vi "DPC LabView Controller.vi"() -> ()   [LabVIEW 2024]
doc: "This example program utilizes almost all VI's included in the AALBORG DPCM LabView Driver Library. In addition to the extended program example it provides access to the PI data Waveform Chart, User Defined Gas Mixture, Alarm Events and Process Information data logging settings and features of the DPM and DPC instruments. \nIf you have questions regarding VI's used in this example please refer to the \"AALBORG DPCM LabView Driver Library\" Manual (available on the AALBORG website and included in this driver library). If you still have questions please contact AALBORG at 845-770-3000 or info@aalborg.com"
uses:
  Examples/DPCM LabView Driver 2020_1v1/SubVI/Utilities/Control 1.ctl
  <vilib>/Utility/error.llb/Trim Whitespace One-Sided.vi
  Examples/DPCM LabView Driver 2020_1v1/SubVI/Utilities/Global.vi
panel:
  out "error out":errorcluster
  in  "Read Valve Output":bool
  in  "Read Register":bool
  out "Register Value":string
  in  "Reg. to read":u16 max=413
  in  "Log Register Values":bool
  out "Total GM:":u16
  in  "Gas mixture input":T1={"Ratio % 1"=0.0, "Enable # 1"=FALSE, "Ratio % 2"=0.0, "Enable # 2"=FALSE, "Ratio % 3"=0.0, "Enable # 3"=FALSE, "Ratio % 4"=0.0, "Enable # 4"=FALSE, "Ratio % 5"=0.0, "Enable # 5"=FALSE, "Mixture Gas 1"=0, "Mixture Gas 2"=0, "Mixture Gas 3"=0, "Mixture Gas 4"=0, "Mixture Gas 5"=0, "Create Mixture"=FALSE, "Mix. #"=200, "Mix. name"="MyMix1", "Completion\ntext"="", "Delete Mixture"=FALSE} caption="User Defined Gas Mixture input" {"Mix. #" min=200 max=219 step=1; "Mixture Gas 5" items=["Air", "Argon", "Carbon Dioxide", "Nitrogen", "Oxygen", "Helium", "Carbon Monoxide", "Ethylene", "Ethane", "n-Butane", "i-Butane", "Propane", "Deuterium", "Hydrogen", "Nitrous Oxide", "Methane", "Neon", "Krypton", "Sulfur Hexafluoride", "Xenon", "Acetylene", "25CO2/75Ar", "10CO2/90Ar", "8CO2/92Ar", "2CO2/98Ar", "75CO2/25Ar", "75He/25Ar", "25He/75Ar", "He A1025", "StargonCS", "95Ar/5CH4"]; "Mixture Gas 4" items=["Air", "Argon", "Carbon Dioxide", "Nitrogen", "Oxygen", "Helium", "Carbon Monoxide", "Ethylene", "Ethane", "n-Butane", "i-Butane", "Propane", "Deuterium", "Hydrogen", "Nitrous Oxide", "Methane", "Neon", "Krypton", "Sulfur Hexafluoride", "Xenon", "Acetylene", "25CO2/75Ar", "10CO2/90Ar", "8CO2/92Ar", "2CO2/98Ar", "75CO2/25Ar", "75He/25Ar", "25He/75Ar", "He A1025", "StargonCS", "95Ar/5CH4"]; "Mixture Gas 3" items=["Air", "Argon", "Carbon Dioxide", "Nitrogen", "Oxygen", "Helium", "Carbon Monoxide", "Ethylene", "Ethane", "n-Butane", "i-Butane", "Propane", "Deuterium", "Hydrogen", "Nitrous Oxide", "Methane", "Neon", "Krypton", "Sulfur Hexafluoride", "Xenon", "Acetylene", "25CO2/75Ar", "10CO2/90Ar", "8CO2/92Ar", "2CO2/98Ar", "75CO2/25Ar", "75He/25Ar", "25He/75Ar", "He A1025", "StargonCS", "95Ar/5CH4"]; "Mixture Gas 2" items=["Air", "Argon", "Carbon Dioxide", "Nitrogen", "Oxygen", "Helium", "Carbon Monoxide", "Ethylene", "Ethane", "n-Butane", "i-Butane", "Propane", "Deuterium", "Hydrogen", "Nitrous Oxide", "Methane", "Neon", "Krypton", "Sulfur Hexafluoride", "Xenon", "Acetylene", "25CO2/75Ar", "10CO2/90Ar", "8CO2/92Ar", "2CO2/98Ar", "75CO2/25Ar", "75He/25Ar", "25He/75Ar", "He A1025", "StargonCS", "95Ar/5CH4"]; "Mixture Gas 1" items=["Air", "Argon", "Carbon Dioxide", "Nitrogen", "Oxygen", "Helium", "Carbon Monoxide", "Ethylene", "Ethane", "n-Butane", "i-Butane", "Propane", "Deuterium", "Hydrogen", "Nitrous Oxide", "Methane", "Neon", "Krypton", "Sulfur Hexafluoride", "Xenon", "Acetylene", "25CO2/75Ar", "10CO2/90Ar", "8CO2/92Ar", "2CO2/98Ar", "75CO2/25Ar", "75He/25Ar", "25He/75Ar", "He A1025", "StargonCS", "95Ar/5CH4"]; "Ratio % 1" min=0.0 max=100.0 step=0.01; "Ratio % 2" min=0.0 max=100.0 step=0.01; "Ratio % 3" min=0.0 max=100.0 step=0.01; "Ratio % 4" min=0.0 max=100.0 step=0.01; "Ratio % 5" min=0.0 max=100.0 step=0.01}
  in  "AE Reset":bool
  in  "Alarm Events":T2={"AE Enable 0"=TRUE, "AE Enable 1"=TRUE, "AE Enable 2"=TRUE, "AE Enable 3"=TRUE, "AE Enable 4"=TRUE, "AE Enable 5"=TRUE, "AE Enable 6"=TRUE, "AE Enable 7"=TRUE, "AE Enable 8"=TRUE, "AE Enable 9"=TRUE, "AE Enable 10"=TRUE, "AE Enable 11"=TRUE, "AE Enable 12"=TRUE, "AE Enable 13"=TRUE, "AE Latch 0"=TRUE, "AE Latch 1"=TRUE, "AE Latch 2"=TRUE, "AE Latch 3"=TRUE, "AE Latch 4"=TRUE, "AE Latch 5"=TRUE, "AE Latch 6"=TRUE, "AE Latch 7"=TRUE, "AE Latch 8"=TRUE, "AE Latch 9"=TRUE, "AE Latch 10"=TRUE, "AE Latch 11"=TRUE, "AE Latch 12"=TRUE, "AE Latch 13"=TRUE, "AE Indicator 0"=FALSE, "AE Indicator 1"=FALSE, "AE Indicator 2"=FALSE, "AE Indicator 3"=FALSE, "AE Indicator 4"=FALSE, "AE Indicator 5"=FALSE, "AE Indicator 6"=FALSE, "AE Indicator 7"=FALSE, "AE Indicator 8"=FALSE, "AE Indicator 9"=FALSE, "AE Indicator 10"=FALSE, "AE Indicator 11"=FALSE, "AE Indicator 12"=FALSE, "AE Indicator 13"=FALSE}
  in  "PI Logging Options":T3={"Set Point"=TRUE, "Valve Counts"=FALSE, "Mass Flow"=TRUE, "Volumetric Flow"=TRUE, "Totalizer#1"=TRUE, "Totalizer#2"=TRUE, "Gas Temperature"=TRUE, "Gas Pressure"=TRUE, "Flow Alarm"=TRUE, "Temp. Alarm"=TRUE, "Pressure Alarm"=TRUE, "Alarm Events"=FALSE, "Diagnostic Events"=FALSE, "Selected Gas"=FALSE, "Log Data"=FALSE, "Include Header"=TRUE}
  in  "Chart: Adjust Scale":bool
  in  "Chart: AutoScale Chart":bool
  in  "Chart: Enable Graphic":bool
  in  "Chart: Pressure":bool
  in  "Chart: Temperature":bool
  in  "Chart: Set Point":bool
  in  "Chart: Volum Flow":bool
  in  "Chart: Mass Flow":bool
  out "Chart":cluster{dbl, dbl, dbl, dbl, dbl}(graph)={50.0, 50.24, 50.0, 23.8, 14.76}
  out "Wait Message":cluster{"Boolean":bool}
  in  "stop":bool
  out "Process Information":T4
  in  "Set Point Options":T5 {"Setpoint Value" min=0.0 max=0.0}
  in  "Analog Input":string(combo)
  in  "Analog Output":string(combo)
  in  "SS Relay Assignment":string(combo)
  in  "Measuring Units":T6
  in  "Update Time  [ms]":u32=150 min=100
  out "Measurem.\nper second":dbl format="%#.3g"
  in  "Selected Gas":string(combo)
  in  "Alarms":enum32{"Flow ", "Temp. ", "Pressure "}(tab)
  in  "Flow Alarm":T7 {"Power Up Delay [s]" min=0.0 max=3600.0 format="%#.0f"; "Action Delay [s]" min=0.0 max=3600.0 format="%#.0f"; "Low Alarm Limit" min=0.0 max=125.0 format="%#.1f"; "High Alarm Limit" min=0.0 max=125.0 format="%#.1f"}
  in  "Temperature Alarm":T8={"Enabled"=FALSE, "Status:"="", "High Temp. Alarm Limit"=253.1, "Low Temp. Alarm Limit"=0.0, "Temp. Alarm Latch"=FALSE, "Action Delay [s]"=0.0, "Power Up Delay [s]"=0.0} {"Power Up Delay [s]" min=0.0 max=3600.0 format="%#.0f"; "Action Delay [s]" min=0.0 max=3600.0 format="%#.0f"; "Low Temp. Alarm Limit" min=0.0 max=125.0 format="%#.1f"; "High Temp. Alarm Limit" min=253.1 max=343.1 format="%#.1f"}
  in  "Pressure Alarm":T9={"Enabled"=FALSE, "Status:"="", "High Pressure Alarm Limit"=253.1, "Low Pressure Alarm Limit"=0.0, "Pressure Alarm Latch"=FALSE, "Action Delay [s]"=0.0, "Power Up Delay [s]"=0.0} {"Power Up Delay [s]" min=0.0 max=3600.0 format="%#.0f"; "Action Delay [s]" min=0.0 max=3600.0 format="%#.0f"; "Low Pressure Alarm Limit" min=0.0 max=125.0 format="%#.1f"; "High Pressure Alarm Limit" min=253.1 max=343.1 format="%#.1f"}
  in  "Tab Control":T10(tab)
  in  "Totalizer #1 Options":T11 {"Power Up Delay [seconds]" min=0.0 max=3600.0 format="%#.0f"; "Auto Reset Delay [seconds]" min=0.0 max=3600.0 format="%#.0f"; "Current Volume" format="%#.2f"; "Action Volume" format="%#.2f"; "Start @ Flow" min=0.0 max=100.0 format="%#.2f"}
  in  "Totalizer #2 Options":T12 {"Current Volume" format="%#.2f"; "Action Volume" format="%#.2f"; "Start @ Flow" min=0.0 max=100.0 format="%#.1f"; "Power Up Delay [Seconds]" min=0.0 max=3600.0 format="%#.0f"; "Auto Reset Delay [Seconds]" min=0.0 max=3600.0 format="%#.0f"}
  in  "Pulse Output Options":T13={"Enabled"=FALSE, "Start @ Flow Rate"=0.0, "Unit Per Pulse"=0.0, "Pulse Unit"="", "Pulse Active Time [ms]"=25.0} {"Pulse Active Time [ms]" min=25.0 max=3276.0 format="%#.0f"; "Unit Per Pulse" format="%#.2f"; "Start @ Flow Rate" min=0.0 max=100.0 format="%#.1f"}
  out "Device Information":T14
  in  "Serial Configuration":T16={"Baud Rate"=9600, "Serial Port #"="COM1", "RS-485"=FALSE, " Address"=17} {"Address" min=1 format="%2x"; "Baud Rate" items=["300"=300, "600"=600, "1200"=1200, "2400"=2400, "4800"=4800, "9600"=9600, "19200"=19200, "38400"=38400]}
  # "Timing Options"
  # "(will require longer update time)"
  # "Before changing Analog Input or Output mode make sure proper equipment is connected to the corresponding pins on the interface connector!"
  # "E/D"
  # "Latch"
  # "Register Values"
  # "AALBORG INSTRUMENTS"
  # "& CONTROLS INC."
  # "Possible Issues\n• When communicating with instruments over RS-485 interface and \"Read Valve Output\" check box is selected some times it is possible to get \"Communication Error\" message when low \"Baud Rate\" settings are selected. In this case use 19200 or higher \"Baud Rate\" settings to be able to faster transfer long data frames to and from the instrument.\n\n• Do not use \"Update Time\" settings with values below 50 ms. Doing so especially with low \"Baud Rate\" settings may result in communication error."
  # "High Flow Alarm"
  # "Low Flow Alarm"
  # "Flow between H & L"
  # "Totalizer#1 > Limit"
  # "Totalizer#2 > Limit"
  # "High Press. Alarm"
  # "Low Pressure Alarm"
  # "Press. between H&L"
  # "High Temp. Alarm"
  # "Low Temp. Alarm"
  # "Temp. Between H&L"
  # "Pulse Output > Limit"
  # "Password Event"
  # "Power On Event"
  # "Altering options will start a new log"
  # "(The data file will be open in the folder containing the VI)"
  # "Populating VI with instrument information. Standby..."
  # "Alarm"
  # "%FS"
  # "%FS"
  # "K  [253.1 - 343.1K]"
  # "K [253.0 - 343.0K]"
  # "PSIA  [0.1-100 PSIA]"
  # "PSIA [0.0-99.9 PSIA]"
  # "%FS"
  # "%FS"
  # "%FS"
  # "/Pulse"
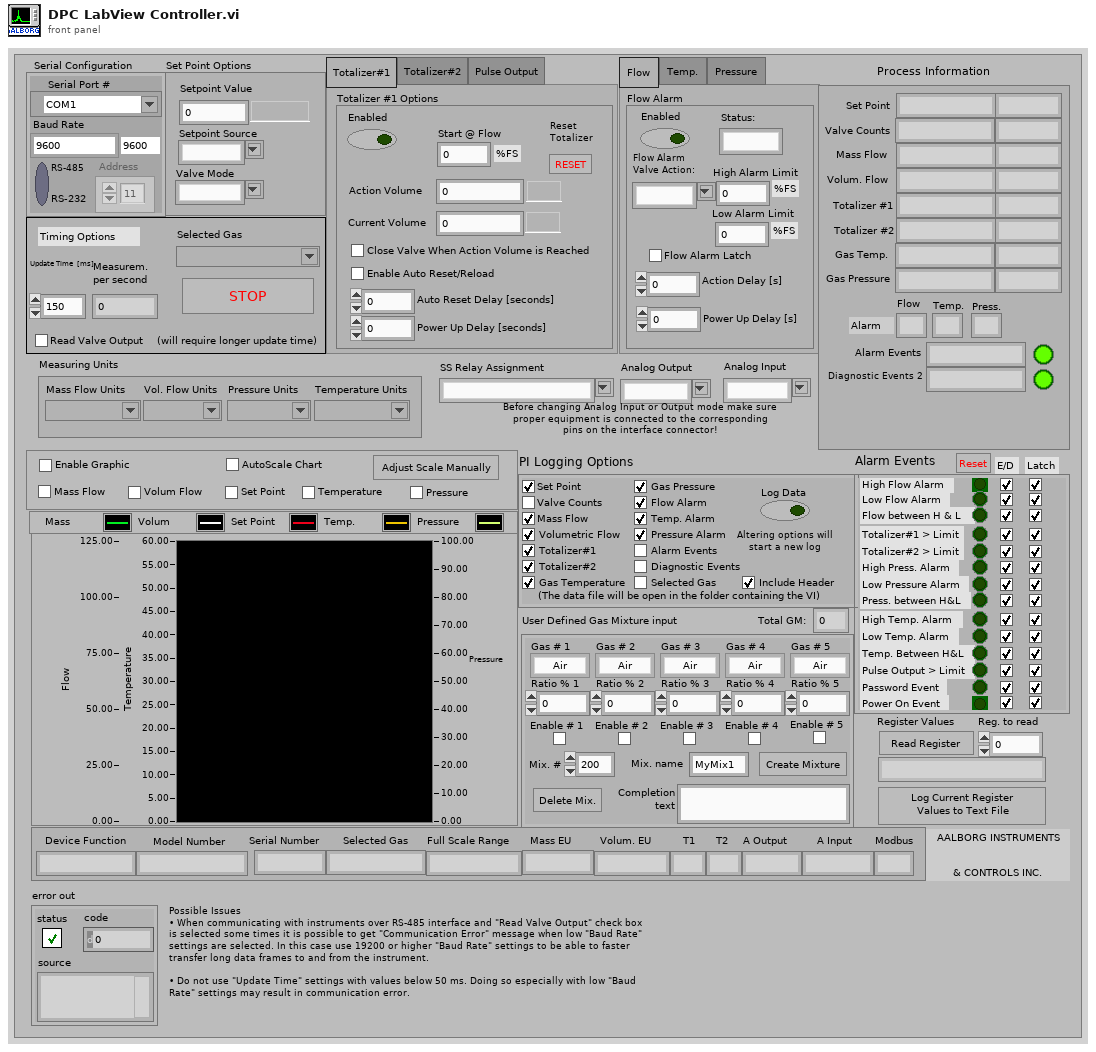
[diagram p1: front panel]
types:
  T1 = cluster{"Ratio % 1":dbl, "Enable # 1":bool, "Ratio % 2":dbl, "Enable # 2":bool, "Ratio % 3":dbl, "Enable # 3":bool, "Ratio % 4":dbl, "Enable # 4":bool, "Ratio % 5":dbl, "Enable # 5":bool, "Mixture Gas 1":u16, "Mixture Gas 2":u16, "Mixture Gas 3":u16, "Mixture Gas 4":u16, "Mixture Gas 5":u16, "Create Mixture":bool, "Mix. #":u16, "Mix. name":string, "Completion\ntext":string, "Delete Mixture":bool}
  T2 = cluster{"AE Enable 0":bool, "AE Enable 1":bool, "AE Enable 2":bool, "AE Enable 3":bool, "AE Enable 4":bool, "AE Enable 5":bool, "AE Enable 6":bool, "AE Enable 7":bool, "AE Enable 8":bool, "AE Enable 9":bool, "AE Enable 10":bool, "AE Enable 11":bool, "AE Enable 12":bool, "AE Enable 13":bool, "AE Latch 0":bool, "AE Latch 1":bool, "AE Latch 2":bool, "AE Latch 3":bool, "AE Latch 4":bool, "AE Latch 5":bool, "AE Latch 6":bool, "AE Latch 7":bool, "AE Latch 8":bool, "AE Latch 9":bool, "AE Latch 10":bool, "AE Latch 11":bool, "AE Latch 12":bool, "AE Latch 13":bool, "AE Indicator 0":bool, "AE Indicator 1":bool, "AE Indicator 2":bool, "AE Indicator 3":bool, "AE Indicator 4":bool, "AE Indicator 5":bool, "AE Indicator 6":bool, "AE Indicator 7":bool, "AE Indicator 8":bool, "AE Indicator 9":bool, "AE Indicator 10":bool, "AE Indicator 11":bool, "AE Indicator 12":bool, "AE Indicator 13":bool}
  T3 = cluster{"Set Point":bool, "Valve Counts":bool, "Mass Flow":bool, "Volumetric Flow":bool, "Totalizer#1":bool, "Totalizer#2":bool, "Gas Temperature":bool, "Gas Pressure":bool, "Flow Alarm":bool, "Temp. Alarm":bool, "Pressure Alarm":bool, "Alarm Events":bool, "Diagnostic Events":bool, "Selected Gas":bool, "Log Data":bool, "Include Header":bool}
  T4 = cluster{"Mass Flow":string, "Volum. Flow":string, "Totalizer #1":string, "Totalizer #2":string, "Gas Temp.":string, "Gas Pressure":string, "Flow":string, "Press.":string, "Temp.":string, "Alarm Events":string, "Diagnostic Events 2":string, "Set Point":string, "Valve Counts":string, "Alarm Ind":bool, "Diagnostic Ind":bool, "SP Units":string, "Valve Counts Units":string, "Mass Flow Units":string, "Vol Flow Units":string, "Total1 Vol Units":string, "Total2 Vol Units":string, "Gas Temp Units":string, "Gas Press Units":string}
  T5 = cluster{"Setpoint Value":dbl, "Mass Flow EU 2":string, "Setpoint Source":string, "Valve Mode":string}
  T6 = cluster{"Mass Flow Units":string, "Vol. Flow Units":string, "Pressure Units":string, "Temperature Units":string}
  T7 = cluster{"Enabled":bool, "Status:":string, "High Alarm Limit":dbl, "Low Alarm Limit":dbl, "Flow Alarm Latch":bool, "Action Delay [s]":dbl, "Power Up Delay [s]":dbl, "Flow Alarm Valve Action:":string}
  T8 = cluster{"Enabled":bool, "Status:":string, "High Temp. Alarm Limit":dbl, "Low Temp. Alarm Limit":dbl, "Temp. Alarm Latch":bool, "Action Delay [s]":dbl, "Power Up Delay [s]":dbl}
  T9 = cluster{"Enabled":bool, "Status:":string, "High Pressure Alarm Limit":dbl, "Low Pressure Alarm Limit":dbl, "Pressure Alarm Latch":bool, "Action Delay [s]":dbl, "Power Up Delay [s]":dbl}
  T10 = enum32{"Totalizer#1", "Totalizer#2", "Pulse Output"}
  T11 = cluster{"Enabled":bool, "Start @ Flow":dbl, "Action Volume":dbl, "Total EU 1":string, "Current Volume":dbl, "Total EU 2":string, "Close Valve When Action Volume is Reached":bool, "Enable Auto Reset/Reload":bool, "Auto Reset Delay [seconds]":dbl, "Power Up Delay [seconds] ":dbl, "Reset Totalizer":bool}
  T12 = cluster{"Enabled":bool, "Start @ Flow":dbl, "Action Volume":dbl, "Total EU 1":string, "Current Volume":dbl, "Total EU 2":string, "Close Valve When Action Volume is Reached":bool, "Enable Auto Reset/Reload":bool, "Auto Reset Delay [Seconds]":dbl, "Power Up Delay [Seconds] ":dbl, "Reset Totalizer":bool}
  T13 = cluster{"Enabled":bool, "Start @ Flow Rate":dbl, "Unit Per Pulse":dbl, "Pulse Unit":string, "Pulse Active Time [ms]":dbl}
  T14 = cluster{"Device Function":string, "Model Number":string, "Serial Number":string, "Selected Gas":string, "Full Scale Range":string, "Mass EU":string, "Volum. EU":string, "    T1 ":string, "   T2 ":string, "A Output":string, "A Input":string, "Modbus":string}
  T15 = typedef "Control 1.ctl" = u32
  T16 = cluster{"Baud Rate":T15, "Serial Port #":refnum<visa-resource-name>, "RS-485":bool, " Address":u8}
  T17 = cluster{"Mass Flow":bool, "Volum Flow":bool, "Set Point":bool, "Temperature":bool, "Pressure":bool, "AutoScale Chart":bool}
  T18 = cluster{"Enabled":string, "High Alarm Limit":string, "Low Alarm Limit":string, "Action Delay":string, "Latch Mode":string, "Power Up Delay":string}
  T19 = cluster{"Enabled":bool, "Start @ Flow":dbl, "Limit Volume":dbl, "Total EU 1":string, "Current Volume":dbl, "Total EU 2":string, "Close Valve When Limit Volume is Reached":bool, "Enable Auto Reset/Reload":bool, "Auto Reset Delay [Seconds]":dbl, "Power Up Delay [Seconds] ":dbl, "Reset Totalizer":bool}
  T20 = cluster{"Enabled":bool, "Start @ Flow":dbl, "Limit Volume":dbl, "Total EU 1":string, "Current Volume":dbl, "Total EU 2":string, "Close Valve When Limit Volume is Reached":bool, "Enable Auto Reset/Reload":bool, "Auto Reset Delay [seconds]":dbl, "Power Up Delay [seconds] ":dbl, "Reset Totalizer":bool}
  T21 = cluster{"Enabled":enum8{"Enabled", "Disabled", "Disabled and Grayed Out"}, "Disabled and Grayed Out":enum8{"Enabled", "Disabled", "Disabled and Grayed Out"}}
  T22 = enum16{"open", "replace", "create", "open or create", "replace or create", "replace or create with confirmation"}
  T23 = cluster{"Mass Flow":string, "Valve Counts":string, "Volumetric Flow":string, "Totalizer":string, "Temperature":string, "Pressure":string}
  T24 = cluster{"Gas # 1":u16, "Mix % 1":dbl, "Include # 1":bool, "Gas # 2":u16, "Mix % 2":dbl, "Include # 2":bool, "Gas # 3":u16, "Mix % 3":dbl, "Include # 3":bool, "Gas # 4":u16, "Mix % 4":dbl, "Include # 4":bool, "Gas # 5":u16, "Mix % 5":dbl, "Include # 5":bool}
  T25 = cluster{"Model Number":string, "Serial Number":string, "Gas Name":string, "FS Range":string, "Mass Flow EU":string, "Volumetric Flow EU":string, "Modbus":string, "Totalizer#1 Mode":string, "Totalizer#2 Mode":string, "Analog Output":string, "Pressure EU":string, "Temperature EU":string, "Device Function":string}
  T26 = enum8{"Enabled", "Disabled", "Disabled and Grayed Out"}
  T27 = typedef "LVComboBoxStrsAndValuesArrayTypeDef.ctl" = cluster{"String":string, "Value":string}[]
  T28 = cluster{"Setpoint Source Out":string, "Valve Mode Out":string, dbl}
  T29 = cluster{"Tot. Mode":string, "Start @ Flow":string, "Limit Volume":string, "Power Up Delay":string, "Auto Reset Mode":string, "Auto Reset Delay":string}
  T30 = cluster{"Enabled":string, "Start @ Flow":string, "Unit Per Pulse":string, "Pulse Active Time":string}
  T31 = cluster{"string array[0]":string, "string array[1]":string, "string array[2]":string, "string array[3]":string, "string array[4]":string, "string array[5]":string, "string array[6]":string, "string array[7]":string, "string array[8]":string, "string array[9]":string, "string array[10]":string}
  T32 = enum16{"Left Button", "Center Button", "Right Button", "Window Close"}
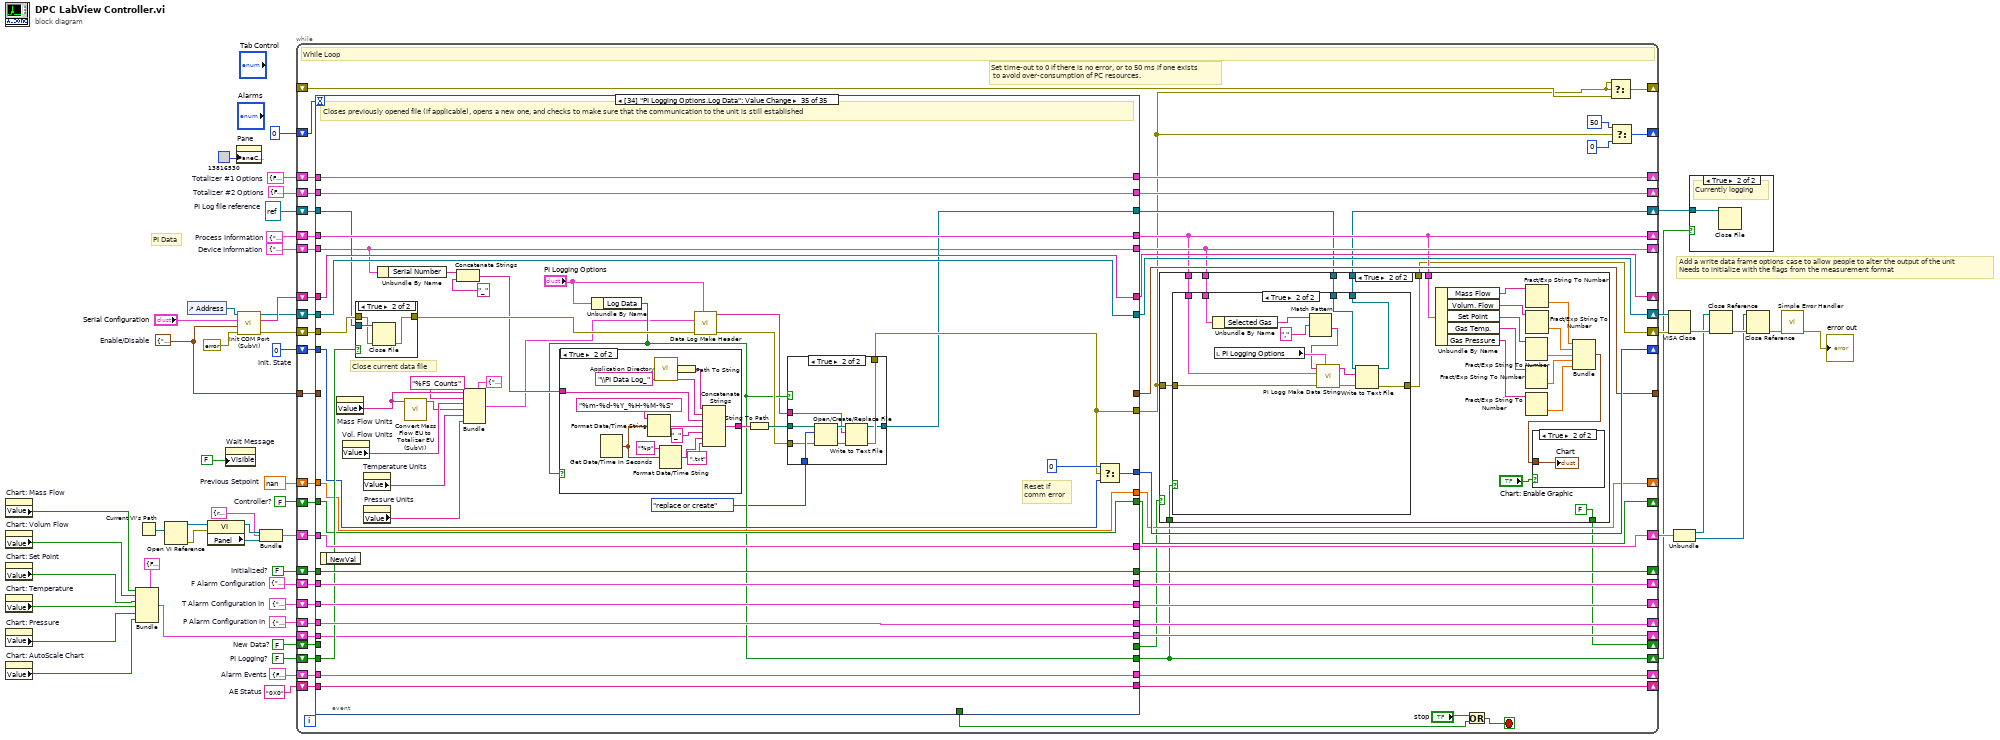
[diagram p0: block diagram]
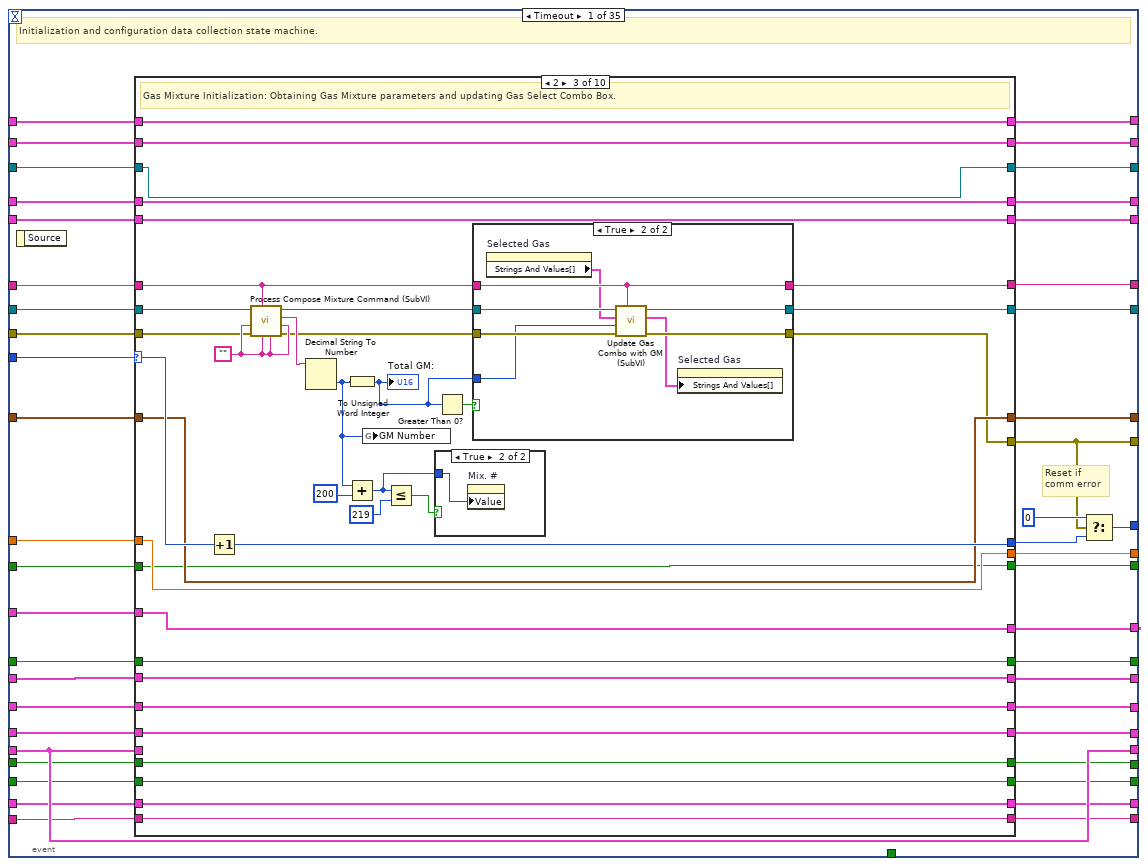
[diagram p6: hidden frame]
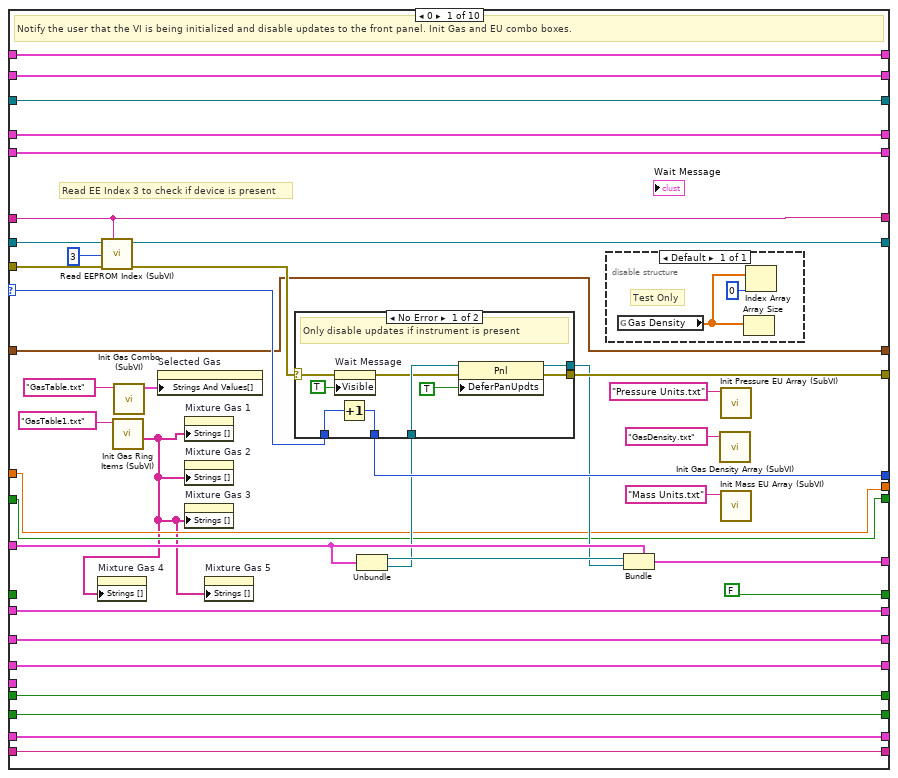
[diagram p7: hidden frame]
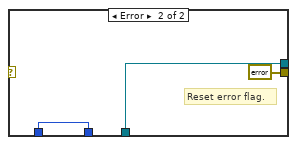
[diagram p8: hidden frame]
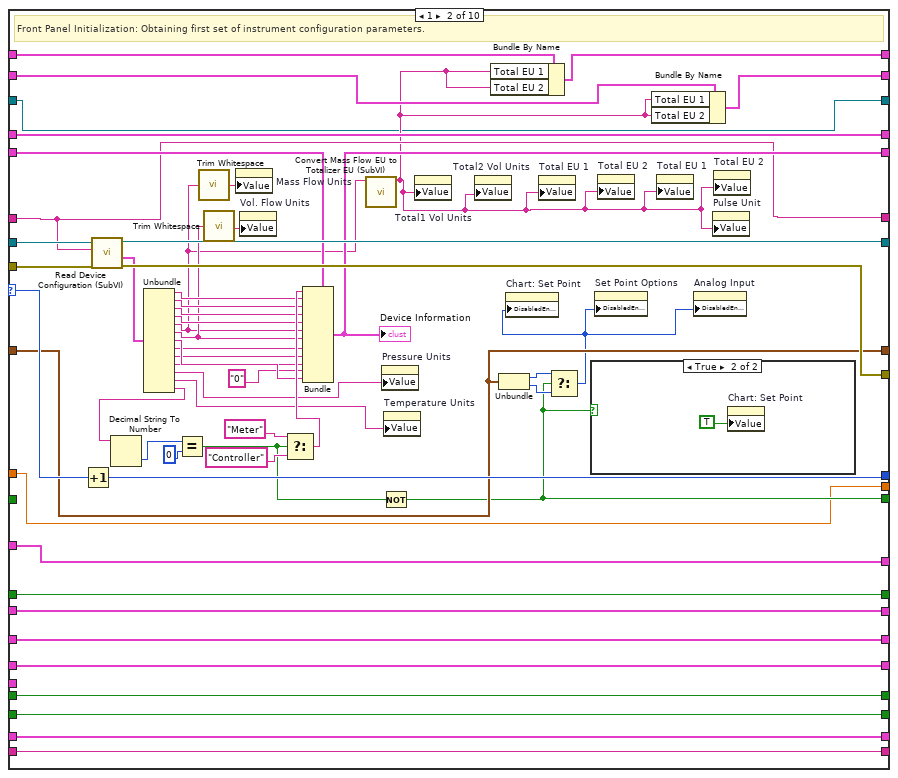
[diagram p9: hidden frame]
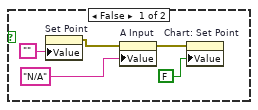
[diagram p10: hidden frame]
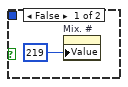
[diagram p11: hidden frame]
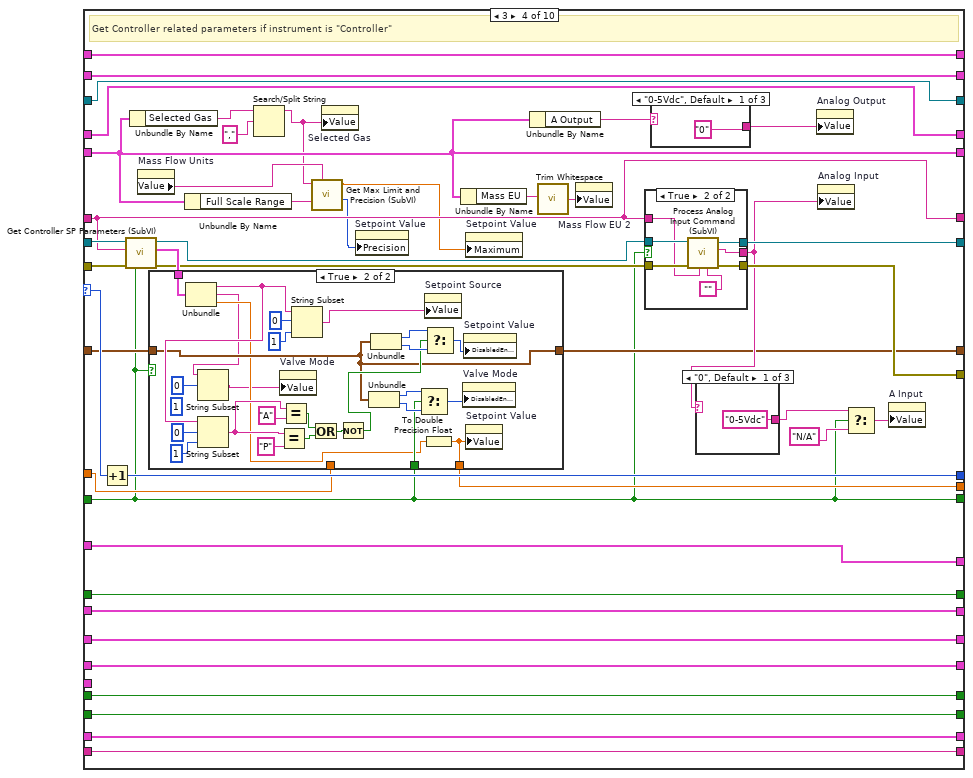
[diagram p13: hidden frame]
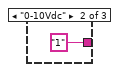
[diagram p15: hidden frame]
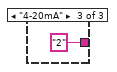
[diagram p16: hidden frame]
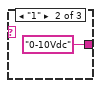
[diagram p17: hidden frame]
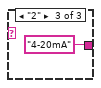
[diagram p18: hidden frame]
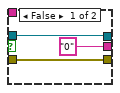
[diagram p19: hidden frame]
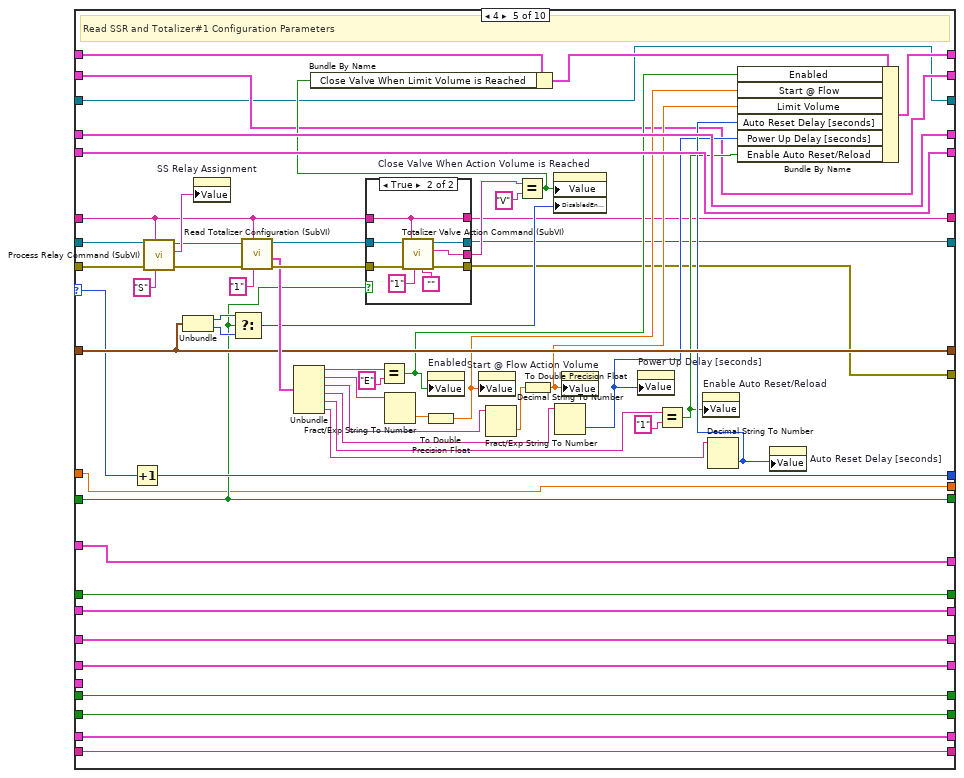
[diagram p20: hidden frame]
diagram:
  w2 = "0X0"  # AE Status
  w3 = T2 {"AE Enable 0"=FALSE, "AE Enable 1"=FALSE, "AE Enable 2"=FALSE, "AE Enable 3"=FALSE, "AE Enable 4"=FALSE, "AE Enable 5"=FALSE, "AE Enable 6"=FALSE, "AE Enable 7"=FALSE, "AE Enable 8"=FALSE, "AE Enable 9"=FALSE, "AE Enable 10"=FALSE, "AE Enable 11"=FALSE, "AE Enable 12"=FALSE, "AE Enable 13"=FALSE, "AE Latch 0"=FALSE, "AE Latch 1"=FALSE, "AE Latch 2"=FALSE, "AE Latch 3"=FALSE, "AE Latch 4"=FALSE, "AE Latch 5"=FALSE, "AE Latch 6"=FALSE, "AE Latch 7"=FALSE, "AE Latch 8"=FALSE, "AE Latch 9"=FALSE, "AE Latch 10"=FALSE, "AE Latch 11"=FALSE, "AE Latch 12"=FALSE, "AE Latch 13"=FALSE, "AE Indicator 0"=FALSE, "AE Indicator 1"=FALSE, "AE Indicator 2"=FALSE, "AE Indicator 3"=FALSE, "AE Indicator 4"=FALSE, "AE Indicator 5"=FALSE, "AE Indicator 6"=FALSE, "AE Indicator 7"=FALSE, "AE Indicator 8"=FALSE, "AE Indicator 9"=FALSE, "AE Indicator 10"=FALSE, "AE Indicator 11"=FALSE, "AE Indicator 12"=FALSE, "AE Indicator 13"=FALSE}  # Alarm Events
  w6 = FALSE  # PI Logging?
  w7 = refnum<file> refnum  # PI Log file reference
  w8 = FALSE  # New Data?
  w17 = T18 {"Enabled"="", "High Alarm Limit"="", "Low Alarm Limit"="", "Action Delay"="", "Latch Mode"="", "Power Up Delay"=""}  # P Alarm Configuration In
  w18 = T18 {"Enabled"="", "High Alarm Limit"="", "Low Alarm Limit"="", "Action Delay"="", "Latch Mode"="", "Power Up Delay"=""}  # T Alarm Configuration In
  w19 = T18 {"Enabled"="D", "High Alarm Limit"="54.00", "Low Alarm Limit"="7.00", "Action Delay"="1", "Latch Mode"="0", "Power Up Delay"="10"}  # F Alarm Configuration
  w20 = T19 {"Enabled"=FALSE, "Start @ Flow"=2.0, "Limit Volume"=0.0, "Total EU 1"="  %s  ", "Current Volume"=0.0, "Total EU 2"="  %s  ", "Close Valve When Limit Volume is Reached"=FALSE, "Enable Auto Reset/Reload"=FALSE, "Auto Reset Delay [Seconds]"=1.0, "Power Up Delay [Seconds] "=10.0, "Reset Totalizer"=FALSE}  # Totalizer #2 Options
  w21 = T20 {"Enabled"=FALSE, "Start @ Flow"=2.0, "Limit Volume"=0.0, "Total EU 1"="  %s  ", "Current Volume"=131.62, "Total EU 2"="  %s  ", "Close Valve When Limit Volume is Reached"=FALSE, "Enable Auto Reset/Reload"=FALSE, "Auto Reset Delay [seconds]"=2.0, "Power Up Delay [seconds] "=8.0, "Reset Totalizer"=FALSE}  # Totalizer #1 Options
  w22 = T14 {"Device Function"="Controller", "Model Number"="DPC17A-VAL6-A2", "Serial Number"="999001-2", "Selected Gas"="0,Air", "Full Scale Range"="0.00050 sl/min", "Mass EU"="%FS", "Volum. EU"=" %FS  ", "    T1 "="D", "   T2 "="D", "A Output"="0-5Vdc", "A Input"="0-5Vdc", "Modbus"="Yes"}  # Device Information
  w23 = T4 {"Mass Flow"="25.00", "Volum. Flow"="25.24", "Totalizer #1"="0.00", "Totalizer #2"="0.00", "Gas Temp."="23.72", "Gas Pressure"="14.68", "Flow"="D", "Press."="D", "Temp."="D", "Alarm Events"="0x0", "Diagnostic Events 2"="0x0", "Set Point"="  0.125", "Valve Counts"="N/A", "Alarm Ind"=FALSE, "Diagnostic Ind"=FALSE, "SP Units"="", "Valve Counts Units"="Counts", "Mass Flow Units"="", "Vol Flow Units"="", "Total1 Vol Units"="%s", "Total2 Vol Units"="%s", "Gas Temp Units"="C", "Gas Press Units"="PSIA"}  # Process Information
  w25 = nan  # Previous Setpoint
  w38 = FALSE  # Controller?
  w39 = FALSE  # Initialized?
  w47 = 0  # Init. State
  w28 = T21 {"Enabled"=enum."Enabled", "Disabled and Grayed Out"=enum."Disabled and Grayed Out"}  # Enable/Disable
  # "Add a write data frame options case to allow people to alter the output of the unit\nNeeds to initialize with the flags from the measurement format"
  # "PI Data"
  n1 = property on="Chart: Mass Flow" class="Bool (strict)"() -> ("Value"=w16:bool)  [unwired: 2 in, 2 out]
  n2 = property on="Chart: Volum Flow" class="Bool (strict)"() -> ("Value"=w15:bool)  [unwired: 2 in, 2 out]
  n3 = property on="Chart: Set Point" class="Bool (strict)"() -> ("Value"=w14:bool)  [unwired: 2 in, 2 out]
  n4 = property on="Chart: Temperature" class="Bool (strict)"() -> ("Value"=w13:bool)  [unwired: 2 in, 2 out]
  n5 = property on="Chart: Pressure" class="Bool (strict)"() -> ("Value"=w12:bool)  [unwired: 2 in, 2 out]
  n6 = property on="Chart: AutoScale Chart" class="Bool (strict)"() -> ("Value"=w11:bool)  [unwired: 2 in, 2 out]
  n7 = Bundle(cluster=T17 {"Mass Flow"=FALSE, "Volum Flow"=FALSE, "Set Point"=FALSE, "Temperature"=FALSE, "Pressure"=FALSE, "AutoScale Chart"=FALSE} ("Graphing enables"), "Mass Flow"=w16, "Volum Flow"=w15, "Set Point"=w14, "Temperature"=w13, "Pressure"=w12, "AutoScale Chart"=w11) -> (w9:T17)
  n8 = Current VI's Path() -> (path=w45:path)
  n9 = Open VI Reference(vi path=w45) -> (vi reference=w44:refnum<vi>, error out=w42:errorcluster)  [unwired: 5 in]
  n10 = control-ref of="Address"() -> (w50:refnum<vi>)
  n11 = property class="VI"(reference=w44, error in=w42) -> (reference out=w41:refnum<vi>, "Panel"=w43:refnum<vi>)  [unwired: 1 out]
  n12 = property on="Wait Message" class="Clust (strict)"("Visible"=FALSE) -> ()  [unwired: 2 in, 2 out]
  n13 = property on="Pane" class="Pane"("PaneColor"=u32 13816530 ("Pane Color")) -> ()  [unwired: 2 in, 2 out]
  n14 = call "Init COM Port (SubVI).vi"("error in (no error)"=errorcluster {"status"=FALSE, "code"=0, "source"=""}, "Enable/Disable"=w28, "Serial Configuration"="Serial Configuration", "Digital in"=w50) -> ("error out"=w49:errorcluster, "Address String"=w48:string, "VISA Refnum out"=w27:refnum<visa-resource-name>)  [unwired: 5 in]
  n15 = Bundle(cluster=cluster{refnum<vi>, "Panel":refnum<vi>} {refnum, "Panel"=refnum}, w41, "Panel"=w43) -> (w40:cluster{refnum<vi>, "Panel":refnum<vi>})
  n16 = while {
    shift-right: [w105] -> w30
    shift-left: w27 -> [w88]
    shift-right: [w89] -> w31
    shift-left: w40 -> [w104]
    shift-right: [w100] -> _
    shift-left: w47 -> [w108]
    shift-right: [w60] -> w29
    shift-left: w49 -> [w107]
    shift-right: [w99] -> _
    shift-left: w39 -> [w103]
    shift-right: [w101] -> _
    shift-left: w38 -> [w102]
    shift-right: [w95] -> _
    shift-left: 0 -> [w98]
    shift-right: [w94] -> _
    shift-left: _ -> [w93]
    shift-right: [w62] -> _
    shift-left: w22 -> [w92]
    shift-right: [w84] -> _
    shift-left: w48 -> [w106]
    shift-right: [w61] -> _
    shift-left: w23 -> [w83]
    shift-right: [w81] -> _
    shift-left: w25 -> [w82]
    tunnel: w28 -> [w91]
    tunnel: [w90] -> _
    shift-right: [w79] -> _
    shift-left: w21 -> [w80]
    shift-right: [w77] -> _
    shift-left: w20 -> [w78]
    shift-right: [w76] -> _
    shift-left: w19 -> [w75]
    shift-right: [w73] -> _
    shift-left: w18 -> [w74]
    shift-right: [w71] -> _
    shift-left: w17 -> [w72]
    shift-right: [w69] -> _
    shift-left: w9 -> [w70]
    shift-right: [w67] -> _
    shift-left: w8 -> [w68]
    shift-right: [w58] -> w5
    shift-left: w7 -> [w65]
    shift-right: [w63] -> w4
    shift-left: w6 -> [w64]
    shift-right: [w56] -> _
    shift-left: w3 -> [w57]
    shift-right: [w54] -> _
    shift-left: w2 -> [w55]
    stop <- w85 stop-if-true
    # "Set time-out to 0 if there is no error, or to 50 ms if one exists\n to avoid over-consumption of PC resources."
    # "While Loop"
    n17 = event shown="[34] \"PI Logging Options.Log Data\": Value Change" {
      selector: _ -> [_ _ _ _ _ _ _ _ _ _ _ _ _ _ _ _ _ _ _ _ _ _ _ _ _ _ _ _ _ _ _ _ _ _ _]
      dyn-events: _ -> [_ _ _ _ _ _ _ _ _ _ _ _ _ _ _ _ _ _ _ _ _ _ _ _ _ _ _ _ _ _ _ _ _ _ _]
      timeout: w98 -> [_ _ _ _ _ _ _ _ _ _ _ _ _ _ _ _ _ _ _ _ _ _ _ _ _ _ _ _ _ _ _ _ _ _ _]
      tunnel: w108 -> [w192 _ _ _ _ _ w1026 w1084 w1175 w1226 w1319 w1372 w1450 w1526 w1581 w1611 w1643 w1671 w1730 w1759 w1796 w1833 w1872 w1983 w2094 w2167 w2298 w2411 w2530 w2570 w2596 w2638 w2672 w2747 w2819]
      tunnel: w107 -> [w191 w927 w947 w962 w982 w1005 w1044 w1092 w1188 w1237 w1294 w1381 w1454 w1530 w1585 w1602 w1634 w1660 w1721 w1751 w1804 w1841 w1879 w1990 w2101 w2174 w2305 w2418 w2511 w2553 w2583 w2625 w2654 w2731 w2829]
      tunnel: w106 -> [w190 _ _ _ _ _ w1037 w1089 w1187 w1232 w1322 w1376 w1448 w1525 w1580 w1601 w1637 w1662 w1720 w1748 w1802 w1839 w1877 w1988 w2099 w2172 w2303 w2416 w2508 w2552 w2578 w2621 w2641 w2726 w2831]
      tunnel: [w179 _ 0 ("Initialization Constant") 0 ("Initialization Constant") 0 ("Initialization Constant") 0 ("Initialization Constant") w1027 w1085 w1177 w1234 w1323 w1378 w1451 w1527 w1583 w1612 w1644 w1672 w1731 w1760 w1798 w1835 w1874 w1985 w2096 w2169 w2300 w2413 w2531 w2571 w2597 w2639 w2673 w2748 w2840] -> w100
      tunnel: [w180 w927 w938 w961 w981 w1004 w1028 w1086 w1176 w1235 w1292 w1379 w1452 w1528 w1582 w1603 w1634 w1659 w1724 w1750 w1797 w1834 w1873 w1984 w2095 w2168 w2299 w2412 w2510 w2554 w2581 w2623 w2642 w2727 w2822] -> w53
      tunnel: [w189 w928 w939 w959 w980 w1003 w1038 w1093 w1189 w1236 w1324 w1380 w1453 w1529 w1586 w1604 w1635 w1665 w1723 w1749 w1803 w1840 w1878 w1989 w2100 w2173 w2304 w2417 w2513 w2557 w2582 w2624 w2643 w2728 w2830] -> w105
      tunnel: [w187 w925 w933 w952 w974 w997 w1032 w1081 w1172 w1227 w1320 w1369 w1444 w1520 w1576 w1608 w1640 w1668 w1727 w1757 w1790 w1827 w1866 w1977 w2088 w2162 w2293 w2406 w2526 w2565 w2592 w2634 w2667 w2744 w2837] -> w89
      tunnel: w104 -> [w188 w925 w933 w952 w974 w997 w1032 w1081 w1172 w1227 w1320 w1369 w1444 w1520 w1576 w1608 w1640 w1668 w1727 w1757 w1790 w1827 w1866 w1977 w2088 w2162 w2293 w2406 w2526 w2565 w2592 w2634 w2667 w2744 w2837]
      tunnel: w103 -> [w186 w924 w932 w951 w973 w996 w1031 w1080 w1171 w1228 w1321 w1368 w1443 w1519 w1575 w1607 w1639 w1667 w1726 w1756 w1789 w1826 w1865 w1976 w2087 w2161 w2292 w2405 w2525 w2564 w2591 w2633 w2666 w2743 w2836]
      tunnel: [w185 w924 w932 w951 w973 w996 w1031 w1080 w1171 w1228 w1321 w1368 w1443 w1519 w1575 w1607 w1639 w1667 w1726 w1756 w1789 w1826 w1865 w1976 w2087 w2161 w2292 w2405 w2525 w2564 w2591 w2633 w2666 w2743 w2836] -> w99
      tunnel: w102 -> [w184 w926 w934 w953 w975 w998 w1033 w1058 w1173 w1224 w1317 w1370 w1442 w1533 w1577 w1609 w1641 w1669 w1728 w1747 w1791 w1828 w1867 w1978 w2089 w2156 w2288 w2401 w2523 w2562 w2589 w2631 w2664 w2741 w2821]
      tunnel: [w183 w926 w934 w953 w975 w998 w1033 w1058 w1173 w1224 w1317 w1370 w1442 w1533 w1577 w1609 w1641 w1669 w1728 w1747 w1791 w1828 w1867 w1978 w2089 w2156 w2288 w2401 w2523 w2562 w2589 w2631 w2664 w2741 w2821] -> w101
      tunnel: [w178 w929 w949 w955 w977 w1000 w1034 w1071 w1182 w1219 w1315 w1361 w1445 w1522 w1574 w1598 w1636 w1663 w1716 w1753 w1793 w1830 w1869 w1980 w2091 w2164 w2295 w2408 w2528 w2567 w2580 w2622 w2669 w2723 w2802] -> w62
      tunnel: w92 -> [w177 w929 w949 w955 w977 w1000 w1034 w1078 w1183 w1219 w1315 w1361 w1445 w1522 w1571 w1598 w1636 w1663 w1717 w1754 w1793 w1830 w1869 w1980 w2091 w2164 w2295 w2408 w2528 w2567 w2580 w2622 w2669 w2723 w2802]
      tunnel: w91 -> [w176 _ w940 _ w984 w1007 _ _ _ _ _ _ w1441 _ _ _ _ _ _ _ _ _ _ _ _ _ _ _ _ _ _ _ _ _ _]
      tunnel: [w175 _ _ _ _ _ _ _ _ _ _ _ _ _ _ _ _ _ _ _ _ _ _ _ _ _ _ _ _ _ _ _ _ _ _] -> w90
      tunnel: w88 -> [w174 w928 w948 w960 w983 w1006 w1045 w1094 w1190 w1238 w1324 w1382 w1455 w1531 w1587 w1605 w1635 w1665 w1722 w1752 w1805 w1842 w1880 w1991 w2102 w2175 w2306 w2419 w2512 w2556 w2584 w2626 w2655 w2732 w2830]
      tunnel: [_ w923 _ _ _ _ _ _ _ _ _ _ _ _ _ _ _ _ _ _ _ _ _ _ _ _ _ _ _ _ _ _ _ _ _] -> w86
      tunnel: [w173 _ w937 _ w979 w1002 w1037 w1089 w1179 w1231 w1322 w1375 w1447 w1524 w1580 w1601 w1637 w1662 w1720 w1746 w1800 w1837 w1876 w1987 w2098 w2171 w2302 w2415 w2509 w2552 w2578 w2621 w2641 w2726 w2831] -> w84
      tunnel: [w172 w922 w950 w956 w978 w1001 w1035 w1067 w1180 w1222 w1316 w1362 w1438 w1523 w1569 w1606 w1638 w1666 w1725 w1755 w1794 w1831 w1870 w1981 w2092 w2165 w2296 w2409 w2519 w2568 w2594 w2636 w2670 w2724 w2838] -> w61
      tunnel: w83 -> [w171 w922 w950 w956 w978 w1001 w1035 w1083 w1181 w1229 w1316 w1373 w1439 w1523 w1569 w1606 w1638 w1666 w1725 w1755 w1794 w1831 w1870 w1981 w2092 w2165 w2296 w2409 w2519 w2568 w2594 w2636 w2670 w2724 w2838]
      tunnel: w82 -> [w170 w921 w935 w954 w976 w999 w1046 w1079 w1174 w1225 w1318 w1371 w1436 w1521 w1578 w1610 w1642 w1670 w1729 w1758 w1792 w1829 w1868 w1979 w2090 w2163 w2294 w2407 w2527 w2566 w2593 w2635 w2668 w2745 w2820]
      tunnel: [w169 w921 w935 w954 w976 w999 w1036 w1057 w1174 w1225 w1318 w1371 w1437 w1521 w1578 w1610 w1642 w1670 w1729 w1758 w1792 w1829 w1868 w1979 w2090 w2163 w2294 w2407 w2527 w2566 w2593 w2635 w2668 w2745 w2820] -> w81
      tunnel: w80 -> [w168 _ _ _ _ _ w1021 w1061 w1168 w1214 w1289 w1358 w1433 w1516 w1564 w1595 w1621 w1653 w1712 w1743 w1795 w1832 w1871 w1982 w2093 w2166 w2297 w2410 w2529 w2569 w2595 w2637 w2671 w2746 w2839]
      tunnel: [w167 _ _ _ _ _ w1021 w1061 w1168 w1214 w1289 w1358 w1433 w1516 w1564 w1595 w1621 w1653 w1712 w1743 w1795 w1832 w1871 w1982 w2093 w2166 w2297 w2410 w2529 w2569 w2595 w2637 w2671 w2746 w2839] -> w79
      tunnel: w78 -> [w166 _ _ _ _ _ w1014 w1062 w1167 w1213 w1288 w1357 w1432 w1515 w1563 w1594 w1620 w1652 w1711 w1742 w1785 w1822 w1861 w1972 w2084 w2158 w2289 w2402 w2524 w2563 w2590 w2632 w2665 w2742 w2835]
      tunnel: [w165 _ _ _ _ _ w1014 w1062 w1167 w1213 w1288 w1357 w1432 w1515 w1563 w1594 w1620 w1652 w1711 w1742 w1785 w1822 w1861 w1972 w2084 w2158 w2289 w2402 w2524 w2563 w2590 w2632 w2665 w2742 w2835] -> w77
      tunnel: [w164 _ _ _ _ _ w1020 w1059 w1165 w1211 w1286 w1355 w1430 w1513 w1561 w1592 w1618 w1650 w1709 w1740 w1783 w1820 w1857 w1968 w2079 w2154 w2286 w2400 w2522 w2561 w2588 w2630 w2663 w2740 w2834] -> w76
      tunnel: w75 -> [w163 _ _ _ _ _ w1020 w1059 w1165 w1211 w1286 w1355 w1430 w1513 w1561 w1592 w1618 w1650 w1709 w1740 w1783 w1820 w1857 w1968 w2079 w2155 w2286 w2400 w2522 w2561 w2588 w2630 w2663 w2740 w2834]
      tunnel: w74 -> [w162 _ _ _ _ _ w1019 w1056 w1164 w1210 w1284 w1354 w1429 w1512 w1560 w1591 w1617 w1649 w1708 w1739 w1782 w1819 w1856 w1967 w2078 w2150 w2285 w2397 w2521 w2560 w2587 w2629 w2662 w2739 w2833]
      tunnel: [w161 _ _ _ _ _ w1019 w1056 w1164 w1210 w1284 w1354 w1429 w1512 w1560 w1591 w1617 w1649 w1708 w1739 w1782 w1819 w1856 w1967 w2078 w2150 w2284 w2397 w2521 w2560 w2587 w2629 w2662 w2739 w2833] -> w73
      tunnel: w72 -> [w160 _ _ _ _ _ w1018 w1055 w1163 w1209 w1283 w1353 w1428 w1511 w1559 w1590 w1616 w1648 w1707 w1738 w1781 w1818 w1855 w1966 w2077 w2149 w2280 w2399 w2520 w2559 w2586 w2628 w2661 w2738 w2832]
      tunnel: [w159 _ _ _ _ _ w1018 w1055 w1163 w1209 w1283 w1353 w1428 w1511 w1559 w1590 w1616 w1648 w1707 w1738 w1781 w1818 w1855 w1966 w2077 w2149 w2280 w2398 w2520 w2559 w2586 w2628 w2661 w2738 w2832] -> w71
      tunnel: w70 -> [w158 _ _ _ _ _ w1017 _ w1162 w1208 w1282 w1352 w1427 w1510 w1558 w1589 w1614 w1646 w1706 w1737 w1780 w1817 w1854 w1965 w2076 w2148 w2279 _ w2506 w2545 w2575 w2616 _ _ w2799]
      tunnel: [w158 _ _ _ _ _ w1017 _ w1162 w1208 w1282 w1352 w1427 w1510 w1558 w1589 w1614 w1646 w1706 w1737 w1780 w1817 w1854 w1965 w2076 w2148 w2279 _ w2506 w2545 w2575 w2616 _ _ w2799] -> w69
      tunnel: w68 -> [w157 _ _ _ _ _ _ _ _ _ _ _ _ _ _ _ _ _ _ _ _ _ _ _ _ _ _ _ _ _ _ _ _ _ _]
      tunnel: [w156 _ _ _ _ _ _ _ _ _ _ _ _ _ _ _ _ _ _ _ _ _ _ _ _ _ _ _ _ _ _ _ _ _ _] -> w66
      tunnel: w65 -> [w155 _ _ _ _ _ w1015 w1063 w1166 w1212 w1287 w1356 w1431 w1514 w1562 w1593 w1619 w1651 w1710 w1741 w1784 w1821 w1858 w1969 w2080 w2151 w2281 w2393 w2507 w2546 w2576 w2617 w2658 w2735 w2827]
      tunnel: [w154 _ _ _ _ _ w1015 w1063 w1166 w1212 w1287 w1356 w1431 w1514 w1562 w1593 w1619 w1651 w1710 w1741 w1784 w1821 w1858 w1969 w2080 w2151 w2281 w2393 w2507 w2546 w2576 w2617 w2658 w2735 w2803] -> w59
      tunnel: w64 -> [w153 _ _ _ _ _ w1016 w1060 w1161 w1207 w1285 w1351 w1426 w1509 w1557 w1588 w1615 w1647 w1705 w1736 w1779 w1816 w1853 w1964 w2075 w2147 w2278 w2392 w2505 w2544 w2574 _ w2657 w2734 w2828]
      tunnel: [w152 _ _ _ _ _ w1016 w1060 w1161 w1207 w1285 w1351 w1426 w1509 w1557 w1588 w1615 w1647 w1705 w1736 w1779 w1816 w1853 w1964 w2075 w2147 w2278 w2392 w2505 w2544 w2574 _ w2657 w2734 w2808] -> w63
      tunnel: w57 -> [w151 _ _ _ _ _ w1022 w1065 w1170 w1216 w1291 w1360 w1435 w1518 w1566 w1597 w1623 w1655 w1714 w1745 w1787 w1824 w1860 w1971 w2082 w2153 w2283 w2395 w2518 _ w2585 w2627 w2660 w2737 w2801]
      tunnel: [w150 _ _ _ _ _ w1022 w1065 w1170 w1216 w1291 w1360 w1435 w1518 w1566 w1597 w1623 w1655 w1714 w1745 w1787 w1824 w1860 w1971 w2082 w2153 w2283 w2395 w2518 "Alarm Events" w2585 w2627 w2660 w2737 w2801] -> w56
      tunnel: w55 -> [w149 _ _ _ _ _ w1023 w1064 w1169 w1215 w1290 w1359 w1434 w1517 w1565 w1596 w1622 w1654 w1713 w1744 w1786 w1823 w1859 w1970 w2081 w2152 w2282 w2394 w2517 w2543 w2573 w2615 w2659 w2736 w2800]
      tunnel: [w148 _ _ _ _ _ w1023 w1064 w1169 w1215 w1290 w1359 w1434 w1517 w1565 w1596 w1622 w1654 w1713 w1744 w1786 w1823 w1859 w1970 w2081 w2152 w2282 w2394 w2517 w2543 w2573 w2615 w2659 w2736 w2800] -> w54
      event Timeout {
        # "Reset if\ncomm error"
        # "Initialization and configuration data collection state machine."
        n18 = event-data() -> ()  [unwired: 1 in, 1 out]
        n19 = case shown="2" w192 {
          selector: w192 -> [w226 w297 w339 w379 w471 w533 w633 w727 w793 w894]
          tunnel: w174 -> [w229 w295 w319 w396 w495 w568 w608 w688 w754 w897]
          tunnel: w191 -> [w228 w294 w318 w395 w494 w566 w604 w704 w755 w896]
          tunnel: w190 -> [w213 w264 w312 w377 w446 w544 w584 w687 w756 w871]
          tunnel: [w225 w296 w338 w380 w470 w532 w632 w726 w794 w894] -> w181
          tunnel: [w224 w292 w314 w389 w444 w545 w594 w683 w786 w872] -> w180
          tunnel: [w223 w293 w316 w391 w445 w546 w595 w691 w754 w874] -> w189
          tunnel: w188 -> [w221 w273 w337 w394 w496 w570 w634 w723 w790 w895]
          tunnel: [w220 w273 w337 w394 w496 w570 w634 w723 w790 w895] -> w187
          tunnel: w186 -> [_ w272 w336 w378 w469 w569 w665 w722 w791 _]
          tunnel: [FALSE ("Data Changed") w272 w336 w378 w469 w569 w665 w722 w791 TRUE] -> w185
          tunnel: [w201 w265 w321 w370 w467 w530 w612 w724 w792 w821] -> w183
          tunnel: w184 -> [w201 _ w321 w370 w467 w530 w612 w724 w792 w821]
          tunnel: [w214 w276 w322 w364 w497 w571 w641 w716 w771 w881] -> w178
          tunnel: w177 -> [w214 w275 w322 w364 w497 w571 w641 w716 w771 w881]
          tunnel: w176 -> [w215 w266 w335 w372 w473 w550 w615 w702 w795 w893]
          tunnel: [w215 w266 w335 w373 w473 w550 w615 w702 w795 w893] -> w175
          tunnel: [w213 w264 w310 w377 w446 w544 w584 w687 w756 w869] -> w173
          tunnel: [w212 w263 w334 w363 w468 w531 w613 w728 w785 w841] -> w172
          tunnel: w171 -> [w212 w263 w334 w363 w468 w531 w613 w728 w785 w863]
          tunnel: w170 -> [w200 w262 w333 w371 w466 w529 w611 w725 w784 w868]
          tunnel: [w200 w262 w333 w374 w466 w529 w611 w725 w784 w868] -> w169
          tunnel: w168 -> [w211 w258 w324 w369 w459 w528 w610 w730 w783 w859]
          tunnel: [w211 w257 w324 w369 w465 w528 w610 w730 w783 w858] -> w167
          tunnel: w166 -> [w210 w255 w323 w368 w453 w527 w609 w729 w782 w852]
          tunnel: [w210 w254 w323 w368 w453 w524 w609 w729 w782 w851] -> w165
          tunnel: [w209 w252 w332 w367 w452 w517 w605 w721 w781 w848] -> w164
          tunnel: w163 -> [w209 w252 w332 w367 w452 w517 w602 w721 w781 w848]
          tunnel: w162 -> [w208 w251 w331 w366 w451 w516 w598 w720 w780 w823]
          tunnel: [w208 w251 w331 w366 w451 w516 w597 w720 w780 w823] -> w161
          tunnel: w160 -> [w207 w250 w330 w365 w450 w515 w591 w719 w779 w824]
          tunnel: [w207 w250 w330 w365 w450 w515 w590 w719 w779 w824] -> w159
          tunnel: w158 -> [_ _ _ _ _ _ _ _ w778 _]
          tunnel: w157 -> [w206 w249 w329 w357 w449 w514 w589 w718 w776 _]
          tunnel: [w206 w249 w329 w357 w449 w514 w589 w718 w776 TRUE] -> w156
          tunnel: w155 -> [w205 w247 w328 w356 w448 w513 w588 _ w760 w842]
          tunnel: [w205 w247 w328 w356 w448 w513 w588 w696 w760 w842] -> w154
          tunnel: w153 -> [w204 w246 w327 w355 w447 w512 w587 _ w759 w843]
          tunnel: [w204 w246 w327 w355 w447 w512 w587 w699 w759 w843] -> w152
          tunnel: w151 -> [w203 w245 w326 w354 w443 w511 w586 _ w758 w837]
          tunnel: [w203 w245 w326 w354 w443 w511 w586 w679 w758 w836] -> w150
          tunnel: [w202 w244 w325 w353 w442 w510 w585 w677 w757 w838] -> w148
          tunnel: w149 -> [w202 w244 w325 w353 w442 w510 w585 _ w757 w835]
          frame 0 {
            # "Read EE Index 3 to check if device is present"
            # "Notify the user that the VI is being initialized and disable updates to the front panel. Init Gas and EU combo boxes."
            n20 = call "Read EEPROM Index (SubVI).vi"("Address"=w213, "error in (no error)"=w228, "Index"=3, "VISA Refnum in"=w229) -> ("error out"=w227:errorcluster, "VISA Refnum out"=w223:refnum<visa-resource-name>)  [unwired: 5 in, 1 out]
            n21 = call "Init Gas Ring Items (SubVI).vi"("name or relative path"="GasTable1.txt") -> ("Array"=w197:string[])  [unwired: 9 in]
            n22 = property on="Mixture Gas 4" class="Ring (strict)"("Strings []"=w197) -> ()  [unwired: 2 in, 2 out]
            n23 = call "Init Gas Combo (SubVI).vi"("name or relative path"="GasTable.txt") -> ("Array"=w199:cluster{"String":string, "Value":string}[])  [unwired: 10 in]
            n24 = property on="Selected Gas" class="CmbBox"("Strings And Values[]"=w199) -> ()  [unwired: 2 in, 2 out]
            n25 = property on="Mixture Gas 1" class="Ring (strict)"("Strings []"=w197) -> ()  [unwired: 2 in, 2 out]
            n26 = property on="Mixture Gas 2" class="Ring (strict)"("Strings []"=w197) -> ()  [unwired: 2 in, 2 out]
            n27 = property on="Mixture Gas 3" class="Ring (strict)"("Strings []"=w197) -> ()  [unwired: 2 in, 2 out]
            n28 = property on="Mixture Gas 5" class="Ring (strict)"("Strings []"=w197) -> ()  [unwired: 2 in, 2 out]
            n29 = Unbundle(w221) -> (w219:refnum<vi>, "Panel"=w218:refnum<vi>)
            n30 = case shown="No Error" w227 {
              selector: w227 -> [w234 _]
              tunnel: [w239 errorcluster {"status"=FALSE, "code"=0, "source"=""} ("error out")] -> w224
              tunnel: [w238 w243] -> w217
              tunnel: w218 -> [w237 w243]
              tunnel: w226 -> [w233 w241]
              tunnel: [w232 w241] -> w225
              frame No Error {
                # "Only disable updates if instrument is present"
                n31 = property on="Wait Message" class="Clust (strict)"(error in=w234, "Visible"=TRUE) -> (error out=w235:errorcluster)  [unwired: 1 in, 1 out]
                n32 = Increment(x=w233) -> (x+1=w232:i32)
                n33 = property class="Pnl"(reference=w237, error in=w235, "DeferPanUpdts"=TRUE ("Defer Panel Updates")) -> (reference out=w238:refnum<vi>, error out=w239:errorcluster)
              }
              frame Error {
                # "Reset error flag."
              }
            }
            n34 = disable-structure shown="Default" {
              frame Enabled {
                # "Test Only"
                n35 = global read "Global.vi" "Gas Density"() -> (w231:dbl[])
                n36 = Array Size(array=w231) -> ()  [unwired: 1 out]
                n37 = Index Array(array=w231, index=0) -> ()  [unwired: 1 out]
              }
            }
            n38 = Bundle(cluster=w221, w219, "Panel"=w217) -> (w220:cluster{refnum<vi>, "Panel":refnum<vi>})
            n39 = call "Init Gas Density Array (SubVI).vi"("name or relative path"="GasDensity.txt") -> ()  [unwired: 10 in, 1 out]
            n40 = call "Init Pressure EU Array (SubVI).vi"("name or relative path"="Pressure Units.txt") -> ()  [unwired: 11 in]
            n41 = call "Init Mass EU Array (SubVI).vi"("name or relative path"="Mass Units.txt") -> ()  [unwired: 11 in]
          }
          frame 1 {
            # "Front Panel Initialization: Obtaining first set of instrument configuration parameters."
            n42 = Increment(x=w297) -> (x+1=w296:i32)
            n43 = call "Read Device Configuration (SubVI).vi"("error in (no error)"=w294, "Address"=w264, "VISA Refnum in"=w295) -> ("error out"=w292:errorcluster, "Device Information"=w291:T25, "VISA Refnum out"=w293:refnum<visa-resource-name>)  [unwired: 4 in, 2 out]
            n44 = Unbundle(w291) -> ("Model Number"=w284:string, "Serial Number"=w283:string, "Gas Name"=w282:string, "FS Range"=w281:string, "Mass Flow EU"=w256:string, "Volumetric Flow EU"=w259:string, "Modbus"=w280:string, "Totalizer#1 Mode"=w271:string, "Totalizer#2 Mode"=w279:string, "Analog Output"=w278:string, "Pressure EU"=w270:string, "Temperature EU"=w269:string, "Device Function"=w286:string)
            n45 = Decimal String To Number(string=w286) -> (number=w287:i32)  [unwired: 2 in, 1 out]
            n46 = Equal?(x=w287, y=0) -> (x = y?=w274:bool)
            n47 = call <vilib>:"Trim Whitespace.vi"("string"=w256) -> ("trimmed string"=w261:string)  [unwired: 1 in]
            n48 = call <vilib>:"Trim Whitespace.vi"("string"=w259) -> ("trimmed string"=w260:string)  [unwired: 1 in]
            n49 = property on="Mass Flow Units" class="CmbBox"("Value"=w261) -> ()  [unwired: 2 in, 2 out]
            n50 = property on="Vol. Flow Units" class="CmbBox"("Value"=w260) -> ()  [unwired: 2 in, 2 out]
            n51 = Select(t="Meter", s=w274, f="Controller") -> (s? t:f=w285:string)
            n52 = Bundle(cluster=w275, "Device Function"=w285, "Model Number"=w284, "Serial Number"=w283, "Selected Gas"=w282, "Full Scale Range"=w281, "Mass EU"=w256, "Volum. EU"=w259, "T1"=w271, "T2"=w279, "A Output"=w278, "A Input"="0", "Modbus"=w280) -> (w276:T14)
            "Device Information" <- w276
            n53 = call "Convert Mass Flow EU to Totalizer EU (SubVI).vi"("Mass Flow EU"=w256) -> ("Totalizer EU"=w253:string)  [unwired: 10 in]
            n54 = Not(x=w274) -> (.not. x?=w265:bool)
            n55 = property on="Pressure Units" class="CmbBox"("Value"=w270) -> ()  [unwired: 2 in, 2 out]
            n56 = property on="Temperature Units" class="CmbBox"("Value"=w269) -> ()  [unwired: 2 in, 2 out]
            n57 = property on="Total1 Vol Units" class="Str"("Value"=w253) -> ()  [unwired: 2 in, 2 out]
            n58 = property on="Total2 Vol Units" class="Str"("Value"=w253) -> ()  [unwired: 2 in, 2 out]
            n59 = Bundle By Name(cluster=w258, "Total EU 1"=w253, "Total EU 2"=w253) -> (w257:T20)
            n60 = Unbundle(w266) -> ("Enabled"=w268:T26, "Disabled and Grayed Out"=w267:T26)
            n61 = property on="Total EU 1" class="Str"("Value"=w253) -> ()  [unwired: 2 in, 2 out]
            n62 = Select(t=w268, s=w265, f=w267) -> (s? t:f=w248:T26)
            n63 = property on="Chart: Set Point" class="Bool (strict)"("DisabledEnum"=w248) -> ()  [unwired: 2 in, 2 out]
            n64 = case shown="True" w265 {
              frame False {
                n65 = property on="Set Point" class="Str"("Value"="") -> (error out=w301:errorcluster)  [unwired: 2 in, 1 out]
                n66 = property on="A Input" class="Str"(error in=w301, "Value"="N/A") -> (error out=w299:errorcluster)  [unwired: 1 in, 1 out]
                n67 = property on="Chart: Set Point" class="Bool (strict)"(error in=w299, "Value"=FALSE) -> ()  [unwired: 1 in, 2 out]
              }
              frame True {
                n68 = property on="Chart: Set Point" class="Bool (strict)"("Value"=TRUE) -> ()  [unwired: 2 in, 2 out]
              }
            }
            n69 = property on="Set Point Options" class="Clust (strict)"("DisabledEnum"=w248) -> ()  [unwired: 2 in, 2 out]
            n70 = property on="Total EU 2" class="Str"("Value"=w253) -> ()  [unwired: 2 in, 2 out]
            n71 = Bundle By Name(cluster=w255, "Total EU 1"=w253, "Total EU 2"=w253) -> (w254:T19)
            n72 = property on="Total EU 1" class="Str"("Value"=w253) -> ()  [unwired: 2 in, 2 out]
            n73 = property on="Analog Input" class="CmbBox"("DisabledEnum"=w248) -> ()  [unwired: 2 in, 2 out]
            n74 = property on="Pulse Unit" class="Str"("Value"=w253) -> ()  [unwired: 2 in, 2 out]
            n75 = property on="Total EU 2" class="Str"("Value"=w253) -> ()  [unwired: 2 in, 2 out]
          }
          frame 2 {
            w320 = ""
            # "Gas Mixture Initialization: Obtaining Gas Mixture parameters and updating Gas Select Combo Box."
            n76 = Increment(x=w339) -> (x+1=w338:i32)
            n77 = call "Process Compose Mixture Command (SubVI).vi"("Argument#4"=w320, "Argument#2"=w320, "Argument#1"=w320, "Address"=w312, "error in (no error)"=w318, "Argument#3"=w320, "VISA Refnum in"=w319) -> ("error out"=w313:errorcluster, "CM Output String"=w317:string, "VISA Refnum out"=w315:refnum<visa-resource-name>)  [unwired: 2 in]
            n78 = Decimal String To Number(string=w317) -> (number=w308:i32)  [unwired: 2 in, 1 out]
            n79 = To Unsigned Word Integer(number=w308) -> (unsigned 16bit integer=w309:u16)
            "Total GM:" <- w309
            n80 = Add(x=w308, y=200) -> (x+y=w304:i32)
            n81 = global write "Global.vi" "GM Number"(w308) -> ()
            n82 = Less Or Equal?(x=w304, y=219) -> (x <= y?=w305:bool)
            n83 = case shown="True" w305 {
              tunnel: w304 -> [_ w341]
              frame False {
                n84 = property on="Mix. #" class="DigNum (strict)"("Value"=219) -> ()  [unwired: 2 in, 2 out]
              }
              frame True {
                n85 = property on="Mix. #" class="DigNum (strict)"("Value"=w341) -> ()  [unwired: 2 in, 2 out]
              }
            }
            n86 = Greater Than 0?(x=w309) -> (x > 0?=w311:bool)
            n87 = case shown="True" w311 {
              tunnel: [w343 w352] -> w316
              tunnel: w315 -> [w343 w351]
              tunnel: [w342 w350] -> w314
              tunnel: w313 -> [w342 w349]
              tunnel: w312 -> [w344 w348]
              tunnel: [w344 w348] -> w310
              tunnel: w309 -> [_ w347]
              frame False {
              }
              frame True {
                n88 = property on="Selected Gas" class="CmbBox"() -> ("Strings And Values[]"=w346:T27)  [unwired: 2 in, 2 out]
                n89 = call "Update Gas Combo with GM (SubVI).vi"("VISA Refnum in"=w351, "Array In"=w346, "Number of Mixtures"=w347, "error in (no error)"=w349, "Address String"=w348) -> ("VISA Refnum out"=w352:refnum<visa-resource-name>, "Array Out"=w345:cluster{"String":string, "Value":string}[], "error out"=w350:errorcluster)  [unwired: 3 in]
                n90 = property on="Selected Gas" class="CmbBox"("Strings And Values[]"=w345) -> ()  [unwired: 2 in, 2 out]
              }
            }
          }
          frame 3 {
            # "Get Controller related parameters if instrument is \"Controller\""
            n91 = Increment(x=w379) -> (x+1=w380:i32)
            n92 = call "Get Controller SP Parameters (SubVI).vi"("error in (no error)"=w395, "Controller?"=w370, "Address"=w377, "VISA Refnum in"=w396) -> ("error out"=w390:errorcluster, "SP and Valve Parameters"=w393:T28, "VISA Refnum out"=w392:refnum<visa-resource-name>)  [unwired: 5 in]
            n93 = Unbundle By Name(w364) -> ("Selected Gas"=w381:string)
            n94 = property on="Mass Flow Units" class="CmbBox"() -> ("Value"=w361:string)  [unwired: 2 in, 2 out]
            n95 = case shown="True" w370 {
              tunnel: w393 -> [_ w425]
              tunnel: w370 -> [_ w422]
              tunnel: [w397 w403] -> w374
              tunnel: w372 -> [w398 w404]
              tunnel: [w398 w404] -> w373
              tunnel: w371 -> [w397 _]
              frame False {
              }
              frame True {
                (unwired) 1
                n96 = Unbundle(w425) -> ("Setpoint Source Out"=w406:string, "Valve Mode Out"=w400:string, w402:dbl)
                n97 = String Subset(string=w400, offset (0)=0) -> (substring=w399:string)  [unwired: 1 in]
                n98 = String Subset(string=w406, offset (0)=0, length (rest)=1) -> (substring=w410:string)
                n99 = Equal?(x=w410, y="P") -> (x = y?=w417:bool)
                n100 = property on="Valve Mode" class="CmbBox"("Value"=w399) -> ()  [unwired: 2 in, 2 out]
                n101 = Equal?(x=w410, y="A") -> (x = y?=w416:bool)
                n102 = String Subset(string=w406, offset (0)=0, length (rest)=1) -> (substring=w405:string)
                n103 = Or(x=w416, y=w417) -> (x .or. y?=w415:bool)
                n104 = Not(x=w415) -> (.not. x?=w409:bool)
                n105 = Unbundle(w404) -> ("Enabled"=w424:T26, "Disabled and Grayed Out"=w423:T26)
                n106 = Unbundle(w404) -> ("Enabled"=w413:T26, "Disabled and Grayed Out"=w414:T26)
                n107 = Select(t=w424, s=w422, f=w423) -> (s? t:f=w421:T26)
                n108 = To Double Precision Float(number=w402) -> (double precision float=w403:dbl)
                n109 = property on="Setpoint Source" class="CmbBox"("Value"=w405) -> ()  [unwired: 2 in, 2 out]
                n110 = Select(t=w413, s=w409, f=w414) -> (s? t:f=w412:T26)
                n111 = property on="Valve Mode" class="CmbBox"("DisabledEnum"=w421) -> ()  [unwired: 2 in, 2 out]
                n112 = property on="Setpoint Value" class="DigNum (strict)"("DisabledEnum"=w412) -> ()  [unwired: 2 in, 2 out]
                n113 = property on="Setpoint Value" class="DigNum (strict)"("Value"=w403) -> ()  [unwired: 2 in, 2 out]
              }
            }
            n114 = Unbundle By Name(w364) -> ("Full Scale Range"=w362:string)
            n115 = Search/Split String(string=w381, search string/char (-)=",") -> (substring before match=w360:string)  [unwired: 1 in, 2 out]
            n116 = call "Get Max Limit and Precision (SubVI).vi"("Gas Index"=w360, "Full Scale SLPM"=w362, "EU Name"=w361) -> ("SP Max Limit"=w359:dbl, "Mass EU Precision"=w358:u32)  [unwired: 5 in, 1 out]
            n117 = property on="Selected Gas" class="CmbBox"("Value"=w360) -> ()  [unwired: 2 in, 2 out]
            n118 = property on="Setpoint Value" class="DigNum (strict)"("Precision"=w358) -> ()  [unwired: 2 in, 2 out]
            n119 = Unbundle By Name(w364) -> ("Mass EU"=w375:string)
            n120 = property on="Setpoint Value" class="DigNum (strict)"("Maximum"=w359) -> ()  [unwired: 2 in, 2 out]
            n121 = Unbundle By Name(w364) -> ("A Output"=w384:string)
            n122 = call <vilib>:"Trim Whitespace.vi"("string"=w375) -> ("trimmed string"=w376:string)  [unwired: 1 in]
            n123 = property on="Mass Flow EU 2" class="Str"("Value"=w376) -> ()  [unwired: 2 in, 2 out]
            n124 = case shown="True" w370 {
              tunnel: w392 -> [w434 w441]
              tunnel: [w434 w440] -> w391
              tunnel: w390 -> [w433 w439]
              tunnel: [w433 w438] -> w389
              tunnel: w377 -> [_ w436]
              tunnel: ["0" w435] -> w388
              frame False {
              }
              frame True {
                n125 = call "Process Analog Input Command (SubVI).vi"("Analog Inp Mode In"="", "Address"=w436, "error in (no error)"=w439, "VISA Refnum in"=w441) -> ("error out"=w438:errorcluster, "Analog Inp Mode Out"=w435:string, "VISA Refnum out"=w440:refnum<visa-resource-name>)  [unwired: 5 in]
              }
            }
            n126 = case shown="\"0-5Vdc\", Default" w384 {
              tunnel: ["0" "1" "2"] -> w383
              frame "0-5Vdc", Default {
              }
              frame "0-10Vdc" {
              }
              frame "4-20mA" {
              }
            }
            n127 = case shown="\"0\", Default" w388 {
              tunnel: ["0-5Vdc" "0-10Vdc" "4-20mA"] -> w386
              frame "0", Default {
              }
              frame "1" {
              }
              frame "2" {
              }
            }
            n128 = property on="Analog Output" class="CmbBox"("Value"=w383) -> ()  [unwired: 2 in, 2 out]
            n129 = property on="Analog Input" class="CmbBox"("Value"=w388) -> ()  [unwired: 2 in, 2 out]
            n130 = Select(t=w386, s=w370, f="N/A") -> (s? t:f=w387:string)
            n131 = property on="A Input" class="Str"("Value"=w387) -> ()  [unwired: 2 in, 2 out]
          }
          frame 4 {
            # "Read SSR and Totalizer#1 Configuration Parameters"
            n132 = Increment(x=w471) -> (x+1=w470:i32)
            n133 = call "Process Relay Command (SubVI).vi"("Relay Mode In"="S", "Address"=w446, "error in (no error)"=w494, "VISA Refnum in"=w495) -> ("error out"=w490:errorcluster, "Relay Mode Out"=w492:string, "VISA Refnum out"=w491:refnum<visa-resource-name>)  [unwired: 5 in]
            n134 = Unbundle(w473) -> ("Enabled"=w475:T26, "Disabled and Grayed Out"=w474:T26)
            n135 = property on="SS Relay Assignment" class="CmbBox"("Value"=w492) -> ()  [unwired: 2 in, 2 out]
            n136 = Select(t=w475, s=w467, f=w474) -> (s? t:f=w472:T26)
            n137 = call "Read Totalizer Configuration (SubVI).vi"("Totalizer Number"="1", "Address"=w446, "error in (no error)"=w490, "VISA Refnum in"=w491) -> ("error out"=w487:errorcluster, "Tot. Status"=w486:T29, "VISA Refnum out"=w488:refnum<visa-resource-name>)  [unwired: 4 in, 1 out]
            n138 = Unbundle(w486) -> ("Tot. Mode"=w485:string, "Start @ Flow"=w483:string, "Limit Volume"=w482:string, "Power Up Delay"=w481:string, "Auto Reset Mode"=w479:string, "Auto Reset Delay"=w478:string)
            n139 = case shown="True" w467 {
              tunnel: w488 -> [w500 w509]
              tunnel: w487 -> [w499 w508]
              tunnel: [w500 w507] -> w445
              tunnel: [w499 w506] -> w444
              tunnel: w446 -> [w501 w502]
              tunnel: ["0" w503] -> w476
              tunnel: [w501 w502] -> _
              frame False {
              }
              frame True {
                n140 = call "Totalizer Valve Action Command (SubVI).vi"("Valve Action In"="", "Totalizer Number"="1", "Address"=w502, "error in (no error)"=w508, "VISA Refnum in"=w509) -> ("error out"=w506:errorcluster, "Valve Action Out"=w503:string, "VISA Refnum out"=w507:refnum<visa-resource-name>)  [unwired: 4 in]
              }
            }
            n141 = Equal?(x=w485, y="E") -> (x = y?=w464:bool)
            n142 = Fract/Exp String To Number(string=w483) -> (number=w463:dbl)  [unwired: 3 in, 1 out]
            n143 = To Double Precision Float(number=w463) -> (double precision float=w462:dbl)
            n144 = property on="Enabled" class="Bool (strict)"("Value"=w464) -> ()  [unwired: 2 in, 2 out]
            n145 = property on="Start @ Flow" class="DigNum (strict)"("Value"=w462) -> ()  [unwired: 2 in, 2 out]
            n146 = Fract/Exp String To Number(string=w482) -> (number=w461:dbl)  [unwired: 3 in, 1 out]
            n147 = Equal?(x=w476, y="V") -> (x = y?=w457:bool)
            n148 = Bundle By Name(cluster=w459, "Close Valve When Limit Volume is Reached"=w457) -> (w458:T20)
            n149 = To Double Precision Float(number=w461) -> (double precision float=w460:dbl)
            n150 = property on="Close Valve When Action Volume is Reached" class="Bool (strict)"("Value"=w457, "DisabledEnum"=w472) -> ()  [unwired: 2 in, 2 out]
            n151 = Decimal String To Number(string=w481) -> (number=w454:i32)  [unwired: 2 in, 1 out]
            n152 = property on="Action Volume" class="DigNum (strict)"("Value"=w460) -> ()  [unwired: 2 in, 2 out]
            n153 = property on="Power Up Delay [seconds]" class="DigNum (strict)"("Value"=w454) -> ()  [unwired: 2 in, 2 out]
            n154 = Equal?(x=w479, y="1") -> (x = y?=w455:bool)
            n155 = property on="Enable Auto Reset/Reload" class="Bool (strict)"("Value"=w455) -> ()  [unwired: 2 in, 2 out]
            n156 = Decimal String To Number(string=w478) -> (number=w456:i32)  [unwired: 2 in, 1 out]
            n157 = Bundle By Name(cluster=w458, "Enabled"=w464, "Start @ Flow"=w462, "Limit Volume"=w460, "Auto Reset Delay [seconds]"=w456, "Power Up Delay [seconds]"=w454, "Enable Auto Reset/Reload"=w455) -> (w465:T20)
            n158 = property on="Auto Reset Delay [seconds]" class="DigNum (strict)"("Value"=w456) -> ()  [unwired: 2 in, 2 out]
          }
          frame 5 {
            # "Read Totalizer#2 and Pulse Output Configuration Parameters"
            n159 = Increment(x=w533) -> (x+1=w532:i32)
            n160 = call "Read Totalizer Configuration (SubVI).vi"("Totalizer Number"="2", "Address"=w544, "error in (no error)"=w566, "VISA Refnum in"=w568) -> ("error out"=w565:errorcluster, "Tot. Status"=w555:T29, "VISA Refnum out"=w567:refnum<visa-resource-name>)  [unwired: 4 in, 1 out]
            n161 = Unbundle(w555) -> ("Tot. Mode"=w563:string, "Start @ Flow"=w561:string, "Limit Volume"=w560:string, "Power Up Delay"=w559:string, "Auto Reset Mode"=w557:string, "Auto Reset Delay"=w556:string)
            n162 = Unbundle(w550) -> ("Enabled"=w554:T26, "Disabled and Grayed Out"=w553:T26)
            n163 = Select(t=w554, s=w530, f=w553) -> (s? t:f=w549:T26)
            n164 = Equal?(x=w563, y="E") -> (x = y?=w523:bool)
            n165 = Fract/Exp String To Number(string=w561) -> (number=w522:dbl)  [unwired: 3 in, 1 out]
            n166 = case shown="True" w530 {
              tunnel: w567 -> [w574 w581]
              tunnel: w565 -> [w573 w580]
              tunnel: ["0" w579] -> w551
              tunnel: [w574 w578] -> w548
              tunnel: [w573 w577] -> w547
              tunnel: w544 -> [w575 w576]
              tunnel: [w575 w576] -> _
              frame False {
              }
              frame True {
                n167 = call "Totalizer Valve Action Command (SubVI).vi"("Valve Action In"="", "Totalizer Number"="2", "Address"=w576, "error in (no error)"=w580, "VISA Refnum in"=w581) -> ("error out"=w577:errorcluster, "Valve Action Out"=w579:string, "VISA Refnum out"=w578:refnum<visa-resource-name>)  [unwired: 4 in]
              }
            }
            n168 = property on="Enabled" class="Bool (strict)"("Value"=w523) -> ()  [unwired: 2 in, 2 out]
            n169 = property on="Start @ Flow" class="DigNum (strict)"("Value"=w522) -> ()  [unwired: 2 in, 2 out]
            n170 = Fract/Exp String To Number(string=w560) -> (number=w521:dbl)  [unwired: 3 in, 1 out]
            n171 = call "Read Pulse Output Configuration (SubVI).vi"("Prefix"=w544, "error in (no error)"=w547, "VISA Refnum in"=w548) -> ("error out"=w545:errorcluster, "Pulse Output Configuration"=w543:T30, "VISA Refnum out"=w546:refnum<visa-resource-name>)  [unwired: 5 in, 1 out]
            n172 = property on="Action Volume" class="DigNum (strict)"("Value"=w521) -> ()  [unwired: 2 in, 2 out]
            n173 = Decimal String To Number(string=w559) -> (number=w519:i32)  [unwired: 2 in, 1 out]
            n174 = Equal?(x=w551, y="V") -> (x = y?=w526:bool)
            n175 = Bundle By Name(cluster=w527, "Close Valve When Limit Volume is Reached"=w526) -> (w525:T19)
            n176 = Unbundle(w543) -> ("Enabled"=w541:string, "Start @ Flow"=w539:string, "Unit Per Pulse"=w537:string, "Pulse Active Time"=w535:string)
            n177 = property on="Close Valve When Action Volume is Reached" class="Bool (strict)"("Value"=w526, "DisabledEnum"=w549) -> ()  [unwired: 2 in, 2 out]
            n178 = property on="Power Up Delay [Seconds]" class="DigNum (strict)"("Value"=w519) -> ()  [unwired: 2 in, 2 out]
            n179 = Equal?(x=w557, y="1") -> (x = y?=w518:bool)
            n180 = Decimal String To Number(string=w556) -> (number=w520:i32)  [unwired: 2 in, 1 out]
            n181 = Equal?(x=w541, y="E") -> (x = y?=w540:bool)
            n182 = property on="Enable Auto Reset/Reload" class="Bool (strict)"("Value"=w518) -> ()  [unwired: 2 in, 2 out]
            n183 = property on="Enabled" class="Bool (strict)"("Value"=w540) -> ()  [unwired: 2 in, 2 out]
            n184 = property on="Auto Reset Delay [Seconds]" class="DigNum (strict)"("Value"=w520) -> ()  [unwired: 2 in, 2 out]
            n185 = Fract/Exp String To Number(string=w539) -> (number=w538:dbl)  [unwired: 3 in, 1 out]
            n186 = Bundle By Name(cluster=w525, "Enabled"=w523, "Start @ Flow"=w522, "Limit Volume"=w521, "Auto Reset Delay [Seconds]"=w520, "Power Up Delay [Seconds]"=w519, "Enable Auto Reset/Reload"=w518) -> (w524:T19)
            n187 = property on="Start @ Flow Rate" class="DigNum (strict)"("Value"=w538) -> ()  [unwired: 2 in, 2 out]
            n188 = Decimal String To Number(string=w535) -> (number=w534:i32)  [unwired: 2 in, 1 out]
            n189 = property on="Pulse Active Time [ms]" class="DigNum (strict)"("Value"=w534) -> ()  [unwired: 2 in, 2 out]
            n190 = Fract/Exp String To Number(string=w537) -> (number=w536:dbl)  [unwired: 3 in, 1 out]
            n191 = property on="Unit Per Pulse" class="DigNum (strict)"("Value"=w536) -> ()  [unwired: 2 in, 2 out]
          }
          frame 6 {
            # "Read Flow ,Temperature, and Pressure Alarm Configuration"
            n192 = Increment(x=w633) -> (x+1=w632:i32)
            n193 = call "Process Flow Alarm Command (SubVI).vi"("Argument#1"="S", "Address"=w584, "error in (no error)"=w604, "Alarm Configuration In"=w602, "VISA Refnum in"=w608) -> ("error out"=w606:errorcluster, "Alarm Configuration Out"=w605:T18, "VISA Refnum out"=w607:refnum<visa-resource-name>)  [unwired: 3 in, 1 out]
            n194 = Unbundle(w605) -> ("Enabled"=w664:string, "High Alarm Limit"=w661:string, "Low Alarm Limit"=w659:string, "Action Delay"=w657:string, "Latch Mode"=w654:string, "Power Up Delay"=w652:string)
            n195 = case shown="True" w612 {
              tunnel: w607 -> [w669 w676]
              tunnel: w606 -> [w667 w675]
              tunnel: [w669 w674] -> w601
              tunnel: [w667 w673] -> w600
              tunnel: w584 -> [w668 w670]
              tunnel: ["0" w671] -> w650
              tunnel: [w668 w670] -> _
              frame False {
              }
              frame True {
                n196 = call "Read Alarm Valve Action (SubVI).vi"("Valve Action In"="", "Address"=w670, "error in (no error)"=w675, "VISA Refnum in"=w676) -> ("error out"=w673:errorcluster, "Valve Action Out"=w671:string, "VISA Refnum out"=w674:refnum<visa-resource-name>)  [unwired: 5 in]
              }
            }
            n197 = property on="Flow Alarm Valve Action:" class="CmbBox"("Value"=w650) -> ()  [unwired: 2 in, 2 out]
            n198 = Equal?(x=w664, y="E") -> (x = y?=w662:bool)
            n199 = Fract/Exp String To Number(string=w661) -> (number=w660:dbl)  [unwired: 3 in, 1 out]
            n200 = property on="Enabled" class="Bool (strict)"("Value"=w662) -> ()  [unwired: 2 in, 2 out]
            n201 = call "Process Temp Alarm Command (SubVI).vi"("Argument#1"="S", "Address"=w584, "error in (no error)"=w600, "Alarm Configuration In"=w598, "VISA Refnum in"=w601) -> ("error out"=w593:errorcluster, "Alarm Configuration Out"=w597:T18, "VISA Refnum out"=w596:refnum<visa-resource-name>)  [unwired: 3 in, 1 out]
            n202 = Unbundle(w597) -> ("Enabled"=w640:string, "High Alarm Limit"=w639:string, "Low Alarm Limit"=w638:string, "Action Delay"=w637:string, "Latch Mode"=w636:string, "Power Up Delay"=w635:string)
            n203 = property on="High Alarm Limit" class="DigNum (strict)"("Value"=w660) -> ()  [unwired: 2 in, 2 out]
            n204 = Fract/Exp String To Number(string=w659) -> (number=w658:dbl)  [unwired: 3 in, 1 out]
            n205 = call "Process Pressure Alarm Command (SubVI).vi"("Argument#1"="S", "Address"=w584, "error in (no error)"=w593, "Alarm Configuration In"=w591, "VISA Refnum in"=w596) -> ("error out"=w594:errorcluster, "Alarm Configuration Out"=w590:T18, "VISA Refnum out"=w595:refnum<visa-resource-name>)  [unwired: 3 in, 1 out]
            n206 = Equal?(x=w640, y="E") -> (x = y?=w648:bool)
            n207 = Fract/Exp String To Number(string=w639) -> (number=w647:dbl)  [unwired: 3 in, 1 out]
            n208 = Decimal String To Number(string=w657) -> (number=w656:i32)  [unwired: 2 in, 1 out]
            n209 = Unbundle(w590) -> ("Enabled"=w630:string, "High Alarm Limit"=w628:string, "Low Alarm Limit"=w626:string, "Action Delay"=w624:string, "Latch Mode"=w620:string, "Power Up Delay"=w618:string)
            n210 = Decimal String To Number(string=w618) -> (number=w619:i32)  [unwired: 2 in, 1 out]
            n211 = property on="Low Alarm Limit" class="DigNum (strict)"("Value"=w658) -> ()  [unwired: 2 in, 2 out]
            n212 = property on="Power Up Delay [s]" class="DigNum (strict)"("Value"=w619) -> ()  [unwired: 2 in, 2 out]
            n213 = property on="Enabled" class="Bool (strict)"("Value"=w648) -> ()  [unwired: 2 in, 2 out]
            n214 = property on="High Temp. Alarm Limit" class="DigNum (strict)"("Value"=w647) -> ()  [unwired: 2 in, 2 out]
            n215 = Fract/Exp String To Number(string=w638) -> (number=w646:dbl)  [unwired: 3 in, 1 out]
            n216 = Decimal String To Number(string=w652) -> (number=w651:i32)  [unwired: 2 in, 1 out]
            n217 = property on="Action Delay [s]" class="DigNum (strict)"("Value"=w656) -> ()  [unwired: 2 in, 2 out]
            n218 = Equal?(x=w654, y="1") -> (x = y?=w653:bool)
            n219 = Equal?(x=w620, y="1") -> (x = y?=w622:bool)
            n220 = Equal?(x=w630, y="E") -> (x = y?=w631:bool)
            n221 = Decimal String To Number(string=w637) -> (number=w645:i32)  [unwired: 2 in, 1 out]
            n222 = property on="Flow Alarm Latch" class="Bool (strict)"("Value"=w653) -> ()  [unwired: 2 in, 2 out]
            n223 = property on="Power Up Delay [s]" class="DigNum (strict)"("Value"=w651) -> ()  [unwired: 2 in, 2 out]
            n224 = property on="Pressure Alarm Latch" class="Bool (strict)"("Value"=w622) -> ()  [unwired: 2 in, 2 out]
            n225 = property on="Enabled" class="Bool (strict)"("Value"=w631) -> ()  [unwired: 2 in, 2 out]
            n226 = property on="Low Temp. Alarm Limit" class="DigNum (strict)"("Value"=w646) -> ()  [unwired: 2 in, 2 out]
            n227 = Unbundle(w615) -> ("Enabled"=w617:T26, "Disabled and Grayed Out"=w616:T26)
            n228 = Fract/Exp String To Number(string=w626) -> (number=w625:dbl)  [unwired: 3 in, 1 out]
            n229 = Fract/Exp String To Number(string=w628) -> (number=w627:dbl)  [unwired: 3 in, 1 out]
            n230 = Decimal String To Number(string=w624) -> (number=w623:i32)  [unwired: 2 in, 1 out]
            n231 = Select(t=w617, s=w612, f=w616) -> (s? t:f=w614:T26)
            n232 = property on="Low Pressure Alarm Limit" class="DigNum (strict)"("Value"=w625) -> ()  [unwired: 2 in, 2 out]
            n233 = property on="Action Delay [s]" class="DigNum (strict)"("Value"=w645) -> ()  [unwired: 2 in, 2 out]
            n234 = property on="High Pressure Alarm Limit" class="DigNum (strict)"("Value"=w627) -> ()  [unwired: 2 in, 2 out]
            n235 = property on="Action Delay [s]" class="DigNum (strict)"("Value"=w623) -> ()  [unwired: 2 in, 2 out]
            n236 = Equal?(x=w636, y="1") -> (x = y?=w643:bool)
            n237 = Decimal String To Number(string=w635) -> (number=w642:i32)  [unwired: 2 in, 1 out]
            n238 = property on="Flow Alarm Valve Action:" class="CmbBox"("DisabledEnum"=w614) -> ()  [unwired: 2 in, 2 out]
            n239 = property on="Temp. Alarm Latch" class="Bool (strict)"("Value"=w643) -> ()  [unwired: 2 in, 2 out]
            n240 = property on="Power Up Delay [s]" class="DigNum (strict)"("Value"=w642) -> ()  [unwired: 2 in, 2 out]
          }
          frame 7 {
            # "Generate PI Data Logging info"
            n241 = Increment(x=w727) -> (x+1=w726:i32)
            n242 = property on="Mass Flow Units" class="CmbBox"() -> ("Value"=w711:string)  [unwired: 2 in, 2 out]
            n243 = property on="Vol. Flow Units" class="CmbBox"() -> ("Value"=w710:string)  [unwired: 2 in, 2 out]
            n244 = property on="Temperature Units" class="CmbBox"() -> ("Value"=w707:string)  [unwired: 2 in, 2 out]
            n245 = Unbundle By Name(w716) -> ("Serial Number"=w715:string)
            n246 = property on="Pressure Units" class="CmbBox"() -> ("Value"=w706:string)  [unwired: 2 in, 2 out]
            n247 = call "Convert Mass Flow EU to Totalizer EU (SubVI).vi"("Mass Flow EU"=w711) -> ("Totalizer EU"=w708:string)  [unwired: 10 in]
            n248 = Concatenate Strings(w715, "_" ("string")) -> (w713:string)
            n249 = Bundle(cluster=T23 {"Mass Flow"="", "Valve Counts"="", "Volumetric Flow"="", "Totalizer"="", "Temperature"="", "Pressure"=""} ("Units of Measure Input"), "Mass Flow"=w711, "Valve Counts"="%FS, Counts", "Volumetric Flow"=w710, "Totalizer"=w708, "Temperature"=w707, "Pressure"=w706) -> (w697:T23)
            n250 = property on="PI Logging Options" class="Clust (strict)"() -> ("Value"=w700:T3)  [unwired: 2 in, 2 out]
            n251 = Unbundle By Name(w700) -> ("Log Data"=w699:bool)
            n252 = case shown="True" w699 {
              tunnel: ["" w745] -> w717
              tunnel: w713 -> [_ w742]
              frame False {
              }
              frame True {
                n253 = Get Date/Time In Seconds() -> (seconds since 1Jan1904=w751:timestamp)
                n254 = Format Date/Time String(time format string (%c)="%m-%d-%Y_%H-%M-%S", seconds (now)=w751) -> (date/time string=w750:string)  [unwired: 1 in]
                n255 = call <vilib>:"Application Directory.vi"() -> ("Application Directory"=w747:path)
                n256 = Format Date/Time String(time format string (%c)="%p", seconds (now)=w751) -> (date/time string=w749:string)  [unwired: 1 in]
                n257 = Path To String(path=w747) -> (string=w744:string)
                n258 = Concatenate Strings(w744, "\\PI Data Log_" ("string"), w742, w750, "_" ("string"), w749, ".txt" ("string")) -> (w745:string)
              }
            }
            n259 = call "Data Log Make Header.vi"("PI Logging Options"=w700, "error in"=w704, "Units of Measure Input"=w697) -> ("error out"=w703:errorcluster, "Data Log Header"=w698:string)  [unwired: 7 in]
            n260 = String To Path(string=w717) -> (path=w701:path)
            n261 = case shown="True" w699 {
              tunnel: w701 -> [_ w739]
              tunnel: w703 -> [w732 w738]
              tunnel: [w732 w736] -> w686
              tunnel: w698 -> [_ w735]
              tunnel: [refnum<file> refnum ("refnum out") w734] -> w696
              tunnel: T22."replace or create" ("operation (0:open)") -> [_ w733]
              frame False {
              }
              frame True {
                n262 = Open/Create/Replace File(file path (use dialog)=w739, error in=w738, operation (0:open)=w733) -> (refnum out=w740:refnum<file>, error out=w737:errorcluster)  [unwired: 3 in, 1 out]
                n263 = Write to Text File(file (use dialog)=w740, text=w735, error in=w737) -> (refnum out=w734:refnum<file>, error out=w736:errorcluster)  [unwired: 1 in, 1 out]
              }
            }
            n264 = call "Process Alarm Events Command (SubVI).vi"("Argument#2"="", "Argument#1"="", "Address"=w687, "error in (no error)"=w686, "VISA Refnum in"=w688) -> ("error out"=w685:errorcluster, "AE Output String"=w677:string, "VISA Refnum out"=w689:refnum<visa-resource-name>)  [unwired: 4 in]
            n265 = property on="Alarm Events" class="Str"("Value"=w677) -> ()  [unwired: 2 in, 2 out]
            n266 = call "Process Alarm Events Command (SubVI).vi"("Argument#2"="", "Argument#1"="M", "Address"=w687, "error in (no error)"=w685, "VISA Refnum in"=w689) -> ("error out"=w684:errorcluster, "AE Output String"=w678:string, "VISA Refnum out"=w690:refnum<visa-resource-name>)  [unwired: 4 in]
            n267 = call "Process Alarm Events Command (SubVI).vi"("Argument#2"="", "Argument#1"="L", "Address"=w687, "error in (no error)"=w684, "VISA Refnum in"=w690) -> ("error out"=w683:errorcluster, "AE Output String"=w682:string, "VISA Refnum out"=w691:refnum<visa-resource-name>)  [unwired: 4 in]
            n268 = call "Populate Alarm Events Data (SubVI).vi"("AE Latch String In"=w682, "AE Mask String In"=w678, "AE Status String In"=w677) -> ("Alarm Events"=w679:T2)  [unwired: 8 in]
            n269 = local write "Alarm Events"(w679) -> ()
          }
          frame 8 {
            w788 = FALSE
            # "Update Chart Scale and hide initialization message, and re-enable updates to the front panel"
            n270 = Increment(x=w793) -> (x+1=w794:i32)
            n271 = property on="Pressure Units" class="CmbBox"() -> ("Value"=w764:string)  [unwired: 2 in, 2 out]
            n272 = Unbundle By Name(w778) -> ("AutoScale Chart"=w777:bool)
            n273 = Unbundle By Name(w771) -> ("Full Scale Range"=w772:string)
            n274 = Unbundle By Name(w771) -> ("Selected Gas"=w773:string)
            n275 = call "Convert PSIA to Active Pressure EU (SubVI).vi"("PSIA Value In"=100.0 ("Y Scale.Range:Minimum"), "EU Name"=w764) -> ("Pressure Value Out"=w765:dbl)  [unwired: 9 in]
            n276 = Search/Split String(string=w773, search string/char (-)=",") -> (substring before match=w769:string)  [unwired: 1 in, 2 out]
            n277 = property on="Mass Flow Units" class="CmbBox"() -> ("Value"=w770:string)  [unwired: 2 in, 2 out]
            n278 = call "Convert PFS to Mass Flow EU (SubVI).vi"("PFS Value In"=125.0, "EU Name"=w770, "Full Scale SLPM"=w772, "Gas Index"=w769) -> ("Mass EU Value Out"=w767:dbl)  [unwired: 7 in]
            n279 = case shown="True" w777 {
              frame False {
                w800 = u8 0 ("Y Scale.Scale Fit")
                w808 = u8 0
                # "Auto Scale is Disabled"
                n280 = property on="Chart" class="WFChart (strict)"("Active Plot"=u32 0, "YScale.ScaleFit"=w808, "Active Plot"=u32 1, "YScale.ScaleFit"=w808, "Active Plot"=u32 2, "YScale.ScaleFit"=w808, "Active Plot"=u32 3, "YScale.ScaleFit"=w808, "Active Plot"=u32 4, "YScale.ScaleFit"=w808) -> ()  [unwired: 2 in, 2 out]
                n281 = property on="Chart" class="WFChart (strict)"("ActYScl"=0, "YScale.ScaleFit"=w800) -> ()  [unwired: 2 in, 2 out]
                n282 = property on="Chart" class="WFChart (strict)"("ActYScl"=2, "YScale.ScaleFit"=w800) -> ()  [unwired: 2 in, 2 out]
                n283 = property on="Chart" class="WFChart (strict)"("ActYScl"=1, "YScale.ScaleFit"=w800) -> ()  [unwired: 2 in, 2 out]
              }
              frame True {
                w810 = u8 2 ("Y Scale.Scale Fit")
                w814 = u8 2
                # "Auto Scale is Enabled"
                n284 = property on="Chart" class="WFChart (strict)"("Active Plot"=u32 0, "YScale.ScaleFit"=w814, "Active Plot"=u32 1, "YScale.ScaleFit"=w814, "Active Plot"=u32 2, "YScale.ScaleFit"=w814, "Active Plot"=u32 3, "YScale.ScaleFit"=w814, "Active Plot"=u32 4, "YScale.ScaleFit"=w814) -> ()  [unwired: 2 in, 2 out]
                n285 = property on="Chart" class="WFChart (strict)"("ActYScl"=0, "YScale.ScaleFit"=w810) -> ()  [unwired: 2 in, 2 out]
                n286 = property on="Chart" class="WFChart (strict)"("ActYScl"=2, "YScale.ScaleFit"=w810) -> ()  [unwired: 2 in, 2 out]
                n287 = property on="Chart" class="WFChart (strict)"("ActYScl"=1, "YScale.ScaleFit"=w810) -> ()  [unwired: 2 in, 2 out]
              }
            }
            n288 = property on="Temperature Units" class="CmbBox"() -> ("Value"=w763:string)  [unwired: 2 in, 2 out]
            n289 = call "Convert Celsius to Active Temp EU (SubVI).vi"("Celsius Value In"=60.0 ("Y Scale.Range:Minimum"), "EU Name"=w763) -> ("Temp. Value Out"=w761:dbl)  [unwired: 9 in]
            n290 = Build Array(w767, w761, w765) -> (w766:dbl[])
            n291 = for {
              tunnel: w766 -> [w798] mode=indexing
              i -> [w797]
              # "Set Y Scale Ranges to Maximum"
              n292 = To Long Integer(number=w797) -> (32bit integer=w796:i32)
              n293 = property on="Chart" class="WFChart (strict)"("ActYScl"=w796, "YScale.Maximum"=w798, "YScale.Minimum"=0.0 ("Y Scale.Range:Minimum")) -> ()  [unwired: 2 in, 2 out]
            }
            n294 = property on="Wait Message" class="Clust (strict)"(error in=w755, "Visible"=w788) -> (error out=w787:errorcluster)  [unwired: 1 in, 1 out]
            n295 = Unbundle(w790) -> ("Panel"=w789:refnum<vi>)  [unwired: 1 out]
            n296 = property class="Pnl"(reference=w789, error in=w787, "DeferPanUpdts"=w788) -> (error out=w786:errorcluster)  [unwired: 1 out]
          }
          frame 9, Default {
            # "Get Valve Output"
            # "Process Information Data Collection"
            n297 = property on="Setpoint Value" class="DigNum (strict)"() -> ("Value"=w886:dbl)  [unwired: 2 in, 2 out]
            n298 = call "Elapsed Time"("Set Start Time (s)"=0.0) -> ("Elapsed Time (s)"=w900:dbl)  [unwired: 11 in, 7 out]
            n299 = call "Read Process Information (SubVI).vi"("error in (no error)"=w896, "Address"=w871, "VISA Refnum in"=w897) -> ("error out"=w873:errorcluster, "PI String Array"=w892:T31, "VISA Refnum out"=w875:refnum<visa-resource-name>)  [unwired: 4 in, 2 out]
            n300 = And(x="Read Valve Output", y=w821) -> (x .and. y?=w820:bool)
            n301 = Format Into String(format string="%7.3f", initial string="", w886) -> (resulting string=w885:string)  [unwired: 1 in, 1 out]
            n302 = Reciprocal(x=w900) -> (1/x=→"Measurem.\nper second":dbl)
            n303 = Unbundle(w892) -> ("string array[0]"=w857:string, "string array[1]"=w891:string, "string array[2]"=w856:string, "string array[3]"=w850:string, "string array[4]"=w890:string, "string array[5]"=w889:string, "string array[6]"=w847:string, "string array[7]"=w846:string, "string array[8]"=w845:string, "string array[9]"=w839:string, "string array[10]"=w883:string)
            n304 = Fract/Exp String To Number(string=w850) -> (number=w853:dbl)  [unwired: 3 in, 1 out]
            n305 = To Double Precision Float(number=w853) -> (double precision float=w849:dbl)
            n306 = case shown="True" w820 {
              tunnel: w875 -> [w910 w920]
              tunnel: [w910 w919] -> w874
              tunnel: w873 -> [w909 w918]
              tunnel: [w909 w917] -> w872
              tunnel: w871 -> [w911 w915]
              tunnel: ["N/A" w916] -> w870
              tunnel: [w911 w915] -> w869
              frame False {
              }
              frame True {
                n307 = call "Send Read Write Command (SubVI).vi"("Search String"="VLV:", "Address"=w915, "error in (no error)"=w918, "Command"="READ,16", "Disable writing (T)"=TRUE, "VISA Refnum in"=w920) -> ("error out"=w917:errorcluster, "Response String"=w916:string, "VISA Refnum out"=w919:refnum<visa-resource-name>)  [unwired: 3 in]
              }
            }
            n308 = To Upper Case(1:w883) -> (0:w832:string)
            n309 = To Upper Case(1:w839) -> (0:w827:string)
            n310 = Bundle By Name(cluster=w852, "Current Volume"=w849) -> (w851:T19)
            n311 = Hexadecimal String To Number(string=w832, offset=2) -> (number=w829:u32)  [unwired: 1 in, 1 out]
            n312 = Hexadecimal String To Number(string=w827, offset=2) -> (number=w826:u32)  [unwired: 1 in, 1 out]
            n313 = To Unsigned Word Integer(number=w826) -> (unsigned 16bit integer=w825:u16)
            n314 = To Unsigned Word Integer(number=w829) -> (unsigned 16bit integer=w831:u16)
            n315 = Not Equal?(x=w839, y=w835) -> (x != y?=w840:bool)
            n316 = property on="Current Volume" class="DigNum (strict)"("Value"=w849) -> ()  [unwired: 2 in, 2 out]
            n317 = Unbundle By Name(w881) -> ("Mass EU"=w866:string, "Volum. EU"=w864:string)
            n318 = Greater?(x=w831, y=u16 0) -> (0:w882:bool)
            n319 = property on="Pressure Units" class="CmbBox"() -> ("Value"=w876:string)  [unwired: 2 in, 2 out]
            n320 = Greater?(x=w825, y=u16 0) -> (0:w884:bool)
            n321 = case shown="True" w840 {
              tunnel: w839 -> [_ w907]
              tunnel: [w904 w907] -> w838
              tunnel: w837 -> [w903 w906]
              tunnel: [w903 w905] -> w836
              tunnel: w835 -> [w904 _]
              frame False {
              }
              frame True {
                n322 = call "Update Alarm Events Indicators (SubVI).vi"("Alarm Events In"=w906, "AE Status String In"=w907) -> ("Alarm Events Out"=w905:T2)  [unwired: 9 in]
                n323 = local write "Alarm Events"(w905) -> ()
              }
            }
            n324 = property on="Mass Flow Units" class="CmbBox"() -> ("Value"=w879:string)  [unwired: 2 in, 2 out]
            n325 = property on="Temperature Units" class="CmbBox"() -> ("Value"=w877:string)  [unwired: 2 in, 2 out]
            n326 = call <vilib>:"Trim Whitespace.vi"("string"=w866) -> ("trimmed string"=w867:string)  [unwired: 1 in]
            n327 = call <vilib>:"Trim Whitespace.vi"("string"=w864) -> ("trimmed string"=w865:string)  [unwired: 1 in]
            n328 = Fract/Exp String To Number(string=w856) -> (number=w855:dbl)  [unwired: 3 in, 1 out]
            n329 = To Double Precision Float(number=w855) -> (double precision float=w854:dbl)
            n330 = call "Convert Mass Flow EU to Totalizer EU (SubVI).vi"("Mass Flow EU"=w879) -> ("Totalizer EU"=w878:string)  [unwired: 10 in]
            n331 = Bundle By Name(cluster=w859, "Current Volume"=w854) -> (w858:T20)
            n332 = property on="Current Volume" class="DigNum (strict)"("Value"=w854) -> ()  [unwired: 2 in, 2 out]
            n333 = Bundle(cluster=w863, "Mass Flow"=w857, "Volum. Flow"=w891, "Totalizer #1"=w856, "Totalizer #2"=w850, "Gas Temp."=w890, "Gas Pressure"=w889, "Flow"=w847, "Press."=w845, "Temp."=w846, "Alarm Events"=w839, "Diagnostic Events 2"=w883, "Set Point"=w885, "Valve Counts"=w870, "Alarm Ind"=w884, "Diagnostic Ind"=w882, "SP Units"=w867, "Valve Counts Units"="Counts", "Mass Flow Units"=w867, "Vol Flow Units"=w865, "Total1 Vol Units"=w878, "Total2 Vol Units"=w878, "Gas Temp Units"=w877, "Gas Press Units"=w876) -> (w841:T4)
            "Process Information" <- w841
            n334 = Unbundle By Name(w841) -> ("Flow"=w862:string)
            n335 = Unbundle By Name(w841) -> ("Press."=w861:string)
            n336 = Unbundle By Name(w841) -> ("Temp."=w860:string)
            n337 = Wait (ms)(milliseconds to wait="Update Time  [ms]") -> ()  [unwired: 1 out]
            n338 = property on="Status:" class="Str"("Value"=w862) -> ()  [unwired: 2 in, 2 out]
            n339 = property on="Status:" class="Str"("Value"=w861) -> ()  [unwired: 2 in, 2 out]
            n340 = property on="Status:" class="Str"("Value"=w860) -> ()  [unwired: 2 in, 2 out]
          }
        }
        n341 = Select(t=0, s=w180, f=w181) -> (s? t:f=w179:i32)
      }
      event Panel Close? {
        w923 = TRUE ("Discard?")
        # "Discard a panel close command and force the program to end. Forces references to be closed before exiting."
        n342 = event-data() -> ()  [unwired: 1 in, 4 out]
        n343 = event-data("Discard?"=w923) -> ()  [unwired: 1 in, 1 out]
      }
      event "Serial Configuration.Serial Port #": Value Change {
        # "Re-initialize State Machine to Zero"
        # "Close the VISA session and re-initialize it with the new COM port value. Resets the state machine to 0 to initialize the instrument."
        n344 = event-data() -> ("NewVal"=w945:refnum<visa-resource-name>)  [unwired: 1 in]
        n345 = VISA Close(VISA resource name=w948, error in (no error)=w947) -> (error out=w931:errorcluster)
        n346 = property on="Address" class="DigNum (strict)"() -> ("Value"=w942:u8)  [unwired: 2 in, 2 out]
        n347 = property on="RS-485" class="Bool (strict)"() -> ("Value"=w943:bool)  [unwired: 2 in, 2 out]
        n348 = property on="Baud Rate" class="Ring (strict)"() -> ("Value"=w944:T15)  [unwired: 2 in, 2 out]
        n349 = local read "Serial Configuration"() -> (w946:T16)
        n350 = Bundle By Name(cluster=w946, "Baud Rate"=w944, "Serial Port #"=w945, "RS-485"=w943, "Address"=w942) -> (w941:T16)
        n351 = control-ref of="Address"() -> (w930:refnum<vi>)
        n352 = call "Init COM Port (SubVI).vi"("error in (no error)"=w931, "Enable/Disable"=w940, "Serial Configuration"=w941, "Digital in"=w930) -> ("error out"=w938:errorcluster, "Address String"=w937:string, "VISA Refnum out"=w939:refnum<visa-resource-name>)  [unwired: 5 in]
      }
      event Value Change {
        # "Re-initialize State Machine to Zero"
        # "Changes the COM Port Baud Rate to the new value, and then it resets the state machine to 0 to initialize the device"
        n353 = event-data() -> ("NewVal"=w963:T15)  [unwired: 1 in]
        n354 = case shown="9600, Default" w963 {
          tunnel: [u32 300 ("Serial Settings:Baud Rate") u32 600 ("Serial Settings:Baud Rate") u32 1200 ("Serial Settings:Baud Rate") u32 2400 ("Serial Settings:Baud Rate") u32 4800 ("Serial Settings:Baud Rate") u32 9600 ("Serial Settings:Baud Rate") u32 19200 ("Serial Settings:Baud Rate") u32 38400 ("Serial Settings:Baud Rate")] -> w958
          frame 300 {
          }
          frame 600 {
          }
          frame 1200 {
          }
          frame 2400 {
          }
          frame 4800 {
          }
          frame 9600, Default {
          }
          frame 19200 {
          }
          frame 38400 {
          }
        }
        n355 = property class="Instr"(reference=w960, error in=w962, "Baud"=w958) -> (reference out=w959:refnum<visa-resource-name>, error out=w961:errorcluster)
      }
      event "Serial Configuration.Address": Value Change {
        # "Re-initialize State Machine to Zero"
        # "Changes the instrument RS485 Address to the new value, and then it resets the state machine to 0 to initialize the device"
        n356 = event-data() -> ("NewVal"=w985:u8)  [unwired: 1 in]
        n357 = VISA Close(VISA resource name=w983, error in (no error)=w982) -> (error out=w989:errorcluster)
        n358 = property on="RS-485" class="Bool (strict)"() -> ("Value"=w986:bool)  [unwired: 2 in, 2 out]
        n359 = property on="Baud Rate" class="Ring (strict)"() -> ("Value"=w988:T15)  [unwired: 2 in, 2 out]
        n360 = property on="Serial Port #" class="VISAName"() -> ("Value"=w987:refnum<visa-resource-name>)  [unwired: 2 in, 2 out]
        n361 = local read "Serial Configuration"() -> (w991:T16)
        n362 = Bundle By Name(cluster=w991, "Baud Rate"=w988, "Serial Port #"=w987, "RS-485"=w986, "Address"=w985) -> (w990:T16)
        n363 = control-ref of="Address"() -> (w972:refnum<vi>)
        n364 = call "Init COM Port (SubVI).vi"("error in (no error)"=w989, "Enable/Disable"=w984, "Serial Configuration"=w990, "Digital in"=w972) -> ("error out"=w981:errorcluster, "Address String"=w979:string, "VISA Refnum out"=w980:refnum<visa-resource-name>)  [unwired: 5 in]
      }
      event "Serial Configuration.RS-485": Value Change {
        # "Re-initialize State Machine to Zero"
        # "Changes the instrument Interface Type (RS485/RS232)  to the new value, and then it resets the state machine to 0 to initialize the device"
        n365 = event-data() -> ("NewVal"=w994:bool)  [unwired: 1 in]
        n366 = VISA Close(VISA resource name=w1006, error in (no error)=w1005) -> (error out=w1010:errorcluster)
        n367 = property on="Address" class="DigNum (strict)"() -> ("Value"=w995:u8)  [unwired: 2 in, 2 out]
        n368 = property on="Baud Rate" class="Ring (strict)"() -> ("Value"=w1009:T15)  [unwired: 2 in, 2 out]
        n369 = property on="Serial Port #" class="VISAName"() -> ("Value"=w1008:refnum<visa-resource-name>)  [unwired: 2 in, 2 out]
        n370 = local read "Serial Configuration"() -> (w1012:T16)
        n371 = Bundle By Name(cluster=w1012, "Baud Rate"=w1009, "Serial Port #"=w1008, "RS-485"=w994, "Address"=w995) -> (w1011:T16)
        n372 = control-ref of="Address"() -> (w993:refnum<vi>)
        n373 = call "Init COM Port (SubVI).vi"("error in (no error)"=w1010, "Enable/Disable"=w1007, "Serial Configuration"=w1011, "Digital in"=w993) -> ("error out"=w1004:errorcluster, "Address String"=w1002:string, "VISA Refnum out"=w1003:refnum<visa-resource-name>)  [unwired: 5 in]
      }
      event "Set Point Options.Setpoint Value": Value Change {
        # "Reset if\ncomm error"
        # "Compares old and new values of the Set Point and if value changed sends new value to the instrument. Reads new SP vaqlue and updates PI data on the front panel."
        n374 = event-data() -> ("NewVal"=w1042:dbl)  [unwired: 1 in]
        n375 = Not Equal?(x=w1042, y=w1046) -> (x != y?=w1043:bool)
        n376 = case shown="True" w1043 {
          tunnel: w1045 -> [w1048 w1054]
          tunnel: [w1048 w1053] -> w1040
          tunnel: w1044 -> [w1047 w1052]
          tunnel: [w1047 w1051] -> w1039
          tunnel: w1037 -> [_ w1050]
          tunnel: w1042 -> [_ w1049]
          frame False {
          }
          frame True {
            n377 = call "Process Set Point Command (SubVI).vi"("Setpoint"=w1049, "Address"=w1050, "error in (no error)"=w1052, "VISA Refnum in"=w1054) -> ("error out"=w1051:errorcluster, "VISA Refnum out"=w1053:refnum<visa-resource-name>)  [unwired: 5 in, 1 out]
          }
        }
        n378 = call "Process Set Point Command (SubVI).vi"("Setpoint"=-1.0, "Address"=w1037, "error in (no error)"=w1039, "VISA Refnum in"=w1040) -> ("error out"=w1028:errorcluster, "Setpoint Value Out"=w1025:string, "VISA Refnum out"=w1038:refnum<visa-resource-name>)  [unwired: 5 in]
        n379 = Fract/Exp String To Number(string=w1025) -> (number=w1024:dbl)  [unwired: 3 in, 1 out]
        n380 = property on="Set Point" class="Str"("Value"=w1025) -> ()  [unwired: 2 in, 2 out]
        n381 = To Double Precision Float(number=w1024) -> (double precision float=w1036:dbl)
        n382 = property on="Setpoint Value" class="DigNum (strict)"("Value"=w1036) -> ()  [unwired: 2 in, 2 out]
        n383 = property on="Update Time  [ms]" class="DigNum (strict)"() -> ("Value"=w1030:u32)  [unwired: 2 in, 2 out]
        n384 = Wait (ms)(milliseconds to wait=w1030) -> ()  [unwired: 1 out]
        n385 = Select(t=0, s=w1028, f=w1026) -> (s? t:f=w1027:i32)
      }
      event "Measuring Units.Mass Flow Units": Value Change {
        # "Update SP Precision and Maximum Value"
        # "Reset if\ncomm error"
        # "Compares old and new values of the Mass Flow EU and if value changed sends new value to the instrument. Updates Set Point value. Updates PI data on the front panel."
        n386 = event-data() -> ("OldVal"=w1091:string, "NewVal"=w1088:string)  [unwired: 1 in]
        n387 = property on="Chart: AutoScale Chart" class="Bool (strict)"() -> ("Value"=w1072:bool)  [unwired: 2 in, 2 out]
        n388 = property on="Update Time  [ms]" class="DigNum (strict)"() -> ("Value"=w1082:u32)  [unwired: 2 in, 2 out]
        n389 = Not Equal?(x=w1091, y=w1088) -> (x != y?=w1090:bool)
        n390 = Wait (ms)(milliseconds to wait=w1082) -> ()  [unwired: 1 out]
        n391 = case shown="True" w1090 {
          tunnel: w1094 -> [w1127 w1145]
          tunnel: [w1127 w1140] -> w1093
          tunnel: w1092 -> [w1126 w1144]
          tunnel: [w1126 w1138] -> w1086
          tunnel: w1089 -> [_ w1137]
          tunnel: w1088 -> [_ w1128]
          tunnel: w1083 -> [w1125 w1142]
          tunnel: [w1125 w1131] -> w1067
          tunnel: w1058 -> [_ w1136]
          tunnel: w1078 -> [w1124 w1135]
          tunnel: [w1124 w1134] -> w1071
          tunnel: [w1123 w1130] -> w1057
          tunnel: w1079 -> [w1123 w1129]
          frame False {
          }
          frame True {
            # "Process Ifo"
            # "Process Ifo"
            # "Set Point"
            # "Dev. Ifo"
            n392 = call "Process Mass Flow EU Command (SubVI).vi"("Mass Flow EU In"=w1128, "Address"=w1137, "error in (no error)"=w1144, "VISA Refnum in"=w1145) -> ("error out"=w1139:errorcluster, "Mass Flow EU Out"=w1133:string, "VISA Refnum out"=w1141:refnum<visa-resource-name>)  [unwired: 5 in]
            n393 = property on="Mass Flow Units" class="CmbBox"("Value"=w1133) -> ()  [unwired: 2 in, 2 out]
            n394 = property on="Mass EU" class="Str"("Value"=w1133) -> ()  [unwired: 2 in, 2 out]
            n395 = property on="Mass Flow EU 2" class="Str"("Value"=w1133) -> ()  [unwired: 2 in, 2 out]
            n396 = property on="Mass Flow Units" class="Str"("Value"=w1133) -> ()  [unwired: 2 in, 2 out]
            n397 = call "Convert Mass Flow EU to Totalizer EU (SubVI).vi"("Mass Flow EU"=w1133) -> ("Totalizer EU"=w1143:string)  [unwired: 10 in]
            n398 = property on="Total EU 1" class="Str"("Value"=w1143) -> ()  [unwired: 2 in, 2 out]
            n399 = property on="SP Units" class="Str"("Value"=w1133) -> ()  [unwired: 2 in, 2 out]
            n400 = Bundle By Name(cluster=w1142, "Mass Flow Units"=w1133) -> (w1132:T4)
            n401 = property on="Total EU 2" class="Str"("Value"=w1143) -> ()  [unwired: 2 in, 2 out]
            n402 = property on="Total EU 1" class="Str"("Value"=w1143) -> ()  [unwired: 2 in, 2 out]
            n403 = property on="Total EU 2" class="Str"("Value"=w1143) -> ()  [unwired: 2 in, 2 out]
            n404 = Bundle By Name(cluster=w1135, "Mass EU"=w1133) -> (w1134:T14)
            n405 = property on="Pulse Unit" class="Str"("Value"=w1143) -> ()  [unwired: 2 in, 2 out]
            n406 = case shown="True" w1136 {
              tunnel: w1141 -> [w1149 w1159]
              tunnel: [w1149 w1158] -> w1140
              tunnel: w1139 -> [w1148 w1157]
              tunnel: [w1148 w1156] -> w1138
              tunnel: w1137 -> [_ w1155]
              tunnel: w1132 -> [w1147 w1153]
              tunnel: [w1147 w1152] -> w1131
              tunnel: [w1146 w1150] -> w1130
              tunnel: w1129 -> [w1146 _]
              frame False {
              }
              frame True {
                n407 = call "Process Set Point Command (SubVI).vi"("Setpoint"=-1.0, "Address"=w1155, "error in (no error)"=w1157, "VISA Refnum in"=w1159) -> ("error out"=w1156:errorcluster, "Setpoint Value Out"=w1151:string, "VISA Refnum out"=w1158:refnum<visa-resource-name>)  [unwired: 5 in]
                n408 = Fract/Exp String To Number(string=w1151) -> (number=w1154:dbl)  [unwired: 3 in, 1 out]
                n409 = To Double Precision Float(number=w1154) -> (double precision float=w1150:dbl)
                n410 = property on="Setpoint Value" class="DigNum (strict)"("Value"=w1150) -> ()  [unwired: 2 in, 2 out]
                n411 = Bundle By Name(cluster=w1153, "Set Point"=w1151) -> (w1152:T4)
              }
            }
          }
        }
        n412 = Unbundle By Name(w1078) -> ("Full Scale Range"=w1074:string)
        n413 = property on="Selected Gas" class="CmbBox"() -> ("Value"=w1075:string)  [unwired: 2 in, 2 out]
        n414 = Unbundle By Name(w1067) -> ("Mass Flow Units"=w1077:string)
        n415 = call "Get Max Limit and Precision (SubVI).vi"("Gas Index"=w1075, "Full Scale SLPM"=w1074, "EU Name"=w1077) -> ("SP Max Limit"=w1073:dbl, "Mass EU Precision"=w1076:u32)  [unwired: 5 in, 1 out]
        n416 = property on="Setpoint Value" class="DigNum (strict)"("Precision"=w1076) -> ()  [unwired: 2 in, 2 out]
        n417 = property on="Setpoint Value" class="DigNum (strict)"("Maximum"=w1073) -> ()  [unwired: 2 in, 2 out]
        n418 = Unbundle By Name(w1067) -> ("Mass Flow Units"=w1066:string)
        n419 = property on="Pressure Units" class="CmbBox"() -> ("Value"=w1070:string)  [unwired: 2 in, 2 out]
        n420 = property on="Temperature Units" class="CmbBox"() -> ("Value"=w1069:string)  [unwired: 2 in, 2 out]
        n421 = call "Update Chart Scale Max Limit (SubVI).vi"("Device Information"=w1071, "Temp EU"=w1069, "Pressure EU"=w1070, "Mass Flow EU"=w1066) -> ("Array"=w1068:dbl[])  [unwired: 7 in]
        n422 = case shown="False" w1072 {
          tunnel: w1068 -> [w1095 _]
          frame False {
            w1096 = u8 0 ("Y Scale.Scale Fit")
            w1101 = u8 0 ("Y Scale.Scale Fit")
            # "Turn off auto-scaling"
            n423 = property on="Chart" class="WFChart (strict)"("Active Plot"=u32 0, "YScale.ScaleFit"=w1101, "Active Plot"=u32 1, "YScale.ScaleFit"=w1101, "Active Plot"=u32 2, "YScale.ScaleFit"=w1101, "Active Plot"=u32 3, "YScale.ScaleFit"=w1101, "Active Plot"=u32 4, "YScale.ScaleFit"=w1101) -> (error out=w1100:errorcluster)  [unwired: 2 in, 1 out]
            n424 = property on="Chart" class="WFChart (strict)"("ActYScl"=0, "YScale.ScaleFit"=w1096) -> ()  [unwired: 2 in, 2 out]
            n425 = property on="Chart" class="WFChart (strict)"("ActYScl"=2, "YScale.ScaleFit"=w1096) -> ()  [unwired: 2 in, 2 out]
            n426 = property on="Chart" class="WFChart (strict)"("ActYScl"=1, "YScale.ScaleFit"=w1096) -> ()  [unwired: 2 in, 2 out]
            n427 = for {
              tunnel: w1095 -> [w1111] mode=indexing
              shift-right: [w1110] -> _
              shift-left: w1100 -> [w1107]
              i -> [w1109]
              # "Set Y Scale Ranges to Maximum"
              n428 = To Long Integer(number=w1109) -> (32bit integer=w1108:i32)
              n429 = property on="Chart" class="WFChart (strict)"(error in=w1107, "ActYScl"=w1108, "YScale.Maximum"=w1111, "YScale.Minimum"=0.0 ("Y Scale.Range:Minimum")) -> (error out=w1110:errorcluster)  [unwired: 1 in, 1 out]
            }
          }
          frame True {
            w1113 = u8 2 ("Y Scale.Scale Fit")
            w1117 = u8 2 ("Y Scale.Scale Fit")
            # "AutoScale is true"
            n430 = property on="Chart" class="WFChart (strict)"("Active Plot"=u32 0, "YScale.ScaleFit"=w1117, "Active Plot"=u32 1, "YScale.ScaleFit"=w1117, "Active Plot"=u32 2, "YScale.ScaleFit"=w1117, "Active Plot"=u32 3, "YScale.ScaleFit"=w1117, "Active Plot"=u32 4, "YScale.ScaleFit"=w1117) -> ()  [unwired: 2 in, 2 out]
            n431 = property on="Chart" class="WFChart (strict)"("ActYScl"=0, "YScale.ScaleFit"=w1113) -> ()  [unwired: 2 in, 2 out]
            n432 = property on="Chart" class="WFChart (strict)"("ActYScl"=1, "YScale.ScaleFit"=w1113) -> ()  [unwired: 2 in, 2 out]
            n433 = property on="Chart" class="WFChart (strict)"("ActYScl"=2, "YScale.ScaleFit"=w1113) -> ()  [unwired: 2 in, 2 out]
          }
        }
        n434 = Select(t=0, s=w1086, f=w1084) -> (s? t:f=w1085:i32)
      }
      event "Measuring Units.Vol. Flow Units": Value Change {
        # "Reset if\ncomm error"
        # "Compares old and new values of the Volumetric Flow EU and if value changed sends new value to the instrument. Updates PI data on the front panel."
        n435 = event-data() -> ("OldVal"=w1186:string, "NewVal"=w1184:string)  [unwired: 1 in]
        n436 = Not Equal?(x=w1186, y=w1184) -> (x != y?=w1185:bool)
        n437 = case shown="True" w1185 {
          tunnel: w1190 -> [w1193 w1206]
          tunnel: [w1193 w1205] -> w1189
          tunnel: w1188 -> [w1192 w1204]
          tunnel: [w1192 w1203] -> w1176
          tunnel: w1187 -> [w1191 w1197]
          tunnel: w1184 -> [_ w1202]
          tunnel: w1183 -> [w1195 w1201]
          tunnel: [w1195 w1200] -> w1182
          tunnel: w1181 -> [w1194 w1199]
          tunnel: [w1194 w1198] -> w1180
          tunnel: [w1191 w1197] -> w1179
          frame False {
          }
          frame True {
            n438 = call "Process Vol Flow EU Command (SubVI).vi"("Vol Flow EU In"=w1202, "Address"=w1197, "error in (no error)"=w1204, "VISA Refnum in"=w1206) -> ("error out"=w1203:errorcluster, "Vol Flow EU Out"=w1196:string, "VISA Refnum out"=w1205:refnum<visa-resource-name>)  [unwired: 5 in]
            n439 = Bundle By Name(cluster=w1201, "Volum. EU"=w1196) -> (w1200:T14)
            n440 = property on="Volum. EU" class="Str"("Value"=w1196) -> ()  [unwired: 2 in, 2 out]
            n441 = property on="Vol. Flow Units" class="CmbBox"("Value"=w1196) -> ()  [unwired: 2 in, 2 out]
            n442 = Bundle By Name(cluster=w1199, "Vol Flow Units"=w1196) -> (w1198:T4)
          }
        }
        n443 = Select(t=0, s=w1176, f=w1175) -> (s? t:f=w1177:i32)
      }
      event "Measuring Units.Pressure Units": Value Change {
        # "Rescale Chart"
        # "Reset if\ncomm error"
        # "Compares old and new values of the Pressure EU and if value changed sends new value to the instrument. Updates PI data on the front panel."
        n444 = event-data() -> ("OldVal"=w1240:string, "NewVal"=w1230:string)  [unwired: 1 in]
        n445 = Not Equal?(x=w1240, y=w1230) -> (x != y?=w1233:bool)
        n446 = property on="Chart: AutoScale Chart" class="Bool (strict)"() -> ("Value"=w1217:bool)  [unwired: 2 in, 2 out]
        n447 = case shown="True" w1233 {
          tunnel: w1238 -> [w1272 w1281]
          tunnel: w1237 -> [w1271 w1280]
          tunnel: [w1272 w1279] -> w1236
          tunnel: [w1271 w1278] -> w1235
          tunnel: w1232 -> [w1269 w1277]
          tunnel: [w1269 w1277] -> w1231
          tunnel: w1230 -> [_ w1276]
          tunnel: w1229 -> [w1270 w1275]
          tunnel: [w1270 w1274] -> w1222
          frame False {
          }
          frame True {
            n448 = call "Process Pressure EU Command (SubVI).vi"("Pressure EU In"=w1276, "Address"=w1277, "error in (no error)"=w1280, "VISA Refnum in"=w1281) -> ("error out"=w1278:errorcluster, "Pressure EU Out"=w1273:string, "VISA Refnum out"=w1279:refnum<visa-resource-name>)  [unwired: 5 in]
            n449 = Bundle By Name(cluster=w1275, "Gas Press Units"=w1273) -> (w1274:T4)
          }
        }
        n450 = Unbundle By Name(w1222) -> ("Mass Flow Units"=w1223:string, "Gas Press Units"=w1221:string, "Gas Temp Units"=w1220:string)
        n451 = call "Update Chart Scale Max Limit (SubVI).vi"("Device Information"=w1219, "Temp EU"=w1220, "Pressure EU"=w1221, "Mass Flow EU"=w1223) -> ("Array"=w1218:dbl[])  [unwired: 7 in]
        n452 = case shown="False" w1217 {
          tunnel: w1218 -> [w1241 _]
          frame False {
            w1242 = u8 0 ("Y Scale.Scale Fit")
            w1247 = u8 0 ("Y Scale.Scale Fit")
            # "Turn off auto-scaling"
            n453 = property on="Chart" class="WFChart (strict)"("Active Plot"=u32 0, "YScale.ScaleFit"=w1247, "Active Plot"=u32 1, "YScale.ScaleFit"=w1247, "Active Plot"=u32 2, "YScale.ScaleFit"=w1247, "Active Plot"=u32 3, "YScale.ScaleFit"=w1247, "Active Plot"=u32 4, "YScale.ScaleFit"=w1247) -> (error out=w1246:errorcluster)  [unwired: 2 in, 1 out]
            n454 = property on="Chart" class="WFChart (strict)"("ActYScl"=0, "YScale.ScaleFit"=w1242) -> ()  [unwired: 2 in, 2 out]
            n455 = property on="Chart" class="WFChart (strict)"("ActYScl"=2, "YScale.ScaleFit"=w1242) -> ()  [unwired: 2 in, 2 out]
            n456 = property on="Chart" class="WFChart (strict)"("ActYScl"=1, "YScale.ScaleFit"=w1242) -> ()  [unwired: 2 in, 2 out]
            n457 = for {
              tunnel: w1241 -> [w1257] mode=indexing
              shift-right: [w1256] -> _
              shift-left: w1246 -> [w1253]
              i -> [w1255]
              # "Set Y Scale Ranges to Maximum"
              n458 = To Long Integer(number=w1255) -> (32bit integer=w1254:i32)
              n459 = property on="Chart" class="WFChart (strict)"(error in=w1253, "ActYScl"=w1254, "YScale.Maximum"=w1257, "YScale.Minimum"=0.0 ("Y Scale.Range:Minimum")) -> (error out=w1256:errorcluster)  [unwired: 1 in, 1 out]
            }
          }
          frame True {
            w1259 = u8 2 ("Y Scale.Scale Fit")
            w1263 = u8 2 ("Y Scale.Scale Fit")
            # "AutoScale is true"
            n460 = property on="Chart" class="WFChart (strict)"("Active Plot"=u32 0, "YScale.ScaleFit"=w1263, "Active Plot"=u32 1, "YScale.ScaleFit"=w1263, "Active Plot"=u32 2, "YScale.ScaleFit"=w1263, "Active Plot"=u32 3, "YScale.ScaleFit"=w1263, "Active Plot"=u32 4, "YScale.ScaleFit"=w1263) -> ()  [unwired: 2 in, 2 out]
            n461 = property on="Chart" class="WFChart (strict)"("ActYScl"=0, "YScale.ScaleFit"=w1259) -> ()  [unwired: 2 in, 2 out]
            n462 = property on="Chart" class="WFChart (strict)"("ActYScl"=1, "YScale.ScaleFit"=w1259) -> ()  [unwired: 2 in, 2 out]
            n463 = property on="Chart" class="WFChart (strict)"("ActYScl"=2, "YScale.ScaleFit"=w1259) -> ()  [unwired: 2 in, 2 out]
          }
        }
        n464 = Select(t=0, s=w1235, f=w1226) -> (s? t:f=w1234:i32)
      }
      event "Chart: Adjust Scale": Value Change {
        w1305 = u8 0 ("Y Scale.Scale Fit")
        w1309 = u8 0 ("Y Scale.Scale Fit")
        # "Manual Chart Scale Settings"
        # "Reset if\ncomm error"
        # "Compares old and new values of the Pressure EU and if value changed sends new value to the instrument. Updates PI data on the front panel."
        n465 = event-data() -> ()  [unwired: 1 in, 1 out]
        n466 = property on="Chart" class="WFChart (strict)"(error in=w1294, "Active Plot"=u32 0, "YScale.ScaleFit"=w1309, "Active Plot"=u32 1, "YScale.ScaleFit"=w1309, "Active Plot"=u32 2, "YScale.ScaleFit"=w1309, "Active Plot"=u32 3, "YScale.ScaleFit"=w1309, "Active Plot"=u32 4, "YScale.ScaleFit"=w1309) -> (error out=w1304:errorcluster)  [unwired: 1 in, 1 out]
        n467 = property on="Chart" class="WFChart (strict)"(error in=w1304, "ActYScl"=0, "YScale.ScaleFit"=w1305) -> (error out=w1303:errorcluster)  [unwired: 1 in, 1 out]
        n468 = property on="Chart" class="WFChart (strict)"(error in=w1303, "ActYScl"=1, "YScale.ScaleFit"=w1305) -> (error out=w1302:errorcluster)  [unwired: 1 in, 1 out]
        n469 = property on="Chart" class="WFChart (strict)"(error in=w1302, "ActYScl"=2, "YScale.ScaleFit"=w1305) -> (error out=w1293:errorcluster)  [unwired: 1 in, 1 out]
        n470 = call <vilib>:"Three Button Dialog.vi"("Allow user to close window? (TRUE)"=FALSE, "Window Title (\"\")"="Scale Adjustment Options" ("Window Title (\"\")"), "Right Button Text (\"Cancel\")"="Cancel" ("Left Button Text (\"Yes\")"), "Center Button Text (\"No\")"="Fit scales to current data" ("Left Button Text (\"Yes\")"), "Left Button Text (\"Yes\")"="Adjust scales manually" ("Left Button Text (\"Yes\")"), "message"="Adjust scales manually, or fit scales to current data?") -> ("Which Button?"=w1295:T32)  [unwired: 5 in]
        n471 = case shown="\"Left Button\", Default" w1295 {
          tunnel: w1293 -> [w1326 w1335 w1350]
          tunnel: [w1326 w1336 w1350] -> w1292
          frame "Left Button", Default {
            # "Adjust scales manually"
            n472 = call "Manual Scale Adjustment Menu.vi"() -> ("Scale Minimum"=w1327:dbl, "Scale Maximum"=w1328:dbl, "Active Y scale"=w1329:u32, "Request Canceled"=w1330:bool)  [unwired: 7 in, 1 out]
            n473 = case shown="False" w1330 {
              tunnel: w1329 -> [w1331 _]
              tunnel: w1328 -> [w1334 _]
              tunnel: w1327 -> [w1333 _]
              frame False {
                # "Adjust scales if false"
                n474 = To Long Integer(number=w1331) -> (32bit integer=w1332:i32)
                n475 = property on="Chart" class="WFChart (strict)"("ActYScl"=w1332, "YScale.Maximum"=w1334, "YScale.Minimum"=w1333) -> ()  [unwired: 2 in, 2 out]
              }
              frame True {
                # "request was aborted"
              }
            }
          }
          frame "Center Button" {
            w1340 = u8 1 ("Y Scale.Scale Fit")
            w1344 = u8 1 ("Y Scale.Scale Fit")
            # "Fit scales to current data"
            n476 = property on="Chart" class="WFChart (strict)"(error in=w1335, "Active Plot"=u32 0, "YScale.ScaleFit"=w1344, "Active Plot"=u32 1, "YScale.ScaleFit"=w1344, "Active Plot"=u32 2, "YScale.ScaleFit"=w1344, "Active Plot"=u32 3, "YScale.ScaleFit"=w1344, "Active Plot"=u32 4, "YScale.ScaleFit"=w1344) -> (error out=w1337:errorcluster)  [unwired: 1 in, 1 out]
            n477 = property on="Chart" class="WFChart (strict)"(error in=w1337, "ActYScl"=0, "YScale.ScaleFit"=w1340) -> (error out=w1339:errorcluster)  [unwired: 1 in, 1 out]
            n478 = property on="Chart" class="WFChart (strict)"(error in=w1339, "ActYScl"=1, "YScale.ScaleFit"=w1340) -> (error out=w1338:errorcluster)  [unwired: 1 in, 1 out]
            n479 = property on="Chart" class="WFChart (strict)"(error in=w1338, "ActYScl"=2, "YScale.ScaleFit"=w1340) -> (error out=w1336:errorcluster)  [unwired: 1 in, 1 out]
          }
          frame "Right Button" {
            # "Request was aborted"
          }
        }
        n480 = Select(t=0, s=w1292, f=w1319) -> (s? t:f=w1323:i32)
      }
      event "Measuring Units.Temperature Units": Value Change {
        # "Rescale Chart"
        # "Reset if\ncomm error"
        # "Compares old and new values of the Temperature EU and if value changed sends new value to the instrument. Updates PI data on the front panel."
        n481 = event-data() -> ("OldVal"=w1384:string, "NewVal"=w1374:string)  [unwired: 1 in]
        n482 = property on="Chart: AutoScale Chart" class="Bool (strict)"() -> ("Value"=w1363:bool)  [unwired: 2 in, 2 out]
        n483 = Not Equal?(x=w1384, y=w1374) -> (x != y?=w1377:bool)
        n484 = case shown="True" w1377 {
          tunnel: w1382 -> [w1416 w1422]
          tunnel: w1381 -> [w1415 w1421]
          tunnel: [w1416 w1420] -> w1380
          tunnel: [w1415 w1419] -> w1379
          tunnel: w1376 -> [w1413 w1425]
          tunnel: [w1413 w1425] -> w1375
          tunnel: w1374 -> [_ w1418]
          tunnel: w1373 -> [w1414 w1424]
          tunnel: [w1414 w1423] -> w1362
          frame False {
          }
          frame True {
            n485 = call "Process Temperature EU Command (SubVI).vi"("Temp. EU In"=w1418, "error in (no error)"=w1421, "VISA Refnum in"=w1422) -> ("error out"=w1419:errorcluster, "Temp. EU Out"=w1417:string, "VISA Refnum out"=w1420:refnum<visa-resource-name>)  [unwired: 6 in]
            n486 = Bundle By Name(cluster=w1424, "Gas Temp Units"=w1417) -> (w1423:T4)
          }
        }
        n487 = Unbundle By Name(w1362) -> ("Mass Flow Units"=w1367:string, "Gas Press Units"=w1366:string, "Gas Temp Units"=w1365:string)
        n488 = call "Update Chart Scale Max Limit (SubVI).vi"("Device Information"=w1361, "Temp EU"=w1365, "Pressure EU"=w1366, "Mass Flow EU"=w1367) -> ("Array"=w1364:dbl[])  [unwired: 7 in]
        n489 = case shown="False" w1363 {
          tunnel: w1364 -> [w1385 _]
          frame False {
            w1386 = u8 0 ("Y Scale.Scale Fit")
            w1391 = u8 0 ("Y Scale.Scale Fit")
            # "Turn off auto-scaling"
            n490 = property on="Chart" class="WFChart (strict)"("Active Plot"=u32 0, "YScale.ScaleFit"=w1391, "Active Plot"=u32 1, "YScale.ScaleFit"=w1391, "Active Plot"=u32 2, "YScale.ScaleFit"=w1391, "Active Plot"=u32 3, "YScale.ScaleFit"=w1391, "Active Plot"=u32 4, "YScale.ScaleFit"=w1391) -> (error out=w1390:errorcluster)  [unwired: 2 in, 1 out]
            n491 = property on="Chart" class="WFChart (strict)"("ActYScl"=0, "YScale.ScaleFit"=w1386) -> ()  [unwired: 2 in, 2 out]
            n492 = property on="Chart" class="WFChart (strict)"("ActYScl"=2, "YScale.ScaleFit"=w1386) -> ()  [unwired: 2 in, 2 out]
            n493 = property on="Chart" class="WFChart (strict)"("ActYScl"=1, "YScale.ScaleFit"=w1386) -> ()  [unwired: 2 in, 2 out]
            n494 = for {
              tunnel: w1385 -> [w1401] mode=indexing
              shift-right: [w1400] -> _
              shift-left: w1390 -> [w1397]
              i -> [w1399]
              # "Set Y Scale Ranges to Maximum"
              n495 = To Long Integer(number=w1399) -> (32bit integer=w1398:i32)
              n496 = property on="Chart" class="WFChart (strict)"(error in=w1397, "ActYScl"=w1398, "YScale.Maximum"=w1401, "YScale.Minimum"=0.0 ("Y Scale.Range:Minimum")) -> (error out=w1400:errorcluster)  [unwired: 1 in, 1 out]
            }
          }
          frame True {
            w1403 = u8 2 ("Y Scale.Scale Fit")
            w1407 = u8 2 ("Y Scale.Scale Fit")
            # "AutoScale is true"
            n497 = property on="Chart" class="WFChart (strict)"("Active Plot"=u32 0, "YScale.ScaleFit"=w1407, "Active Plot"=u32 1, "YScale.ScaleFit"=w1407, "Active Plot"=u32 2, "YScale.ScaleFit"=w1407, "Active Plot"=u32 3, "YScale.ScaleFit"=w1407, "Active Plot"=u32 4, "YScale.ScaleFit"=w1407) -> ()  [unwired: 2 in, 2 out]
            n498 = property on="Chart" class="WFChart (strict)"("ActYScl"=0, "YScale.ScaleFit"=w1403) -> ()  [unwired: 2 in, 2 out]
            n499 = property on="Chart" class="WFChart (strict)"("ActYScl"=1, "YScale.ScaleFit"=w1403) -> ()  [unwired: 2 in, 2 out]
            n500 = property on="Chart" class="WFChart (strict)"("ActYScl"=2, "YScale.ScaleFit"=w1403) -> ()  [unwired: 2 in, 2 out]
          }
        }
        n501 = Select(t=0, s=w1379, f=w1372) -> (s? t:f=w1378:i32)
      }
      event "Set Point Options.Setpoint Source": Value Change {
        # "Reset if\ncomm error"
        # "Compares old and new values of the Set Point Source and if value changed sends new value to the instrument. Disables Set Point Value control for Analog and PSP sources."
        n502 = event-data() -> ("OldVal"=w1457:string, "NewVal"=w1446:string)  [unwired: 1 in]
        n503 = Not Equal?(x=w1457, y=w1446) -> (x != y?=w1449:bool)
        n504 = property on="Update Time  [ms]" class="DigNum (strict)"() -> ("Value"=w1440:u32)  [unwired: 2 in, 2 out]
        n505 = case shown="True" w1442 {
          tunnel: w1455 -> [w1461 w1475]
          tunnel: w1454 -> [w1460 w1474]
          tunnel: [w1461 w1473] -> w1453
          tunnel: [w1460 w1472] -> w1452
          tunnel: w1449 -> [_ w1471]
          tunnel: w1448 -> [w1462 w1470]
          tunnel: [w1462 w1469] -> w1447
          tunnel: w1446 -> [_ w1468]
          tunnel: w1441 -> [_ w1467]
          tunnel: w1439 -> [w1459 w1466]
          tunnel: [w1459 w1465] -> w1438
          tunnel: [w1458 w1464] -> w1437
          tunnel: w1436 -> [w1458 w1463]
          frame False {
          }
          frame True {
            n506 = case shown="True" w1471 {
              tunnel: w1475 -> [w1480 w1508]
              tunnel: w1474 -> [w1479 w1507]
              tunnel: [w1480 w1490] -> w1473
              tunnel: [w1479 w1488] -> w1472
              tunnel: w1470 -> [w1478 w1487]
              tunnel: [w1478 w1487] -> w1469
              tunnel: w1468 -> [_ w1506]
              tunnel: w1467 -> [_ w1501]
              tunnel: w1466 -> [w1477 w1484]
              tunnel: [w1477 w1483] -> w1465
              tunnel: [w1476 w1481] -> w1464
              tunnel: w1463 -> [w1476 _]
              frame False {
              }
              frame True {
                # "Update Set Point value as well if Set Point Source was changed."
                n507 = call "Process Set Point Source Command (SubVI).vi"("Set Point Source In"=w1506, "Address"=w1487, "error in (no error)"=w1507, "VISA Refnum in"=w1508) -> ("error out"=w1489:errorcluster, "Setpoint Source Out"=w1493:string, "VISA Refnum out"=w1491:refnum<visa-resource-name>)  [unwired: 5 in]
                n508 = String Subset(string=w1493, offset (0)=0, length (rest)=1) -> (substring=w1492:string)
                n509 = Unbundle(w1501) -> ("Enabled"=w1500:T26, "Disabled and Grayed Out"=w1499:T26)
                n510 = Equal?(x=w1492, y="A") -> (x = y?=w1502:bool)
                n511 = Equal?(x=w1492, y="P") -> (x = y?=w1503:bool)
                n512 = Or(x=w1502, y=w1503) -> (x .or. y?=w1498:bool)
                n513 = Not(x=w1498) -> (.not. x?=w1497:bool)
                n514 = Select(t=w1500, s=w1497, f=w1499) -> (s? t:f=w1496:T26)
                n515 = property on="Setpoint Value" class="DigNum (strict)"("DisabledEnum"=w1496) -> ()  [unwired: 2 in, 2 out]
                n516 = call "Process Set Point Command (SubVI).vi"("Setpoint"=-1.0, "Address"=w1487, "error in (no error)"=w1489, "VISA Refnum in"=w1491) -> ("error out"=w1488:errorcluster, "Setpoint Value Out"=w1482:string, "VISA Refnum out"=w1490:refnum<visa-resource-name>)  [unwired: 5 in]
                n517 = Fract/Exp String To Number(string=w1482) -> (number=w1485:dbl)  [unwired: 3 in, 1 out]
                n518 = Bundle By Name(cluster=w1484, "Set Point"=w1482) -> (w1483:T4)
                n519 = To Double Precision Float(number=w1485) -> (double precision float=w1481:dbl)
                n520 = property on="Setpoint Value" class="DigNum (strict)"("Value"=w1481) -> ()  [unwired: 2 in, 2 out]
              }
            }
          }
        }
        n521 = Wait (ms)(milliseconds to wait=w1440) -> ()  [unwired: 1 out]
        n522 = Select(t=0, s=w1452, f=w1450) -> (s? t:f=w1451:i32)
      }
      event "Set Point Options.Valve Mode": Value Change {
        # "Reset if\ncomm error"
        # "Sends new value of Valve Mode to the instrument. If new value is \"Open\" prompts user with warning message regarding differential pressure limits."
        n523 = event-data() -> ()  [unwired: 1 in, 2 out]
        n524 = case shown="True" w1533 {
          tunnel: w1531 -> [w1535 w1549]
          tunnel: w1530 -> [w1534 w1548]
          tunnel: [w1535 w1547] -> w1529
          tunnel: [w1534 w1546] -> w1528
          tunnel: [w1536 w1545] -> w1524
          tunnel: w1525 -> [w1536 w1545]
          frame False {
          }
          frame True {
            n525 = Unbundle By Name("Set Point Options") -> ("Valve Mode"=w1540:string)
            n526 = Equal?(x=w1540, y="O") -> (x = y?=w1543:bool)
            n527 = case shown="True" w1543 {
              tunnel: w1540 -> [w1550 w1556]
              tunnel: [w1550 w1554] -> w1539
              tunnel: "Are You Sure? Excessive differential pressure may damage\n instrument pressure sensors! Make sure the excessive flow \nwill not create differential pressure across instrument which \nexceeds maximum differential pressure limit for this model." -> [_ w1552]
              tunnel: "Open Valve" -> [_ w1551]
              frame False {
              }
              frame True {
                n528 = Two Button Dialog(message=w1552, 2:w1551) -> (T button?=w1553:bool)  [unwired: 1 in]
                n529 = Select(t=w1556, s=w1553, f="") -> (s? t:f=w1554:string)
              }
            }
            n530 = call "Process Valve Mode Command (SubVI).vi"("Valve Mode In"=w1539, "Address"=w1545, "error in (no error)"=w1548, "VISA Refnum in"=w1549) -> ("error out"=w1546:errorcluster, "Valve Mode Out"=w1537:string, "VISA Refnum out"=w1547:refnum<visa-resource-name>)  [unwired: 5 in]
            n531 = property on="Valve Mode" class="CmbBox"("Value"=w1537) -> ()  [unwired: 2 in, 2 out]
          }
        }
        n532 = Select(t=0, s=w1528, f=w1526) -> (s? t:f=w1527:i32)
      }
      event "Selected Gas": Value Change {
        # "Update SP Precision and Maximum Value"
        # "Reset if\ncomm error"
        # "Sends new Gas selection to the instrument and updates device information claster."
        n533 = event-data() -> ()  [unwired: 1 in, 2 out]
        n534 = call "Process Gas Select Command (SubVI).vi"("Gas Select In"="Selected Gas", "Address"=w1580, "error in (no error)"=w1585, "VISA Refnum in"=w1587) -> ("error out"=w1582:errorcluster, "Gas Select Out"=w1570:string, "VISA Refnum out"=w1586:refnum<visa-resource-name>)  [unwired: 5 in]
        n535 = Unbundle By Name(w1571) -> ("Full Scale Range"=w1572:string)
        n536 = Unbundle By Name(w1569) -> ("Mass Flow Units"=w1573:string)
        n537 = property on="Selected Gas" class="Str"("Value"=w1570) -> ()  [unwired: 2 in, 2 out]
        n538 = Bundle By Name(cluster=w1571, "Selected Gas"=w1570) -> (w1574:T14)
        n539 = call "Get Max Limit and Precision (SubVI).vi"("Gas Index"=w1570, "Full Scale SLPM"=w1572, "EU Name"=w1573) -> ("SP Max Limit"=w1568:dbl, "Mass EU Precision"=w1567:u32)  [unwired: 5 in, 1 out]
        n540 = property on="Setpoint Value" class="DigNum (strict)"("Precision"=w1567) -> ()  [unwired: 2 in, 2 out]
        n541 = property on="Setpoint Value" class="DigNum (strict)"("Maximum"=w1568) -> ()  [unwired: 2 in, 2 out]
        n542 = Select(t=0, s=w1582, f=w1581) -> (s? t:f=w1583:i32)
      }
      event "SS Relay Assignment": Value Change {
        # "Reset if\ncomm error"
        # "Sends new SSR assignment to the instrument."
        n543 = event-data() -> ()  [unwired: 1 in, 2 out]
        n544 = call "Process SSR Command (SubVI).vi"("SSR Settings In"="SS Relay Assignment", "Address"=w1601, "error in (no error)"=w1602, "VISA Refnum in"=w1605) -> ("error out"=w1603:errorcluster, "SSR Settings Out"=w1599:string, "VISA Refnum out"=w1604:refnum<visa-resource-name>)  [unwired: 5 in]
        n545 = property on="SS Relay Assignment" class="CmbBox"("Value"=w1599) -> ()  [unwired: 2 in, 2 out]
        n546 = Select(t=0, s=w1603, f=w1611) -> (s? t:f=w1612:i32)
      }
      event "Chart: Mass Flow", "Chart: Volum Flow", "Chart: Set Point", "Chart: Pressure", "Chart: Temperature": Value Change {
        # "Reset if\ncomm error"
        # "Adjust which variables are displayed in the chart, and check the communication to the instrument"
        n547 = event-data() -> ()  [unwired: 1 in, 6 out]
        n548 = property on="Chart" class="WFChart (strict)"("Active Plot"=u32 0, "Plot.Visible?"="Chart: Mass Flow", "Active Plot"=u32 1, "Plot.Visible?"="Chart: Volum Flow", "Active Plot"=u32 2, "Plot.Visible?"="Chart: Set Point", "Active Plot"=u32 3, "Plot.Visible?"="Chart: Temperature", "Active Plot"=u32 4, "Plot.Visible?"="Chart: Pressure") -> ()  [unwired: 2 in, 2 out]
        n549 = Select(t=0, s=w1634, f=w1643) -> (s? t:f=w1644:i32)
      }
      event "Chart: AutoScale Chart": Value Change {
        # "Reset if\ncomm error"
        # "Toggles auto scale in the chart, and check the communication to the instrument"
        n550 = event-data() -> ()  [unwired: 1 in, 6 out]
        n551 = property on="Pressure Units" class="CmbBox"() -> ("Value"=w1657:string)  [unwired: 2 in, 2 out]
        n552 = property on="Temperature Units" class="CmbBox"() -> ("Value"=w1656:string)  [unwired: 2 in, 2 out]
        n553 = property on="Mass Flow Units" class="CmbBox"() -> ("Value"=w1658:string)  [unwired: 2 in, 2 out]
        n554 = call "Update Chart Scale Max Limit (SubVI).vi"("Device Information"=w1663, "Temp EU"=w1656, "Pressure EU"=w1657, "Mass Flow EU"=w1658) -> ("Array"=w1661:dbl[])  [unwired: 7 in]
        n555 = case shown="False" "Chart: AutoScale Chart" {
          tunnel: w1661 -> [w1681 _]
          tunnel: w1660 -> [w1680 w1698]
          tunnel: [w1679 w1698] -> w1659
          frame False {
            w1674 = u8 0 ("Y Scale.Scale Fit")
            w1682 = u8 0 ("Y Scale.Scale Fit")
            # "Turn off auto-scaling"
            n556 = property on="Chart" class="WFChart (strict)"(error in=w1680, "Active Plot"=u32 0, "YScale.ScaleFit"=w1682, "Active Plot"=u32 1, "YScale.ScaleFit"=w1682, "Active Plot"=u32 2, "YScale.ScaleFit"=w1682, "Active Plot"=u32 3, "YScale.ScaleFit"=w1682, "Active Plot"=u32 4, "YScale.ScaleFit"=w1682) -> (error out=w1678:errorcluster)  [unwired: 1 in, 1 out]
            n557 = property on="Chart" class="WFChart (strict)"("ActYScl"=0, "YScale.ScaleFit"=w1674) -> ()  [unwired: 2 in, 2 out]
            n558 = property on="Chart" class="WFChart (strict)"("ActYScl"=2, "YScale.ScaleFit"=w1674) -> ()  [unwired: 2 in, 2 out]
            n559 = property on="Chart" class="WFChart (strict)"("ActYScl"=1, "YScale.ScaleFit"=w1674) -> ()  [unwired: 2 in, 2 out]
            n560 = for {
              tunnel: w1681 -> [w1692] mode=indexing
              shift-right: [w1691] -> w1679
              shift-left: w1678 -> [w1688]
              i -> [w1690]
              # "Set Y Scale Ranges to Maximum"
              n561 = To Long Integer(number=w1690) -> (32bit integer=w1689:i32)
              n562 = property on="Chart" class="WFChart (strict)"(error in=w1688, "ActYScl"=w1689, "YScale.Maximum"=w1692, "YScale.Minimum"=0.0 ("Y Scale.Range:Minimum")) -> (error out=w1691:errorcluster)  [unwired: 1 in, 1 out]
            }
          }
          frame True {
            w1694 = u8 2 ("Y Scale.Scale Fit")
            w1699 = u8 2 ("Y Scale.Scale Fit")
            # "AutoScale is true"
            n563 = property on="Chart" class="WFChart (strict)"("Active Plot"=u32 0, "YScale.ScaleFit"=w1699, "Active Plot"=u32 1, "YScale.ScaleFit"=w1699, "Active Plot"=u32 2, "YScale.ScaleFit"=w1699, "Active Plot"=u32 3, "YScale.ScaleFit"=w1699, "Active Plot"=u32 4, "YScale.ScaleFit"=w1699) -> ()  [unwired: 2 in, 2 out]
            n564 = property on="Chart" class="WFChart (strict)"("ActYScl"=0, "YScale.ScaleFit"=w1694) -> ()  [unwired: 2 in, 2 out]
            n565 = property on="Chart" class="WFChart (strict)"("ActYScl"=1, "YScale.ScaleFit"=w1694) -> ()  [unwired: 2 in, 2 out]
            n566 = property on="Chart" class="WFChart (strict)"("ActYScl"=2, "YScale.ScaleFit"=w1694) -> ()  [unwired: 2 in, 2 out]
          }
        }
        n567 = Select(t=0, s=w1659, f=w1671) -> (s? t:f=w1672:i32)
      }
      event "Analog Output": Value Change {
        # "Reset if\ncomm error"
        # "Sends new Analog Output selection to the instrument and updates device information claster."
        n568 = event-data() -> ()  [unwired: 1 in, 2 out]
        n569 = call "Process Analog Output Command (SubVI).vi"("Analog Out Mode In"="Analog Output", "Address"=w1720, "error in (no error)"=w1721, "VISA Refnum in"=w1722) -> ("error out"=w1724:errorcluster, "Analog Out Mode Out"=w1718:string, "VISA Refnum out"=w1723:refnum<visa-resource-name>)  [unwired: 5 in]
        n570 = case shown="\"0\", Default" w1718 {
          tunnel: ["0-5Vdc" "0-10Vdc" "4-20mA"] -> w1715
          frame "0", Default {
          }
          frame "1" {
          }
          frame "2" {
          }
        }
        n571 = property on="Analog Output" class="CmbBox"("Value"=w1718) -> ()  [unwired: 2 in, 2 out]
        n572 = property on="A Output" class="Str"("Value"=w1715) -> ()  [unwired: 2 in, 2 out]
        n573 = Bundle By Name(cluster=w1717, "A Output"=w1715) -> (w1716:T14)
        n574 = Select(t=0, s=w1724, f=w1730) -> (s? t:f=w1731:i32)
      }
      event "Analog Input": Value Change {
        # "Reset if\ncomm error"
        # "Sends new Analog Input selection to the instrument and updates device information claster."
        n575 = event-data() -> ()  [unwired: 1 in, 2 out]
        n576 = case shown="True" w1747 {
          tunnel: w1754 -> [w1764 w1775]
          tunnel: [w1764 w1774] -> w1753
          tunnel: w1752 -> [w1763 w1772]
          tunnel: w1751 -> [w1762 w1771]
          tunnel: [w1762 w1770] -> w1750
          tunnel: [w1763 w1769] -> w1749
          tunnel: w1748 -> [w1765 w1766]
          tunnel: [w1765 w1766] -> w1746
          frame False {
          }
          frame True {
            n577 = call "Process Analog Input Command (SubVI).vi"("Analog Inp Mode In"="Analog Input", "Address"=w1766, "error in (no error)"=w1771, "VISA Refnum in"=w1772) -> ("error out"=w1770:errorcluster, "Analog Inp Mode Out"=w1767:string, "VISA Refnum out"=w1769:refnum<visa-resource-name>)  [unwired: 5 in]
            n578 = property on="Analog Input" class="CmbBox"("Value"=w1767) -> ()  [unwired: 2 in, 2 out]
            n579 = case shown="\"0\", Default" w1767 {
              tunnel: ["0-5Vdc" "0-10Vdc" "4-20mA"] -> w1773
              frame "0", Default {
              }
              frame "1" {
              }
              frame "2" {
              }
            }
            n580 = property on="A Input" class="Str"("Value"=w1773) -> ()  [unwired: 2 in, 2 out]
            n581 = Bundle By Name(cluster=w1775, "A Input"=w1773) -> (w1774:T14)
          }
        }
        n582 = Select(t=0, s=w1750, f=w1759) -> (s? t:f=w1760:i32)
      }
      event "Totalizer #1 Options.Reset Totalizer": Value Change {
        # "Reset if\ncomm error"
        # "Performs Totalizer#1 Reset to Zero Command"
        n583 = event-data() -> ("NewVal"=w1788:bool)  [unwired: 1 in, 1 out]
        n584 = Equal?(x=TRUE, y=w1788) -> (x = y?=w1801:bool)
        n585 = case shown="True" w1801 {
          tunnel: w1805 -> [w1808 w1815]
          tunnel: w1804 -> [w1807 w1814]
          tunnel: [w1808 w1813] -> w1803
          tunnel: [w1807 w1812] -> w1797
          tunnel: w1802 -> [w1809 w1811]
          tunnel: [w1809 w1811] -> w1800
          frame False {
          }
          frame True {
            n586 = call "Reset Totalizer to Zero (SubVI).vi"("Totalizer Number"="1", "Address"=w1811, "error in (no error)"=w1814, "VISA Refnum in"=w1815) -> ("error out"=w1812:errorcluster, "VISA Refnum out"=w1813:refnum<visa-resource-name>)  [unwired: 5 in, 1 out]
          }
        }
        n587 = Select(t=0, s=w1797, f=w1796) -> (s? t:f=w1798:i32)
      }
      event "Totalizer #2 Options.Reset Totalizer": Value Change {
        # "Reset if\ncomm error"
        # "Performs Totalizer#2 Reset to Zero Command"
        n588 = event-data() -> ("NewVal"=w1825:bool)  [unwired: 1 in, 1 out]
        n589 = Equal?(x=TRUE, y=w1825) -> (x = y?=w1838:bool)
        n590 = case shown="True" w1838 {
          tunnel: w1842 -> [w1845 w1852]
          tunnel: w1841 -> [w1844 w1851]
          tunnel: [w1845 w1850] -> w1840
          tunnel: [w1844 w1849] -> w1834
          tunnel: w1839 -> [w1846 w1848]
          tunnel: [w1846 w1848] -> w1837
          frame False {
          }
          frame True {
            n591 = call "Reset Totalizer to Zero (SubVI).vi"("Totalizer Number"="2", "Address"=w1848, "error in (no error)"=w1851, "VISA Refnum in"=w1852) -> ("error out"=w1849:errorcluster, "VISA Refnum out"=w1850:refnum<visa-resource-name>)  [unwired: 5 in, 1 out]
          }
        }
        n592 = Select(t=0, s=w1834, f=w1833) -> (s? t:f=w1835:i32)
      }
      event "Totalizer #1 Options.Enabled", "Totalizer #1 Options.Start @ Flow", "Totalizer #1 Options.Action Volume", "Totalizer #1 Options.Close Valve When Action Volume is Reached", "Totalizer #1 Options.Enable Auto Reset/Reload", "Totalizer #1 Options.Auto Reset Delay [seconds]", "Totalizer #1 Options.Power Up Delay [seconds]": Value Change {
        # "Reset if\ncomm error"
        # "Sends new Totalizer#1 selection to the instrument and updates device information claster."
        n593 = event-data() -> ("CtlRef"=w1864:refnum<vi>)  [unwired: 1 in, 2 out]
        n594 = property class="Ctl"(reference=w1864) -> ("Label.Text"=w1863:string)  [unwired: 1 in, 2 out]
        n595 = case shown="\"Enabled\"" w1863 {
          tunnel: w1880 -> [w1893 w1906 w1913 w1924 w1937 w1945 w1950 w1963]
          tunnel: w1879 -> [w1891 w1904 w1912 w1923 w1936 w1944 w1949 w1962]
          tunnel: [w1892 w1905 w1911 w1922 w1935 w1943 w1950 w1961] -> w1878
          tunnel: [w1890 w1903 w1910 w1921 w1934 w1942 w1949 w1960] -> w1873
          tunnel: w1877 -> [w1889 w1902 w1909 w1918 w1933 w1939 w1951 w1953]
          tunnel: [w1889 w1902 w1909 w1918 w1933 w1939 w1951 w1953] -> w1876
          tunnel: "Totalizer #1 Options" -> [w1888 w1901 w1917 w1928 w1938 w1948 _ w1958]
          frame "Start @ Flow" {
            n596 = Unbundle By Name(w1888) -> ("Start @ Flow"=w1887:dbl, "Action Volume"=w1884:dbl)
            n597 = Format Into String(format string="%f", w1887) -> (resulting string=w1882:string)  [unwired: 2 in, 1 out]
            n598 = Format Into String(format string="%f", w1884) -> (resulting string=w1881:string)  [unwired: 2 in, 1 out]
            n599 = call "Totalizer Start And Limit Command (SubVI).vi"("Start @ Flow"=w1882, "Totalizer Number"="1", "Address"=w1889, "error in (no error)"=w1891, "Limit Volume"=w1881, "VISA Refnum in"=w1893) -> ("error out"=w1890:errorcluster, "VISA Refnum out"=w1892:refnum<visa-resource-name>)  [unwired: 3 in, 1 out]
          }
          frame "Limit Volume" {
            n600 = Unbundle By Name(w1901) -> ("Start @ Flow"=w1900:dbl, "Action Volume"=w1897:dbl)
            n601 = Format Into String(format string="%f", w1900) -> (resulting string=w1895:string)  [unwired: 2 in, 1 out]
            n602 = Format Into String(format string="%f", w1897) -> (resulting string=w1894:string)  [unwired: 2 in, 1 out]
            n603 = call "Totalizer Start And Limit Command (SubVI).vi"("Start @ Flow"=w1895, "Totalizer Number"="1", "Address"=w1902, "error in (no error)"=w1904, "Limit Volume"=w1894, "VISA Refnum in"=w1906) -> ("error out"=w1903:errorcluster, "VISA Refnum out"=w1905:refnum<visa-resource-name>)  [unwired: 3 in, 1 out]
          }
          frame "Close Valve When Limit Volume is Reached" {
            n604 = Unbundle By Name(w1917) -> ("Close Valve When Action Volume is Reached"=w1914:bool)
            n605 = Select(t="V", s=w1914, f="D") -> (s? t:f=w1907:string)
            n606 = call "Totalizer Valve Action Command (SubVI).vi"("Valve Action In"=w1907, "Totalizer Number"="1", "Address"=w1909, "error in (no error)"=w1912, "VISA Refnum in"=w1913) -> ("error out"=w1910:errorcluster, "VISA Refnum out"=w1911:refnum<visa-resource-name>)  [unwired: 4 in, 1 out]
          }
          frame "Enable Auto Reset/Reload" {
            n607 = Unbundle By Name(w1928) -> ("Enable Auto Reset/Reload"=w1925:bool)
            n608 = Select(t="1", s=w1925, f="0") -> (s? t:f=w1919:string)
            n609 = call "Totalizer Auto Reset Command (SubVI).vi"("Auto Reset In"=w1919, "Totalizer Number"="1", "Address"=w1918, "error in (no error)"=w1923, "VISA Refnum in"=w1924) -> ("error out"=w1921:errorcluster, "VISA Refnum out"=w1922:refnum<visa-resource-name>)  [unwired: 4 in, 1 out]
          }
          frame "Auto Reset Delay [seconds]" {
            n610 = Unbundle By Name(w1938) -> ("Auto Reset Delay [seconds]"=w1930:dbl)
            n611 = Format Into String(format string="%d", w1930) -> (resulting string=w1929:string)  [unwired: 2 in, 1 out]
            n612 = call "Totalizer Auto Reset Delay (SubVI).vi"("Auto Reset Delay In"=w1929, "Totalizer Number"="1", "Address"=w1933, "error in (no error)"=w1936, "VISA Refnum in"=w1937) -> ("error out"=w1934:errorcluster, "VISA Refnum out"=w1935:refnum<visa-resource-name>)  [unwired: 4 in, 1 out]
          }
          frame "Power Up Delay [seconds] " {
            n613 = Unbundle By Name(w1948) -> ("Power Up Delay [seconds]"=w1946:dbl)
            n614 = Format Into String(format string="%d", w1946) -> (resulting string=w1940:string)  [unwired: 2 in, 1 out]
            n615 = call "Totalizer Power On Delay (SubVI).vi"("Power On Delay In"=w1940, "Totalizer Number"="1", "Address"=w1939, "error in (no error)"=w1944, "VISA Refnum in"=w1945) -> ("error out"=w1942:errorcluster, "VISA Refnum out"=w1943:refnum<visa-resource-name>)  [unwired: 4 in, 1 out]
          }
          frame "Else", Default {
          }
          frame "Enabled" {
            n616 = Unbundle By Name(w1958) -> ("Enabled"=w1957:bool)
            n617 = Select(t="E", s=w1957, f="D") -> (s? t:f=w1954:string)
            n618 = call "Totalizer Mode Command (SubVI).vi"("Mode"=w1954, "Totalizer Number"="1", "Address"=w1953, "error in (no error)"=w1962, "VISA Refnum in"=w1963) -> ("error out"=w1960:errorcluster, "Tot Reply String"=w1952:string, "VISA Refnum out"=w1961:refnum<visa-resource-name>)  [unwired: 4 in]
            n619 = property on="T1" class="Str"("Value"=w1952) -> ()  [unwired: 2 in, 2 out]
          }
        }
        n620 = Select(t=0, s=w1873, f=w1872) -> (s? t:f=w1874:i32)
      }
      event "Totalizer #2 Options.Start @ Flow", "Totalizer #2 Options.Close Valve When Action Volume is Reached", "Totalizer #2 Options.Enable Auto Reset/Reload", "Totalizer #2 Options.Auto Reset Delay [Seconds]", "Totalizer #2 Options.Power Up Delay [Seconds]", "Totalizer #2 Options.Action Volume", "Totalizer #2 Options.Enabled": Value Change {
        # "Reset if\ncomm error"
        # "Sends new Totalizer#2 selection to the instrument and updates device information claster."
        n621 = event-data() -> ("CtlRef"=w1975:refnum<vi>)  [unwired: 1 in, 2 out]
        n622 = property class="Ctl"(reference=w1975) -> ("Label.Text"=w1974:string)  [unwired: 1 in, 2 out]
        n623 = case shown="\"Enabled\"" w1974 {
          tunnel: w1991 -> [w2004 w2017 w2024 w2035 w2048 w2056 w2061 w2074]
          tunnel: w1990 -> [w2002 w2015 w2023 w2034 w2047 w2055 w2060 w2073]
          tunnel: [w2003 w2016 w2022 w2033 w2046 w2054 w2061 w2072] -> w1989
          tunnel: [w2001 w2014 w2021 w2032 w2045 w2053 w2060 w2071] -> w1984
          tunnel: w1988 -> [w2000 w2013 w2020 w2029 w2044 w2050 w2062 w2064]
          tunnel: [w2000 w2013 w2020 w2029 w2044 w2050 w2062 w2064] -> w1987
          tunnel: "Totalizer #2 Options" -> [w1999 w2012 w2028 w2039 w2049 w2059 _ w2069]
          frame "Start @ Flow" {
            n624 = Unbundle By Name(w1999) -> ("Start @ Flow"=w1998:dbl, "Action Volume"=w1995:dbl)
            n625 = Format Into String(format string="%f", w1998) -> (resulting string=w1993:string)  [unwired: 2 in, 1 out]
            n626 = Format Into String(format string="%f", w1995) -> (resulting string=w1992:string)  [unwired: 2 in, 1 out]
            n627 = call "Totalizer Start And Limit Command (SubVI).vi"("Start @ Flow"=w1993, "Totalizer Number"="2", "Address"=w2000, "error in (no error)"=w2002, "Limit Volume"=w1992, "VISA Refnum in"=w2004) -> ("error out"=w2001:errorcluster, "VISA Refnum out"=w2003:refnum<visa-resource-name>)  [unwired: 3 in, 1 out]
          }
          frame "Limit Volume" {
            n628 = Unbundle By Name(w2012) -> ("Start @ Flow"=w2011:dbl, "Action Volume"=w2008:dbl)
            n629 = Format Into String(format string="%f", w2011) -> (resulting string=w2006:string)  [unwired: 2 in, 1 out]
            n630 = Format Into String(format string="%f", w2008) -> (resulting string=w2005:string)  [unwired: 2 in, 1 out]
            n631 = call "Totalizer Start And Limit Command (SubVI).vi"("Start @ Flow"=w2006, "Totalizer Number"="2", "Address"=w2013, "error in (no error)"=w2015, "Limit Volume"=w2005, "VISA Refnum in"=w2017) -> ("error out"=w2014:errorcluster, "VISA Refnum out"=w2016:refnum<visa-resource-name>)  [unwired: 3 in, 1 out]
          }
          frame "Close Valve When Limit Volume is Reached" {
            n632 = Unbundle By Name(w2028) -> ("Close Valve When Action Volume is Reached"=w2025:bool)
            n633 = Select(t="V", s=w2025, f="D") -> (s? t:f=w2018:string)
            n634 = call "Totalizer Valve Action Command (SubVI).vi"("Valve Action In"=w2018, "Totalizer Number"="2", "Address"=w2020, "error in (no error)"=w2023, "VISA Refnum in"=w2024) -> ("error out"=w2021:errorcluster, "VISA Refnum out"=w2022:refnum<visa-resource-name>)  [unwired: 4 in, 1 out]
          }
          frame "Enable Auto Reset/Reload" {
            n635 = Unbundle By Name(w2039) -> ("Enable Auto Reset/Reload"=w2036:bool)
            n636 = Select(t="1", s=w2036, f="0") -> (s? t:f=w2030:string)
            n637 = call "Totalizer Auto Reset Command (SubVI).vi"("Auto Reset In"=w2030, "Totalizer Number"="2", "Address"=w2029, "error in (no error)"=w2034, "VISA Refnum in"=w2035) -> ("error out"=w2032:errorcluster, "VISA Refnum out"=w2033:refnum<visa-resource-name>)  [unwired: 4 in, 1 out]
          }
          frame "Auto Reset Delay [Seconds]" {
            n638 = Unbundle By Name(w2049) -> ("Auto Reset Delay [Seconds]"=w2041:dbl)
            n639 = Format Into String(format string="%d", w2041) -> (resulting string=w2040:string)  [unwired: 2 in, 1 out]
            n640 = call "Totalizer Auto Reset Delay (SubVI).vi"("Auto Reset Delay In"=w2040, "Totalizer Number"="2", "Address"=w2044, "error in (no error)"=w2047, "VISA Refnum in"=w2048) -> ("error out"=w2045:errorcluster, "VISA Refnum out"=w2046:refnum<visa-resource-name>)  [unwired: 4 in, 1 out]
          }
          frame "Power Up Delay [Seconds] " {
            n641 = Unbundle By Name(w2059) -> ("Power Up Delay [Seconds]"=w2057:dbl)
            n642 = Format Into String(format string="%d", w2057) -> (resulting string=w2051:string)  [unwired: 2 in, 1 out]
            n643 = call "Totalizer Power On Delay (SubVI).vi"("Power On Delay In"=w2051, "Totalizer Number"="2", "Address"=w2050, "error in (no error)"=w2055, "VISA Refnum in"=w2056) -> ("error out"=w2053:errorcluster, "VISA Refnum out"=w2054:refnum<visa-resource-name>)  [unwired: 4 in, 1 out]
          }
          frame "Else", Default {
          }
          frame "Enabled" {
            n644 = Unbundle By Name(w2069) -> ("Enabled"=w2068:bool)
            n645 = Select(t="E", s=w2068, f="D") -> (s? t:f=w2065:string)
            n646 = call "Totalizer Mode Command (SubVI).vi"("Mode"=w2065, "Totalizer Number"="2", "Address"=w2064, "error in (no error)"=w2073, "VISA Refnum in"=w2074) -> ("error out"=w2071:errorcluster, "Tot Reply String"=w2063:string, "VISA Refnum out"=w2072:refnum<visa-resource-name>)  [unwired: 4 in]
            n647 = property on="T2" class="Str"("Value"=w2063) -> ()  [unwired: 2 in, 2 out]
          }
        }
        n648 = Select(t=0, s=w1984, f=w1983) -> (s? t:f=w1985:i32)
      }
      event "Pulse Output Options.Enabled", "Pulse Output Options.Start @ Flow Rate", "Pulse Output Options.Unit Per Pulse", "Pulse Output Options.Pulse Active Time [ms]": Value Change {
        # "Reset if\ncomm error"
        # "Sends new Pulse Output selection to the instrument and updates device information claster."
        n649 = event-data() -> ("CtlRef"=w2086:refnum<vi>)  [unwired: 1 in, 2 out]
        n650 = property class="Ctl"(reference=w2086) -> ("Label.Text"=w2085:string)  [unwired: 1 in, 2 out]
        n651 = case shown="\"Enabled\"" w2085 {
          tunnel: w2102 -> [w2104 w2112 w2125 w2135 w2145]
          tunnel: w2101 -> [w2103 w2109 w2122 w2132 w2142]
          tunnel: [w2104 w2111 w2124 w2134 w2144] -> w2100
          tunnel: [w2103 w2110 w2123 w2133 w2143] -> w2095
          tunnel: w2099 -> [w2105 w2106 w2121 w2131 w2141]
          tunnel: [w2105 w2106 w2121 w2131 w2141] -> w2098
          tunnel: "Pulse Output Options" -> [_ w2116 w2126 w2136 w2146]
          frame "Else", Default {
          }
          frame "Enabled" {
            n652 = Unbundle By Name(w2116) -> ("Enabled"=w2115:bool)
            n653 = Select(t="E", s=w2115, f="D") -> (s? t:f=w2108:string)
            n654 = call "Process Pulse Output Command (SubVI).vi"("Argument#2"="", "Argument#1"=w2108, "Address"=w2106, "error in (no error)"=w2109, "VISA Refnum in"=w2112) -> ("error out"=w2110:errorcluster, "VISA Refnum out"=w2111:refnum<visa-resource-name>)  [unwired: 3 in, 2 out]
          }
          frame "Start @ Flow Rate" {
            n655 = Unbundle By Name(w2126) -> ("Start @ Flow Rate"=w2119:dbl)
            n656 = Format Into String(format string="%f", w2119) -> (resulting string=w2117:string)  [unwired: 2 in, 1 out]
            n657 = call "Process Pulse Output Command (SubVI).vi"("Argument#2"=w2117, "Argument#1"="F", "Address"=w2121, "error in (no error)"=w2122, "VISA Refnum in"=w2125) -> ("error out"=w2123:errorcluster, "VISA Refnum out"=w2124:refnum<visa-resource-name>)  [unwired: 3 in, 2 out]
          }
          frame "Unit Per Pulse" {
            n658 = Unbundle By Name(w2136) -> ("Unit Per Pulse"=w2129:dbl)
            n659 = Format Into String(format string="%f", w2129) -> (resulting string=w2127:string)  [unwired: 2 in, 1 out]
            n660 = call "Process Pulse Output Command (SubVI).vi"("Argument#2"=w2127, "Argument#1"="U", "Address"=w2131, "error in (no error)"=w2132, "VISA Refnum in"=w2135) -> ("error out"=w2133:errorcluster, "VISA Refnum out"=w2134:refnum<visa-resource-name>)  [unwired: 3 in, 2 out]
          }
          frame "Pulse Active Time [ms]" {
            n661 = Unbundle By Name(w2146) -> ("Pulse Active Time [ms]"=w2138:dbl)
            n662 = Format Into String(format string="%d", w2138) -> (resulting string=w2137:string)  [unwired: 2 in, 1 out]
            n663 = call "Process Pulse Output Command (SubVI).vi"("Argument#2"=w2137, "Argument#1"="T", "Address"=w2141, "error in (no error)"=w2142, "VISA Refnum in"=w2145) -> ("error out"=w2143:errorcluster, "VISA Refnum out"=w2144:refnum<visa-resource-name>)  [unwired: 3 in, 2 out]
          }
        }
        n664 = Select(t=0, s=w2095, f=w2094) -> (s? t:f=w2096:i32)
      }
      event "Flow Alarm.Enabled", "Flow Alarm.High Alarm Limit", "Flow Alarm.Low Alarm Limit", "Flow Alarm.Flow Alarm Latch", "Flow Alarm.Action Delay [s]", "Flow Alarm.Power Up Delay [s]", "Flow Alarm.Flow Alarm Valve Action:": Value Change {
        # "Reset if\ncomm error"
        # "Sends new Flow Alarm selection to the instrument and updates device information claster."
        n665 = event-data() -> ("CtlRef"=w2160:refnum<vi>)  [unwired: 1 in, 2 out]
        n666 = property class="Ctl"(reference=w2160) -> ("Label.Text"=w2159:string)  [unwired: 1 in, 2 out]
        n667 = case shown="\"Enabled\"" w2159 {
          tunnel: w2175 -> [w2178 w2188 w2203 w2218 w2235 w2244 w2264 w2276]
          tunnel: w2174 -> [w2177 w2187 w2202 w2217 w2234 w2241 w2263 w2275]
          tunnel: [w2178 w2186 w2201 w2216 w2233 w2243 w2262 w2274] -> w2173
          tunnel: [w2177 w2185 w2200 w2215 w2232 w2242 w2261 w2273] -> w2168
          tunnel: w2172 -> [w2179 w2183 w2199 w2214 w2231 w2240 w2260 w2272]
          tunnel: [w2179 w2183 w2199 w2214 w2231 w2240 w2260 w2272] -> w2171
          tunnel: "Flow Alarm" -> [_ w2193 w2208 w2223 w2236 w2245 w2265 w2277]
          tunnel: w2156 -> [_ _ _ _ _ w2238 _ _]
          tunnel: w2155 -> [w2176 w2181 w2195 w2210 w2225 w2237 w2255 w2267]
          tunnel: [w2176 w2180 w2194 w2209 w2224 w2237 w2254 w2266] -> w2154
          frame "Else", Default {
          }
          frame "Enabled" {
            n668 = Unbundle By Name(w2193) -> ("Enabled"=w2192:bool)
            n669 = Select(t="E", s=w2192, f="D") -> (s? t:f=w2184:string)
            n670 = call "Process Flow Alarm Command (SubVI).vi"("Argument#2"="", "Argument#1"=w2184, "Address"=w2183, "error in (no error)"=w2187, "Argument#3"="", "Alarm Configuration In"=w2181, "VISA Refnum in"=w2188) -> ("error out"=w2185:errorcluster, "Alarm Configuration Out"=w2180:T18, "VISA Refnum out"=w2186:refnum<visa-resource-name>)  [unwired: 1 in, 1 out]
          }
          frame "High Alarm Limit" {
            n671 = Unbundle By Name(w2208) -> ("High Alarm Limit"=w2206:dbl, "Low Alarm Limit"=w2204:dbl)
            n672 = Format Into String(format string="%f", w2206) -> (resulting string=w2198:string)  [unwired: 2 in, 1 out]
            n673 = Format Into String(format string="%f", w2204) -> (resulting string=w2196:string)  [unwired: 2 in, 1 out]
            n674 = call "Process Flow Alarm Command (SubVI).vi"("Argument#2"=w2198, "Argument#1"="C", "Address"=w2199, "error in (no error)"=w2202, "Argument#3"=w2196, "Alarm Configuration In"=w2195, "VISA Refnum in"=w2203) -> ("error out"=w2200:errorcluster, "Alarm Configuration Out"=w2194:T18, "VISA Refnum out"=w2201:refnum<visa-resource-name>)  [unwired: 1 in, 1 out]
          }
          frame "Low Alarm Limit" {
            n675 = Unbundle By Name(w2223) -> ("High Alarm Limit"=w2221:dbl, "Low Alarm Limit"=w2219:dbl)
            n676 = Format Into String(format string="%f", w2221) -> (resulting string=w2213:string)  [unwired: 2 in, 1 out]
            n677 = Format Into String(format string="%f", w2219) -> (resulting string=w2211:string)  [unwired: 2 in, 1 out]
            n678 = call "Process Flow Alarm Command (SubVI).vi"("Argument#2"=w2213, "Argument#1"="C", "Address"=w2214, "error in (no error)"=w2217, "Argument#3"=w2211, "Alarm Configuration In"=w2210, "VISA Refnum in"=w2218) -> ("error out"=w2215:errorcluster, "Alarm Configuration Out"=w2209:T18, "VISA Refnum out"=w2216:refnum<visa-resource-name>)  [unwired: 1 in, 1 out]
          }
          frame "Flow Alarm Latch" {
            n679 = Unbundle By Name(w2236) -> ("Flow Alarm Latch"=w2227:bool)
            n680 = Select(t="1", s=w2227, f="0") -> (s? t:f=w2226:string)
            n681 = call "Process Flow Alarm Command (SubVI).vi"("Argument#2"=w2226, "Argument#1"="L", "Address"=w2231, "error in (no error)"=w2234, "Alarm Configuration In"=w2225, "VISA Refnum in"=w2235) -> ("error out"=w2232:errorcluster, "Alarm Configuration Out"=w2224:T18, "VISA Refnum out"=w2233:refnum<visa-resource-name>)  [unwired: 2 in, 1 out]
          }
          frame "Flow Alarm Valve Action:" {
            n682 = Unbundle By Name(w2245) -> ("Flow Alarm Valve Action:"=w2239:string)
            n683 = case shown="True" w2238 {
              tunnel: w2244 -> [w2247 w2253]
              tunnel: [w2247 w2252] -> w2243
              tunnel: [w2246 w2251] -> w2242
              tunnel: w2241 -> [w2246 w2250]
              tunnel: w2240 -> [_ w2249]
              tunnel: w2239 -> [_ w2248]
              frame False {
              }
              frame True {
                n684 = call "Read Alarm Valve Action (SubVI).vi"("Valve Action In"=w2248, "Address"=w2249, "error in (no error)"=w2250, "VISA Refnum in"=w2253) -> ("error out"=w2251:errorcluster, "VISA Refnum out"=w2252:refnum<visa-resource-name>)  [unwired: 5 in, 1 out]
              }
            }
          }
          frame "Action Delay [s]" {
            n685 = Unbundle By Name(w2265) -> ("Action Delay [s]"=w2257:dbl)
            n686 = Format Into String(format string="%d", w2257) -> (resulting string=w2256:string)  [unwired: 2 in, 1 out]
            n687 = call "Process Flow Alarm Command (SubVI).vi"("Argument#2"=w2256, "Argument#1"="A", "Address"=w2260, "error in (no error)"=w2263, "Alarm Configuration In"=w2255, "VISA Refnum in"=w2264) -> ("error out"=w2261:errorcluster, "Alarm Configuration Out"=w2254:T18, "VISA Refnum out"=w2262:refnum<visa-resource-name>)  [unwired: 2 in, 1 out]
          }
          frame "Power Up Delay [s]" {
            n688 = Unbundle By Name(w2277) -> ("Power Up Delay [s]"=w2269:dbl)
            n689 = Format Into String(format string="%d", w2269) -> (resulting string=w2268:string)  [unwired: 2 in, 1 out]
            n690 = call "Process Flow Alarm Command (SubVI).vi"("Argument#2"=w2268, "Argument#1"="P", "Address"=w2272, "error in (no error)"=w2275, "Alarm Configuration In"=w2267, "VISA Refnum in"=w2276) -> ("error out"=w2273:errorcluster, "Alarm Configuration Out"=w2266:T18, "VISA Refnum out"=w2274:refnum<visa-resource-name>)  [unwired: 2 in, 1 out]
          }
        }
        n691 = Select(t=0, s=w2168, f=w2167) -> (s? t:f=w2169:i32)
      }
      event "Temperature Alarm.Enabled", "Temperature Alarm.High Temp. Alarm Limit", "Temperature Alarm.Low Temp. Alarm Limit", "Temperature Alarm.Temp. Alarm Latch", "Temperature Alarm.Action Delay [s]", "Temperature Alarm.Power Up Delay [s]": Value Change {
        # "Reset if\ncomm error"
        # "Sends new Flow Alarm selection to the instrument and updates device information claster."
        n692 = event-data() -> ("CtlRef"=w2291:refnum<vi>)  [unwired: 1 in, 2 out]
        n693 = property class="Ctl"(reference=w2291) -> ("Label.Text"=w2290:string)  [unwired: 1 in, 2 out]
        n694 = case shown="\"Enabled\"" w2290 {
          tunnel: w2306 -> [w2309 w2317 w2334 w2348 w2362 w2375 w2387]
          tunnel: w2305 -> [w2308 w2318 w2331 w2347 w2360 w2374 w2386]
          tunnel: [w2309 w2320 w2333 w2349 w2363 w2376 w2388] -> w2304
          tunnel: [w2308 w2319 w2332 w2346 w2361 w2373 w2385] -> w2299
          tunnel: w2303 -> [w2310 w2311 w2329 w2340 w2357 w2370 w2382]
          tunnel: [w2310 w2311 w2329 w2340 w2357 w2370 w2382] -> w2302
          tunnel: "Temperature Alarm" -> [_ w2324 w2339 w2354 w2367 w2379 w2391]
          tunnel: w2288 -> [_ _ _ _ _ _ _]
          tunnel: w2285 -> [w2307 w2316 w2330 w2344 w2359 w2372 w2384]
          tunnel: [w2307 w2315 w2328 w2345 w2358 w2371 w2383] -> w2284
          frame "Else", Default {
          }
          frame "Enabled" {
            n695 = Unbundle By Name(w2324) -> ("Enabled"=w2323:bool)
            n696 = Select(t="E", s=w2323, f="D") -> (s? t:f=w2314:string)
            n697 = call "Process Temp Alarm Command (SubVI).vi"("Argument#2"="", "Argument#1"=w2314, "Address"=w2311, "error in (no error)"=w2318, "Argument#3"="", "Alarm Configuration In"=w2316, "VISA Refnum in"=w2317) -> ("error out"=w2319:errorcluster, "Alarm Configuration Out"=w2315:T18, "VISA Refnum out"=w2320:refnum<visa-resource-name>)  [unwired: 1 in, 1 out]
          }
          frame "High Temp. Alarm Limit" {
            n698 = Unbundle By Name(w2339) -> ("High Temp. Alarm Limit"=w2337:dbl, "Low Temp. Alarm Limit"=w2335:dbl)
            n699 = Format Into String(format string="%f", w2337) -> (resulting string=w2326:string)  [unwired: 2 in, 1 out]
            n700 = Format Into String(format string="%f", w2335) -> (resulting string=w2327:string)  [unwired: 2 in, 1 out]
            n701 = call "Process Temp Alarm Command (SubVI).vi"("Argument#2"=w2326, "Argument#1"="C", "Address"=w2329, "error in (no error)"=w2331, "Argument#3"=w2327, "Alarm Configuration In"=w2330, "VISA Refnum in"=w2334) -> ("error out"=w2332:errorcluster, "Alarm Configuration Out"=w2328:T18, "VISA Refnum out"=w2333:refnum<visa-resource-name>)  [unwired: 1 in, 1 out]
          }
          frame "Low Temp. Alarm Limit" {
            n702 = Unbundle By Name(w2354) -> ("High Temp. Alarm Limit"=w2352:dbl, "Low Temp. Alarm Limit"=w2350:dbl)
            n703 = Format Into String(format string="%f", w2352) -> (resulting string=w2341:string)  [unwired: 2 in, 1 out]
            n704 = Format Into String(format string="%f", w2350) -> (resulting string=w2342:string)  [unwired: 2 in, 1 out]
            n705 = call "Process Temp Alarm Command (SubVI).vi"("Argument#2"=w2341, "Argument#1"="C", "Address"=w2340, "error in (no error)"=w2347, "Argument#3"=w2342, "Alarm Configuration In"=w2344, "VISA Refnum in"=w2348) -> ("error out"=w2346:errorcluster, "Alarm Configuration Out"=w2345:T18, "VISA Refnum out"=w2349:refnum<visa-resource-name>)  [unwired: 1 in, 1 out]
          }
          frame "Temp. Alarm Latch" {
            n706 = Unbundle By Name(w2367) -> ("Temp. Alarm Latch"=w2364:bool)
            n707 = Select(t="1", s=w2364, f="0") -> (s? t:f=w2356:string)
            n708 = call "Process Temp Alarm Command (SubVI).vi"("Argument#2"=w2356, "Argument#1"="L", "Address"=w2357, "error in (no error)"=w2360, "Alarm Configuration In"=w2359, "VISA Refnum in"=w2362) -> ("error out"=w2361:errorcluster, "Alarm Configuration Out"=w2358:T18, "VISA Refnum out"=w2363:refnum<visa-resource-name>)  [unwired: 2 in, 1 out]
          }
          frame "Action Delay [s]" {
            n709 = Unbundle By Name(w2379) -> ("Action Delay [s]"=w2377:dbl)
            n710 = Format Into String(format string="%d", w2377) -> (resulting string=w2368:string)  [unwired: 2 in, 1 out]
            n711 = call "Process Temp Alarm Command (SubVI).vi"("Argument#2"=w2368, "Argument#1"="A", "Address"=w2370, "error in (no error)"=w2374, "Alarm Configuration In"=w2372, "VISA Refnum in"=w2375) -> ("error out"=w2373:errorcluster, "Alarm Configuration Out"=w2371:T18, "VISA Refnum out"=w2376:refnum<visa-resource-name>)  [unwired: 2 in, 1 out]
          }
          frame "Power Up Delay [s]" {
            n712 = Unbundle By Name(w2391) -> ("Power Up Delay [s]"=w2389:dbl)
            n713 = Format Into String(format string="%d", w2389) -> (resulting string=w2381:string)  [unwired: 2 in, 1 out]
            n714 = call "Process Temp Alarm Command (SubVI).vi"("Argument#2"=w2381, "Argument#1"="P", "Address"=w2382, "error in (no error)"=w2386, "Alarm Configuration In"=w2384, "VISA Refnum in"=w2387) -> ("error out"=w2385:errorcluster, "Alarm Configuration Out"=w2383:T18, "VISA Refnum out"=w2388:refnum<visa-resource-name>)  [unwired: 2 in, 1 out]
          }
        }
        n715 = Select(t=0, s=w2299, f=w2298) -> (s? t:f=w2300:i32)
      }
      event "Pressure Alarm.Enabled", "Pressure Alarm.High Pressure Alarm Limit", "Pressure Alarm.Low Pressure Alarm Limit", "Pressure Alarm.Pressure Alarm Latch", "Pressure Alarm.Action Delay [s]", "Pressure Alarm.Power Up Delay [s]": Value Change {
        # "Reset if\ncomm error"
        # "Sends new Flow Alarm selection to the instrument and updates device information claster."
        n716 = event-data() -> ("CtlRef"=w2404:refnum<vi>)  [unwired: 1 in, 2 out]
        n717 = property class="Ctl"(reference=w2404) -> ("Label.Text"=w2403:string)  [unwired: 1 in, 2 out]
        n718 = case shown="\"Enabled\"" w2403 {
          tunnel: w2419 -> [w2422 w2430 w2446 w2461 w2474 w2487 w2500]
          tunnel: w2418 -> [w2421 w2431 w2445 w2458 w2473 w2486 w2499]
          tunnel: [w2422 w2433 w2447 w2462 w2475 w2488 w2501] -> w2417
          tunnel: [w2421 w2432 w2444 w2459 w2470 w2485 w2498] -> w2412
          tunnel: w2416 -> [w2423 w2427 w2441 w2453 w2469 w2481 w2493]
          tunnel: [w2423 w2427 w2441 w2453 w2469 w2481 w2493] -> w2415
          tunnel: "Pressure Alarm" -> [_ w2437 w2452 w2467 w2480 w2492 w2504]
          tunnel: w2401 -> [_ _ _ _ _ _ _]
          tunnel: w2399 -> [w2420 w2429 w2442 w2460 w2472 w2483 w2495]
          tunnel: [w2420 w2428 w2443 w2454 w2471 w2484 w2494] -> w2398
          frame "Else", Default {
          }
          frame "Enabled" {
            n719 = Unbundle By Name(w2437) -> ("Enabled"=w2436:bool)
            n720 = Select(t="E", s=w2436, f="D") -> (s? t:f=w2426:string)
            n721 = call "Process Pressure Alarm Command (SubVI).vi"("Argument#2"="", "Argument#1"=w2426, "Address"=w2427, "error in (no error)"=w2431, "Argument#3"="", "Alarm Configuration In"=w2429, "VISA Refnum in"=w2430) -> ("error out"=w2432:errorcluster, "Alarm Configuration Out"=w2428:T18, "VISA Refnum out"=w2433:refnum<visa-resource-name>)  [unwired: 1 in, 1 out]
          }
          frame "High Pressure Alarm Limit" {
            n722 = Unbundle By Name(w2452) -> ("High Pressure Alarm Limit"=w2450:dbl, "Low Pressure Alarm Limit"=w2448:dbl)
            n723 = Format Into String(format string="%f", w2450) -> (resulting string=w2439:string)  [unwired: 2 in, 1 out]
            n724 = Format Into String(format string="%f", w2448) -> (resulting string=w2440:string)  [unwired: 2 in, 1 out]
            n725 = call "Process Pressure Alarm Command (SubVI).vi"("Argument#2"=w2439, "Argument#1"="C", "Address"=w2441, "error in (no error)"=w2445, "Argument#3"=w2440, "Alarm Configuration In"=w2442, "VISA Refnum in"=w2446) -> ("error out"=w2444:errorcluster, "Alarm Configuration Out"=w2443:T18, "VISA Refnum out"=w2447:refnum<visa-resource-name>)  [unwired: 1 in, 1 out]
          }
          frame "Low Pressure Alarm Limit" {
            n726 = Unbundle By Name(w2467) -> ("High Pressure Alarm Limit"=w2465:dbl, "Low Pressure Alarm Limit"=w2463:dbl)
            n727 = Format Into String(format string="%f", w2465) -> (resulting string=w2456:string)  [unwired: 2 in, 1 out]
            n728 = Format Into String(format string="%f", w2463) -> (resulting string=w2457:string)  [unwired: 2 in, 1 out]
            n729 = call "Process Pressure Alarm Command (SubVI).vi"("Argument#2"=w2456, "Argument#1"="C", "Address"=w2453, "error in (no error)"=w2458, "Argument#3"=w2457, "Alarm Configuration In"=w2460, "VISA Refnum in"=w2461) -> ("error out"=w2459:errorcluster, "Alarm Configuration Out"=w2454:T18, "VISA Refnum out"=w2462:refnum<visa-resource-name>)  [unwired: 1 in, 1 out]
          }
          frame "Pressure Alarm Latch" {
            n730 = Unbundle By Name(w2480) -> ("Pressure Alarm Latch"=w2477:bool)
            n731 = Select(t="1", s=w2477, f="0") -> (s? t:f=w2468:string)
            n732 = call "Process Pressure Alarm Command (SubVI).vi"("Argument#2"=w2468, "Argument#1"="L", "Address"=w2469, "error in (no error)"=w2473, "Alarm Configuration In"=w2472, "VISA Refnum in"=w2474) -> ("error out"=w2470:errorcluster, "Alarm Configuration Out"=w2471:T18, "VISA Refnum out"=w2475:refnum<visa-resource-name>)  [unwired: 2 in, 1 out]
          }
          frame "Action Delay [s]" {
            n733 = Unbundle By Name(w2492) -> ("Action Delay [s]"=w2490:dbl)
            n734 = Format Into String(format string="%d", w2490) -> (resulting string=w2482:string)  [unwired: 2 in, 1 out]
            n735 = call "Process Pressure Alarm Command (SubVI).vi"("Argument#2"=w2482, "Argument#1"="A", "Address"=w2481, "error in (no error)"=w2486, "Alarm Configuration In"=w2483, "VISA Refnum in"=w2487) -> ("error out"=w2485:errorcluster, "Alarm Configuration Out"=w2484:T18, "VISA Refnum out"=w2488:refnum<visa-resource-name>)  [unwired: 2 in, 1 out]
          }
          frame "Power Up Delay [s]" {
            n736 = Unbundle By Name(w2504) -> ("Power Up Delay [s]"=w2502:dbl)
            n737 = Format Into String(format string="%d", w2502) -> (resulting string=w2496:string)  [unwired: 2 in, 1 out]
            n738 = call "Process Pressure Alarm Command (SubVI).vi"("Argument#2"=w2496, "Argument#1"="P", "Address"=w2493, "error in (no error)"=w2499, "Alarm Configuration In"=w2495, "VISA Refnum in"=w2500) -> ("error out"=w2498:errorcluster, "Alarm Configuration Out"=w2494:T18, "VISA Refnum out"=w2501:refnum<visa-resource-name>)  [unwired: 2 in, 1 out]
          }
        }
        n739 = Select(t=0, s=w2412, f=w2411) -> (s? t:f=w2413:i32)
      }
      event "AE Reset": Value Change {
        # "Reset if\ncomm error"
        # "Resets Alarm Events LED Indicators when corresponding Alarm Event Latch is enabled."
        n740 = event-data() -> ("NewVal"=w2514:bool)  [unwired: 1 in]
        n741 = Equal?(x=TRUE, y=w2514) -> (x = y?=w2515:bool)
        n742 = case shown="True" w2515 {
          tunnel: w2512 -> [w2534 w2541]
          tunnel: w2511 -> [w2533 w2538]
          tunnel: [w2534 w2540] -> w2513
          tunnel: [w2533 w2539] -> w2510
          tunnel: w2508 -> [w2535 w2536]
          tunnel: [w2535 w2536] -> w2509
          frame False {
          }
          frame True {
            n743 = call "Process Alarm Events Command (SubVI).vi"("Argument#2"="", "Argument#1"="R", "Address"=w2536, "error in (no error)"=w2538, "VISA Refnum in"=w2541) -> ("error out"=w2539:errorcluster, "VISA Refnum out"=w2540:refnum<visa-resource-name>)  [unwired: 4 in, 1 out]
          }
        }
        n744 = Select(t=0, s=w2510, f=w2530) -> (s? t:f=w2531:i32)
      }
      event "Alarm Events.AE Enable 0", "Alarm Events.AE Enable 1", "Alarm Events.AE Enable 2", "Alarm Events.AE Enable 3", "Alarm Events.AE Enable 4", "Alarm Events.AE Enable 5", "Alarm Events.AE Enable 6", "Alarm Events.AE Enable 7", "Alarm Events.AE Enable 8", "Alarm Events.AE Enable 9", "Alarm Events.AE Enable 10", "Alarm Events.AE Enable 11", "Alarm Events.AE Enable 12", "Alarm Events.AE Enable 13", "Alarm Events.AE Latch 0", "Alarm Events.AE Latch 1", "Alarm Events.AE Latch 2", "Alarm Events.AE Latch 3", "Alarm Events.AE Latch 4", "Alarm Events.AE Latch 5", "Alarm Events.AE Latch 6", "Alarm Events.AE Latch 7", "Alarm Events.AE Latch 8", "Alarm Events.AE Latch 9", "Alarm Events.AE Latch 10", "Alarm Events.AE Latch 11", "Alarm Events.AE Latch 12", "Alarm Events.AE Latch 13": Value Change {
        # "Reset if\ncomm error"
        # "Converts Alarm Events Mask and Latch settings to hexadecimal strings and sends them to the instruments."
        n745 = event-data() -> ()  [unwired: 1 in, 6 out]
        n746 = call "Convert Alarm Events to Number (SubVI).vi"("Alarm Events In"="Alarm Events") -> ("Latch Hex String"=w2548:string, "Enable Hex String"=w2549:string)  [unwired: 9 in]
        n747 = call "Process Alarm Events Command (SubVI).vi"("Argument#2"=w2549, "Argument#1"="M", "Address"=w2552, "error in (no error)"=w2553, "VISA Refnum in"=w2556) -> ("error out"=w2555:errorcluster, "VISA Refnum out"=w2558:refnum<visa-resource-name>)  [unwired: 4 in, 1 out]
        n748 = call "Process Alarm Events Command (SubVI).vi"("Argument#2"=w2548, "Argument#1"="L", "Address"=w2552, "error in (no error)"=w2555, "VISA Refnum in"=w2558) -> ("error out"=w2554:errorcluster, "VISA Refnum out"=w2557:refnum<visa-resource-name>)  [unwired: 4 in, 1 out]
        n749 = Select(t=0, s=w2554, f=w2570) -> (s? t:f=w2571:i32)
      }
      event "Log Register Values": Value Change {
        # "Reset if\ncomm error"
        # "Reads all current EEPROM registers values in to the text file in the folder containing this VI."
        n750 = event-data() -> ()  [unwired: 1 in, 2 out]
        n751 = Unbundle By Name(w2580) -> ("Serial Number"=w2579:string)
        n752 = case shown="True" "Log Register Values" {
          tunnel: w2584 -> [w2600 w2607]
          tunnel: w2583 -> [w2599 w2606]
          tunnel: [w2600 w2605] -> w2582
          tunnel: w2578 -> [_ w2604]
          tunnel: [w2599 w2602] -> w2581
          tunnel: w2579 -> [_ w2601]
          frame False {
          }
          frame True {
            n753 = Get Date/Time String(want seconds? (F)=TRUE) -> (date string=w2613:string, time string=w2612:string)  [unwired: 2 in]
            n754 = Concatenate Strings(w2613, ", " ("string"), w2612) -> (w2608:string)
            n755 = call "Log Registers Values (SubVI).vi"("Address"=w2604, "error in (no error)"=w2606, "Serial Number"=w2601, "VISA Refnum in"=w2607) -> ("error out"=w2603:errorcluster, "VISA Refnum out"=w2605:refnum<visa-resource-name>)  [unwired: 6 in]
            n756 = Concatenate Strings("Register log saved in VI folder." ("Message"), w2608) -> (w2610:string)
            n757 = call "Display Message to User"("error in (no error)"=w2603, "Message"=w2610) -> ("error out"=w2602:errorcluster)  [unwired: 8 in, 1 out]
          }
        }
        n758 = Select(t=0, s=w2581, f=w2596) -> (s? t:f=w2597:i32)
      }
      event "Read Register", "Reg. to read": Value Change {
        # "Reset if\ncomm error"
        # "Reads selected EEPROM registers number value when Read Register button is pressed or register number is changed."
        n759 = event-data() -> ()  [unwired: 1 in, 6 out]
        n760 = Number To Decimal String(number="Reg. to read") -> (decimal integer string=w2619:string)  [unwired: 1 in]
        n761 = call "Read Register (SubVI).vi"("Address"=w2621, "error in (no error)"=w2625, "Register Number"=w2619, "VISA Refnum in"=w2626) -> ("error out"=w2623:errorcluster, "Register Value"=→"Register Value":string, "VISA Refnum out"=w2624:refnum<visa-resource-name>)  [unwired: 5 in]
        n762 = Select(t=0, s=w2623, f=w2638) -> (s? t:f=w2639:i32)
      }
      event "Gas mixture input.Create Mixture": Value Change {
        w2651 = ""
        # "Reset if\ncomm error"
        # "Checks Gas Mixture ratios and sends command to create new gas mixture."
        n763 = event-data() -> ()  [unwired: 1 in, 3 out]
        n764 = call "Process Compose Mixture Command (SubVI).vi"("Argument#4"=w2651, "Argument#2"=w2651, "Argument#1"=w2651, "Address"=w2641, "error in (no error)"=w2654, "Argument#3"=w2651, "VISA Refnum in"=w2655) -> ("error out"=w2652:errorcluster, "CM Output String"=w2650:string, "VISA Refnum out"=w2653:refnum<visa-resource-name>)  [unwired: 2 in]
        n765 = Decimal String To Number(string=w2650) -> (number=w2656:i32)  [unwired: 2 in, 1 out]
        n766 = To Long Integer(number=w2656) -> (32bit integer=w2649:i32)
        n767 = global write "Global.vi" "GM Number"(w2656) -> ()
        n768 = Less?(x=w2649, y=20) -> (x < y?=w2647:bool)
        n769 = case shown="True" w2647 {
          tunnel: [w2692 w2700] -> w2644
          tunnel: [w2691 w2698] -> w2645
          tunnel: w2653 -> [w2692 w2699]
          tunnel: w2652 -> [w2691 w2697]
          tunnel: w2641 -> [_ w2701]
          tunnel: "Gas mixture input" -> [_ w2704]
          frame False {
          }
          frame True {
            n770 = Unbundle(w2704) -> ("Ratio % 1"=w2705:dbl, "Enable # 1"=w2706:bool, "Ratio % 2"=w2707:dbl, "Enable # 2"=w2708:bool, "Ratio % 3"=w2709:dbl, "Enable # 3"=w2710:bool, "Ratio % 4"=w2712:dbl, "Enable # 4"=w2711:bool, "Ratio % 5"=w2713:dbl, "Enable # 5"=w2714:bool, "Mixture Gas 1"=w2702:u16, "Mixture Gas 2"=w2718:u16, "Mixture Gas 3"=w2717:u16, "Mixture Gas 4"=w2716:u16, "Mixture Gas 5"=w2715:u16, "Mix. #"=w2694:u16, "Mix. name"=w2696:string)  [unwired: 3 out]
            n771 = Bundle(cluster=T24 {"Gas # 1"=236, "Mix % 1"=0.0, "Include # 1"=FALSE, "Gas # 2"=0, "Mix % 2"=0.0, "Include # 2"=FALSE, "Gas # 3"=0, "Mix % 3"=0.0, "Include # 3"=FALSE, "Gas # 4"=0, "Mix % 4"=0.0, "Include # 4"=FALSE, "Gas # 5"=0, "Mix % 5"=0.0, "Include # 5"=FALSE} ("COMPOSER gas mix input"), "Gas # 1"=w2702, "Mix % 1"=w2705, "Include # 1"=w2706, "Gas # 2"=w2718, "Mix % 2"=w2707, "Include # 2"=w2708, "Gas # 3"=w2717, "Mix % 3"=w2709, "Include # 3"=w2710, "Gas # 4"=w2716, "Mix % 4"=w2712, "Include # 4"=w2711, "Gas # 5"=w2715, "Mix % 5"=w2713, "Include # 5"=w2714) -> (w2695:T24)
            n772 = call "Write Gas Mixture.vi"("Gas mix name"=w2696, "Address"=w2701, "error in"=w2697, "Gas # to store mix as"=w2694, "User Defined gas mixture input"=w2695, "VISA Refnum in"=w2699) -> ("error out"=w2698:errorcluster, "Completion text"=w2693:string, "VISA Refnum out"=w2700:refnum<visa-resource-name>)  [unwired: 3 in]
            n773 = property on="Completion\ntext" class="Str"("Value"=w2693) -> ()  [unwired: 2 in, 2 out]
          }
        }
        n774 = case shown="No Error" w2645 {
          selector: w2645 -> [w2681 w2689]
          tunnel: w2644 -> [w2684 w2690]
          tunnel: [w2687 w2690] -> w2643
          tunnel: [w2686 w2689] -> w2642
          tunnel: w2641 -> [w2677 _]
          frame No Error {
            w2685 = ""
            n775 = call "Process Compose Mixture Command (SubVI).vi"("Argument#4"=w2685, "Argument#2"=w2685, "Argument#1"=w2685, "Address"=w2677, "error in (no error)"=w2681, "Argument#3"=w2685, "VISA Refnum in"=w2684) -> ("error out"=w2682:errorcluster, "CM Output String"=w2679:string, "VISA Refnum out"=w2683:refnum<visa-resource-name>)  [unwired: 2 in]
            n776 = Decimal String To Number(string=w2679) -> (number=w2680:i32)  [unwired: 2 in, 1 out]
            n777 = call "Init Gas Combo (SubVI).vi"("name or relative path"="GasTable.txt") -> ("Array"=w2675:cluster{"String":string, "Value":string}[])  [unwired: 10 in]
            n778 = To Unsigned Word Integer(number=w2680) -> (unsigned 16bit integer=w2678:u16)
            n779 = call "Update Gas Combo with GM (SubVI).vi"("VISA Refnum in"=w2683, "Array In"=w2675, "Number of Mixtures"=w2678, "error in (no error)"=w2682, "Address String"=w2677) -> ("VISA Refnum out"=w2687:refnum<visa-resource-name>, "Array Out"=w2688:cluster{"String":string, "Value":string}[], "error out"=w2686:errorcluster)  [unwired: 3 in]
            n780 = global write "Global.vi" "GM Number"(w2678) -> ()
            n781 = property on="Selected Gas" class="CmbBox"("Strings And Values[]"=w2688) -> ()  [unwired: 2 in, 2 out]
          }
          frame Error {
          }
        }
        n782 = Select(t=0, s=w2642, f=w2672) -> (s? t:f=w2673:i32)
      }
      event "Gas mixture input.Delete Mixture": Value Change {
        w2730 = ""
        # "Get number of mixtures in the instrument EEPROM memory."
        # "Reset if\ncomm error"
        # "Checks Number of Gas Mixtures saved in the instrument memory and delete the last entry if it is present. Updates Select Gas combo box."
        n783 = event-data() -> ("NewVal"=w2721:bool)  [unwired: 1 in, 1 out]
        n784 = call "Process Compose Mixture Command (SubVI).vi"("Argument#4"=w2730, "Argument#2"=w2730, "Argument#1"=w2730, "Address"=w2726, "error in (no error)"=w2731, "Argument#3"=w2730, "VISA Refnum in"=w2732) -> ("error out"=w2719:errorcluster, "CM Output String"=w2729:string, "VISA Refnum out"=w2720:refnum<visa-resource-name>)  [unwired: 2 in]
        n785 = Decimal String To Number(string=w2729) -> (number=w2733:i32)  [unwired: 2 in, 1 out]
        n786 = global write "Global.vi" "GM Number"(w2733) -> ()
        n787 = To Long Integer(number=w2733) -> (32bit integer=w2725:i32)
        n788 = Greater Than 0?(x=w2725) -> (x > 0?=w2722:bool)
        n789 = case shown="True" w2721 {
          tunnel: [w2751 w2757] -> w2728
          tunnel: [w2750 w2756] -> w2727
          tunnel: w2726 -> [_ w2755]
          tunnel: w2722 -> [_ w2754]
          tunnel: w2720 -> [w2751 w2753]
          tunnel: w2719 -> [w2750 w2752]
          frame False {
          }
          frame True {
            n790 = case shown="True" w2754 {
              tunnel: [w2759 w2780] -> w2757
              tunnel: [w2758 w2779] -> w2756
              tunnel: w2755 -> [_ w2760]
              tunnel: w2753 -> [w2759 w2778]
              tunnel: w2752 -> [w2758 w2777]
              frame False {
              }
              frame True {
                w2773 = ""
                # "If number of mixtures > 0 then send CM,D command to delete last mixture entry."
                n791 = call "Process Compose Mixture Command (SubVI).vi"("Argument#4"=w2773, "Argument#2"=w2773, "Argument#1"="D", "Address"=w2760, "error in (no error)"=w2777, "Argument#3"=w2773, "VISA Refnum in"=w2778) -> ("error out"=w2775:errorcluster, "CM Output String"=w2765:string, "VISA Refnum out"=w2776:refnum<visa-resource-name>)  [unwired: 2 in]
                n792 = Decimal String To Number(string=w2765) -> (number=w2771:i32)  [unwired: 2 in, 1 out]
                n793 = Greater Or Equal?(x=w2771, y=200) -> (x >= y?=w2768:bool)
                n794 = Less?(x=w2771, y=220) -> (x < y?=w2769:bool)
                n795 = And(x=w2768, y=w2769) -> (x .and. y?=w2767:bool)
                n796 = Concatenate Strings("Mixture #", w2765, " has been deleted!") -> (w2763:string)
                n797 = Select(t=w2763, s=w2767, f=" Error in Deleting Mixture!") -> (s? t:f=w2761:string)
                n798 = property on="Completion\ntext" class="Str"("Value"=w2761) -> ()  [unwired: 2 in, 2 out]
                n799 = case shown="No Error" w2775 {
                  selector: w2775 -> [w2789 w2797]
                  tunnel: w2776 -> [w2792 w2798]
                  tunnel: [w2795 w2798] -> w2780
                  tunnel: [w2794 w2797] -> w2779
                  tunnel: w2760 -> [w2787 _]
                  frame No Error {
                    w2793 = ""
                    # "Update Mixture number index\nto be used for new mixture."
                    # "Update Select Gas combo box."
                    n800 = call "Process Compose Mixture Command (SubVI).vi"("Argument#4"=w2793, "Argument#2"=w2793, "Argument#1"=w2793, "Address"=w2787, "error in (no error)"=w2789, "Argument#3"=w2793, "VISA Refnum in"=w2792) -> ("error out"=w2790:errorcluster, "CM Output String"=w2788:string, "VISA Refnum out"=w2791:refnum<visa-resource-name>)  [unwired: 2 in]
                    n801 = Decimal String To Number(string=w2788) -> (number=w2783:i32)  [unwired: 2 in, 1 out]
                    n802 = To Unsigned Word Integer(number=w2783) -> (unsigned 16bit integer=w2781:u16)
                    n803 = Add(x=w2781, y=u16 200) -> (x+y=w2782:u16)
                    n804 = call "Init Gas Combo (SubVI).vi"("name or relative path"="GasTable.txt") -> ("Array"=w2785:cluster{"String":string, "Value":string}[])  [unwired: 10 in]
                    n805 = property on="Mix. #" class="DigNum (strict)"("Value"=w2782) -> ()  [unwired: 2 in, 2 out]
                    n806 = call "Update Gas Combo with GM (SubVI).vi"("VISA Refnum in"=w2791, "Array In"=w2785, "Number of Mixtures"=w2781, "error in (no error)"=w2790, "Address String"=w2787) -> ("VISA Refnum out"=w2795:refnum<visa-resource-name>, "Array Out"=w2796:cluster{"String":string, "Value":string}[], "error out"=w2794:errorcluster)  [unwired: 3 in]
                    n807 = global write "Global.vi" "GM Number"(w2781) -> ()
                    n808 = property on="Selected Gas" class="CmbBox"("Strings And Values[]"=w2796) -> ()  [unwired: 2 in, 2 out]
                  }
                  frame Error {
                  }
                }
              }
            }
          }
        }
        n809 = Select(t=0, s=w2727, f=w2747) -> (s? t:f=w2748:i32)
      }
      event "PI Logging Options.Log Data": Value Change {
        # "Close current data file"
        # "Reset if\ncomm error"
        # "Closes previously opened file (if applicable), opens a new one, and checks to make sure that the communication to the unit is still established"
        n810 = event-data() -> ()  [unwired: 1 in, 1 out]
        n811 = property on="Mass Flow Units" class="CmbBox"() -> ("Value"=w2817:string)  [unwired: 2 in, 2 out]
        n812 = property on="Vol. Flow Units" class="CmbBox"() -> ("Value"=w2816:string)  [unwired: 2 in, 2 out]
        n813 = case shown="True" w2828 {
          tunnel: w2827 -> [_ w2868]
          tunnel: w2829 -> [w2865 w2867]
          tunnel: [w2865 w2866] -> w2826
          frame False {
          }
          frame True {
            n814 = Close File(refnum=w2868, error in=w2867) -> (error out=w2866:errorcluster)  [unwired: 1 out]
          }
        }
        n815 = property on="Temperature Units" class="CmbBox"() -> ("Value"=w2813:string)  [unwired: 2 in, 2 out]
        n816 = property on="Pressure Units" class="CmbBox"() -> ("Value"=w2812:string)  [unwired: 2 in, 2 out]
        n817 = Unbundle By Name(w2802) -> ("Serial Number"=w2811:string)
        n818 = call "Convert Mass Flow EU to Totalizer EU (SubVI).vi"("Mass Flow EU"=w2817) -> ("Totalizer EU"=w2814:string)  [unwired: 10 in]
        n819 = Concatenate Strings(w2811, "_" ("string")) -> (w2809:string)
        n820 = Bundle(cluster=T23 {"Mass Flow"="", "Valve Counts"="", "Volumetric Flow"="", "Totalizer"="", "Temperature"="", "Pressure"=""} ("Units of Measure Input"), "Mass Flow"=w2817, "Valve Counts"="%FS  Counts", "Volumetric Flow"=w2816, "Totalizer"=w2814, "Temperature"=w2813, "Pressure"=w2812) -> (w2807:T23)
        n821 = Unbundle By Name("PI Logging Options") -> ("Log Data"=w2808:bool)
        n822 = case shown="True" w2808 {
          tunnel: ["" w2854] -> w2825
          tunnel: w2809 -> [_ w2853]
          frame False {
          }
          frame True {
            n823 = Get Date/Time In Seconds() -> (seconds since 1Jan1904=w2862:timestamp)
            n824 = Format Date/Time String(time format string (%c)="%m-%d-%Y_%H-%M-%S", seconds (now)=w2862) -> (date/time string=w2861:string)  [unwired: 1 in]
            n825 = call <vilib>:"Application Directory.vi"() -> ("Application Directory"=w2858:path)
            n826 = Format Date/Time String(time format string (%c)="%p", seconds (now)=w2862) -> (date/time string=w2860:string)  [unwired: 1 in]
            n827 = Path To String(path=w2858) -> (string=w2856:string)
            n828 = Concatenate Strings(w2856, "\\PI Data Log_" ("string"), w2853, w2861, "_" ("string"), w2860, ".txt" ("string")) -> (w2854:string)
          }
        }
        n829 = call "Data Log Make Header.vi"("PI Logging Options"="PI Logging Options", "error in"=w2826, "Units of Measure Input"=w2807) -> ("error out"=w2823:errorcluster, "Data Log Header"=w2805:string)  [unwired: 7 in]
        n830 = String To Path(string=w2825) -> (path=w2824:path)
        n831 = case shown="True" w2808 {
          tunnel: [w2842 w2849] -> w2822
          tunnel: w2823 -> [w2842 w2844]
          tunnel: w2805 -> [_ w2848]
          tunnel: w2824 -> [_ w2847]
          tunnel: T22."replace or create" ("operation (0:open)") -> [_ w2846]
          tunnel: [refnum<file> refnum ("refnum out") w2845] -> w2803
          frame False {
          }
          frame True {
            n832 = Open/Create/Replace File(file path (use dialog)=w2847, error in=w2844, operation (0:open)=w2846) -> (refnum out=w2851:refnum<file>, error out=w2850:errorcluster)  [unwired: 3 in, 1 out]
            n833 = Write to Text File(file (use dialog)=w2851, text=w2848, error in=w2850) -> (refnum out=w2845:refnum<file>, error out=w2849:errorcluster)  [unwired: 1 in, 1 out]
          }
        }
        n834 = Select(t=0, s=w2822, f=w2819) -> (s? t:f=w2840:i32)
      }
    }
    n835 = case shown="True" w66 {
      selector: w66 -> [w111 _]
      tunnel: [w111 FALSE] -> w67
      tunnel: w61 -> [_ w130]
      tunnel: w63 -> [_ w118]
      tunnel: w62 -> [_ w117]
      tunnel: w61 -> [_ w116]
      tunnel: w53 -> [w110 w115]
      tunnel: [w110 w114] -> w60
      tunnel: w59 -> [w109 w113]
      tunnel: [w109 w112] -> w58
      frame False {
      }
      frame True {
        n836 = case shown="True" w118 {
          tunnel: w117 -> [_ w146]
          tunnel: w116 -> [_ w141]
          tunnel: w115 -> [w134 w138]
          tunnel: [w134 w137] -> w114
          tunnel: w113 -> [w133 w136]
          tunnel: [w133 w135] -> w112
          frame False {
          }
          frame True {
            n837 = Unbundle By Name(w146) -> ("Selected Gas"=w145:string)
            n838 = local read "PI Logging Options"() -> (w143:T3)
            n839 = Match Pattern(string=w145, regular expression=",") -> (after substring=w142:string)  [unwired: 1 in, 3 out]
            n840 = call "PI Logg Make Data String.vi"("PI Logging Options"=w143, "error in"=w138, "Process Information"=w141, "Selected Gas"=w142) -> ("error out"=w139:errorcluster, "Data Log String"=w140:string)  [unwired: 5 in, 1 out]
            n841 = Write to Text File(file (use dialog)=w136, text=w140, error in=w139) -> (refnum out=w135:refnum<file>, error out=w137:errorcluster)  [unwired: 1 in, 1 out]
          }
        }
        n842 = Unbundle By Name(w130) -> ("Mass Flow"=w129:string, "Volum. Flow"=w128:string, "Set Point"=w127:string, "Gas Temp."=w126:string, "Gas Pressure"=w125:string)
        n843 = Fract/Exp String To Number(string=w127) -> (number=w122:dbl)  [unwired: 3 in, 1 out]
        n844 = Fract/Exp String To Number(string=w126) -> (number=w121:dbl)  [unwired: 3 in, 1 out]
        n845 = Fract/Exp String To Number(string=w125) -> (number=w120:dbl)  [unwired: 3 in, 1 out]
        n846 = Fract/Exp String To Number(string=w129) -> (number=w124:dbl)  [unwired: 3 in, 1 out]
        n847 = Fract/Exp String To Number(string=w128) -> (number=w123:dbl)  [unwired: 3 in, 1 out]
        n848 = Bundle(w124, w123, w122, w121, w120) -> (w119:cluster{dbl, dbl, dbl, dbl, dbl})  [unwired: 1 in]
        n849 = case shown="True" "Chart: Enable Graphic" {
          tunnel: w119 -> [_ w147]
          frame False {
          }
          frame True {
            "Chart" <- w147
          }
        }
      }
    }
    n850 = Or(x="stop", y=w86) -> (x .or. y?=w85:bool)
    n851 = Select(t=w53, s=w53, f=w93) -> (s? t:f=w94:errorcluster)
    n852 = Select(t=50, s=w53, f=0) -> (s? t:f=w95:i32)
  }
  n853 = VISA Close(VISA resource name=w30, error in (no error)=w29) -> (error out=w35:errorcluster)
  n854 = Unbundle(w31) -> (w33:refnum<vi>, "Panel"=w32:refnum<vi>)
  n855 = case shown="True" w4 {
    tunnel: w5 -> [_ w2869]
    frame False {
    }
    frame True {
      # "Currently logging"
      n856 = Close File(refnum=w2869) -> ()  [unwired: 1 in, 2 out]
    }
  }
  n857 = Close Reference(reference=w33, error in (no error)=w35) -> (error out=w36:errorcluster)
  n858 = Close Reference(reference=w32, error in (no error)=w36) -> (error out=w34:errorcluster)
  n859 = call <vilib>:"Simple Error Handler.vi"("error in (no error)"=w34) -> ("error out"=→"error out":errorcluster)  [unwired: 4 in, 4 out]
